vi "Elevator.vi"() -> ()   [LabVIEW 2018]
uses:
  Elevator Cabin.ctl
  Floors Schematic.ctl
  Elevator Panel.ctl
  Elevator Automate.ctl
  Elevator Command.ctl
  Elevator Constants.ctl
panel:
  out "Delay Timer":i32
  out "Passenger Information Board":string="Этаж 1\r\nОстановка"
  out "# elements in Elevator Command Queue":i32
  out "Global Wait in ms":u32=10
  out "# elements in Elevator Floor Queue":i32
  out "Position:Top":i32=585
  out "Elevator Floor Queue":u8[](array[numeric])
  out "Elevator Command Queue":T1[](array[typedef])
  in  "Elevator Automate":T2={"Elevator Panel Array"=[FALSE, FALSE, FALSE, FALSE, FALSE, FALSE, FALSE, FALSE, FALSE, FALSE, FALSE, FALSE], "Floor Array"=[FALSE, FALSE, FALSE, FALSE, FALSE, FALSE, FALSE, FALSE, FALSE, FALSE, FALSE, FALSE], "Elevator Command"=enum."Open Doors", "Target Floor"=0, "Forced Stop"=FALSE, "Cancel Delay"=FALSE, "Elevator Status"=enum."Stand By", "Update\nTarget Floor"=FALSE, "Take a Call"=FALSE, "Add Floor\nto Queue"=FALSE}
  in  "Elevator Panel":T3
  in  "Floors Schematic":T4={"Call 1"=FALSE, "Call 2"=FALSE, "Call 3"=FALSE, "Call 4"=FALSE, "Call 5"=FALSE, "Call 6"=FALSE, "Call 7"=FALSE, "Call 8"=FALSE, "Call 9"=FALSE, "Call 10"=FALSE, "Call 11"=FALSE, "Call 12"=FALSE, "Floor Position"=[0, 0, 0, 0, 0, 0, 0, 0, 0, 0, 0, 0]}
  in  "STOP":bool
  out "Elevator Cabin":T5 scale=0.0..100.0
  # "Краткая информация об автомате лифта\n\nЕсть две очереди: очередь команд лифта (Elevator Command Queue) и очередь вызовов этажей лифта (Elevator Floor Queue).\n\nАвтомат при вызове этажа обрабатывает и перестраивает очередь с учетом приоритета вызовов.\n\nАвтомат принимает решения исходя из этажа-цели (Target Floor), текущей выполняющейся команды (Elevator Command) и статуса состояния лифта (Elevator Status).\n\nАвтомат имеет хранилище вызовов этажей из кабины лифта (Elevator Panel Array) и вызовов с этажей дома (Floor Array).\n\nКоманды Elevator Command:\n1) Idle - команда ожидания;\n2) Short Delay - короткая задержка (2 сек);\n3) Long Delay - длинная задержка (6 сек);\n4) Cancel Delay - задержка в случае отмены вызова и принятия решений обработки следующего вызова (6 сек или 15 сек в зависимости от состояний автомата лифта);\n5) Open Doors - открыть двери кабины лифта;\n6) Close Doors - закрыть двери кабины лифта;\n7) Going Up - движение вверх к этажу-цели;\n8) Going Down - движение вниз к этажу-цели;\n9) Unpress Button отжать кнопки на этаже-цели.\n\nСостояния Elevator Status:\n1) Stand By - состояние остановки кабины лифта и ожидания вызова;\n2) Stop - состояние остановки кабины лифта при движении вверх или вниз;\n3) Going Up - состояние движения вверх к этажу-цели;\n4) Going Down - состояние движения вниз к этажу-цели;\n5) Cancel - состояние отмены текущих вызовов панели кабины лифта.\n\nКнопки Автомата для обработки событий:\n1) Take a Call - обработать следующий вызов из очереди;\n2) Add Floor to Queue - добавить этаж в очередь вызовов;\n3) Update Target Floor - обновить этаж-цель;\n4) Forced Stop - прерывание исполняемой команды лифта;\n5) Cancel Delay - обработка события отмены вызовов панели кабины лифта."
  # "Симулятор работы лифта в двенадцатиэтажном доме\n\nВ симуляторе имеются:\n1) кнопки вызова (1-12) на этажах дома (Floors Schematic);\n2) кнопки вызова (1-12) панели кабины лифта (Elevator Panel);\n3) кнопка отмены всех вызовов панели кабины лифта (Cancel);\n4) кнопка вызова оператора (Emergency);\n5) кнопка закрытия дверей (>||<);\n6) кнопка открытия дверей (<||>);\n7) Информационное табло лифта (Passenger Information Board).\n\nКнопки вызова на этажах дома являются вызовом по направлению движения кабины лифта вниз.\n\nПриоритет этажей построен так, чтобы обработать максимально возможное количество вызовов при заданном направлении движения кабины лифта.\n\nОчередь вызовов выстраивается с учетом направления движения кабины лифта, вызова на этаж из кабины лифта и вызова на этаж дома (приведено в поряжке убывания приоритета).\n\nНачальное состояние работы симулятора:\nкабина лифта на первом этаже, двери кабины лифта закрыты, все кнопки вызова отжаты.\n\nТабло лифта приводит информацию о текущем этаже, статусе движения кабины лифта (движение вверх, движение вниз, остановка), а также сигнализирует о работе кнопки вызова оператора.\n\nЕсли лифт приезжает на обработанный с учетом очереди этаж-цель (Targer Floor), кнопка вызова этажа-цели отжимаются как в кабине лифта, так и на этаже дома.\n\nДвери кабины лифта не откроются при движении лифта вверх или вниз. Лифт открывает двери повторно, если двери кабины лифта не закрыты на этаже-цели. Лифт не закроет двери, пока не закончится открытие дверей."
  # "12"
  # "11"
  # "10"
  # "9"
  # "8"
  # "7"
  # "6"
  # "5"
  # "4"
  # "3"
  # "2"
  # "1"
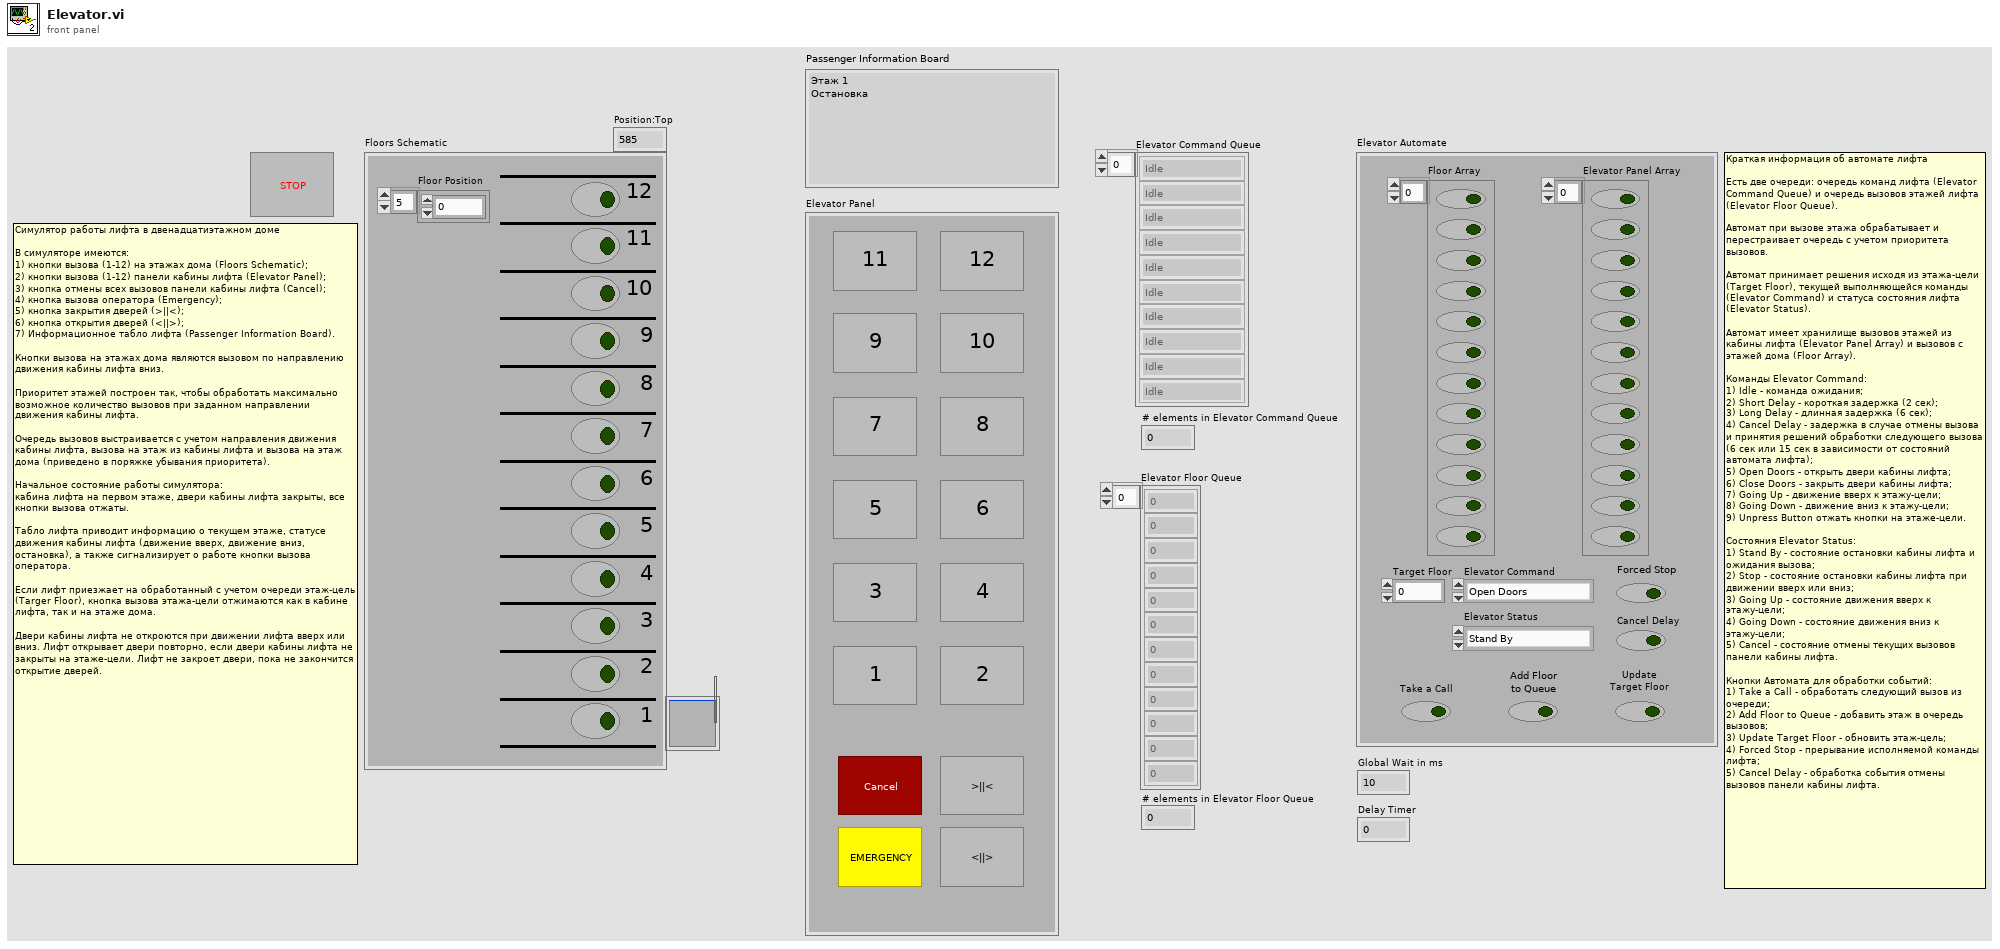
[diagram p1: front panel]
types:
  T1 = typedef "Elevator Command.ctl" = enum16{"Idle", "Short Delay", "Long Delay", "Cancel Delay", "Open Doors", "Close Doors", "Going Up", "Going Down", "Unpress Button"}
  T2 = typedef "Elevator Automate.ctl" = cluster{"Elevator Panel Array":bool[], "Floor Array":bool[], "Elevator Command":T1, "Target Floor":u8, "Forced Stop":bool, "Cancel Delay":bool, "Elevator Status":enum16{"Stand By", "Stop", "Going Up", "Going Down", "Cancel"}, "Update\nTarget Floor":bool, "Take a Call":bool, "Add Floor\nto Queue":bool}
  T3 = typedef "Elevator Panel.ctl" = cluster{"Open Doors":bool, "Close Doors":bool, "Floor 2":bool, "Floor 1":bool, "Floor 3":bool, "Floor 4":bool, "Floor 5":bool, "Floor 6":bool, "Floor 7":bool, "Floor 8":bool, "Floor 9":bool, "Floor 10":bool, "Floor 11":bool, "Floor 12":bool, "Emergency":bool, "Cancel":bool}
  T4 = typedef "Floors Schematic.ctl" = cluster{"Call 1":bool, "Call 2":bool, "Call 3":bool, "Call 4":bool, "Call 5":bool, "Call 6":bool, "Call 7":bool, "Call 8":bool, "Call 9":bool, "Call 10":bool, "Call 11":bool, "Call 12":bool, "Floor Position":i16[]}
  T5 = typedef "Elevator Cabin.ctl" = u8
  T6 = enum16{"Stand By", "Stop", "Going Up", "Going Down", "Cancel"}
  T7 = enum8{"Enabled", "Disabled", "Disabled and Grayed Out"}
  T8 = typedef "Elevator Constants.ctl" = u8
  T9 = enum16{"Stand By", "Stop", "Going Up", "Going Down"}
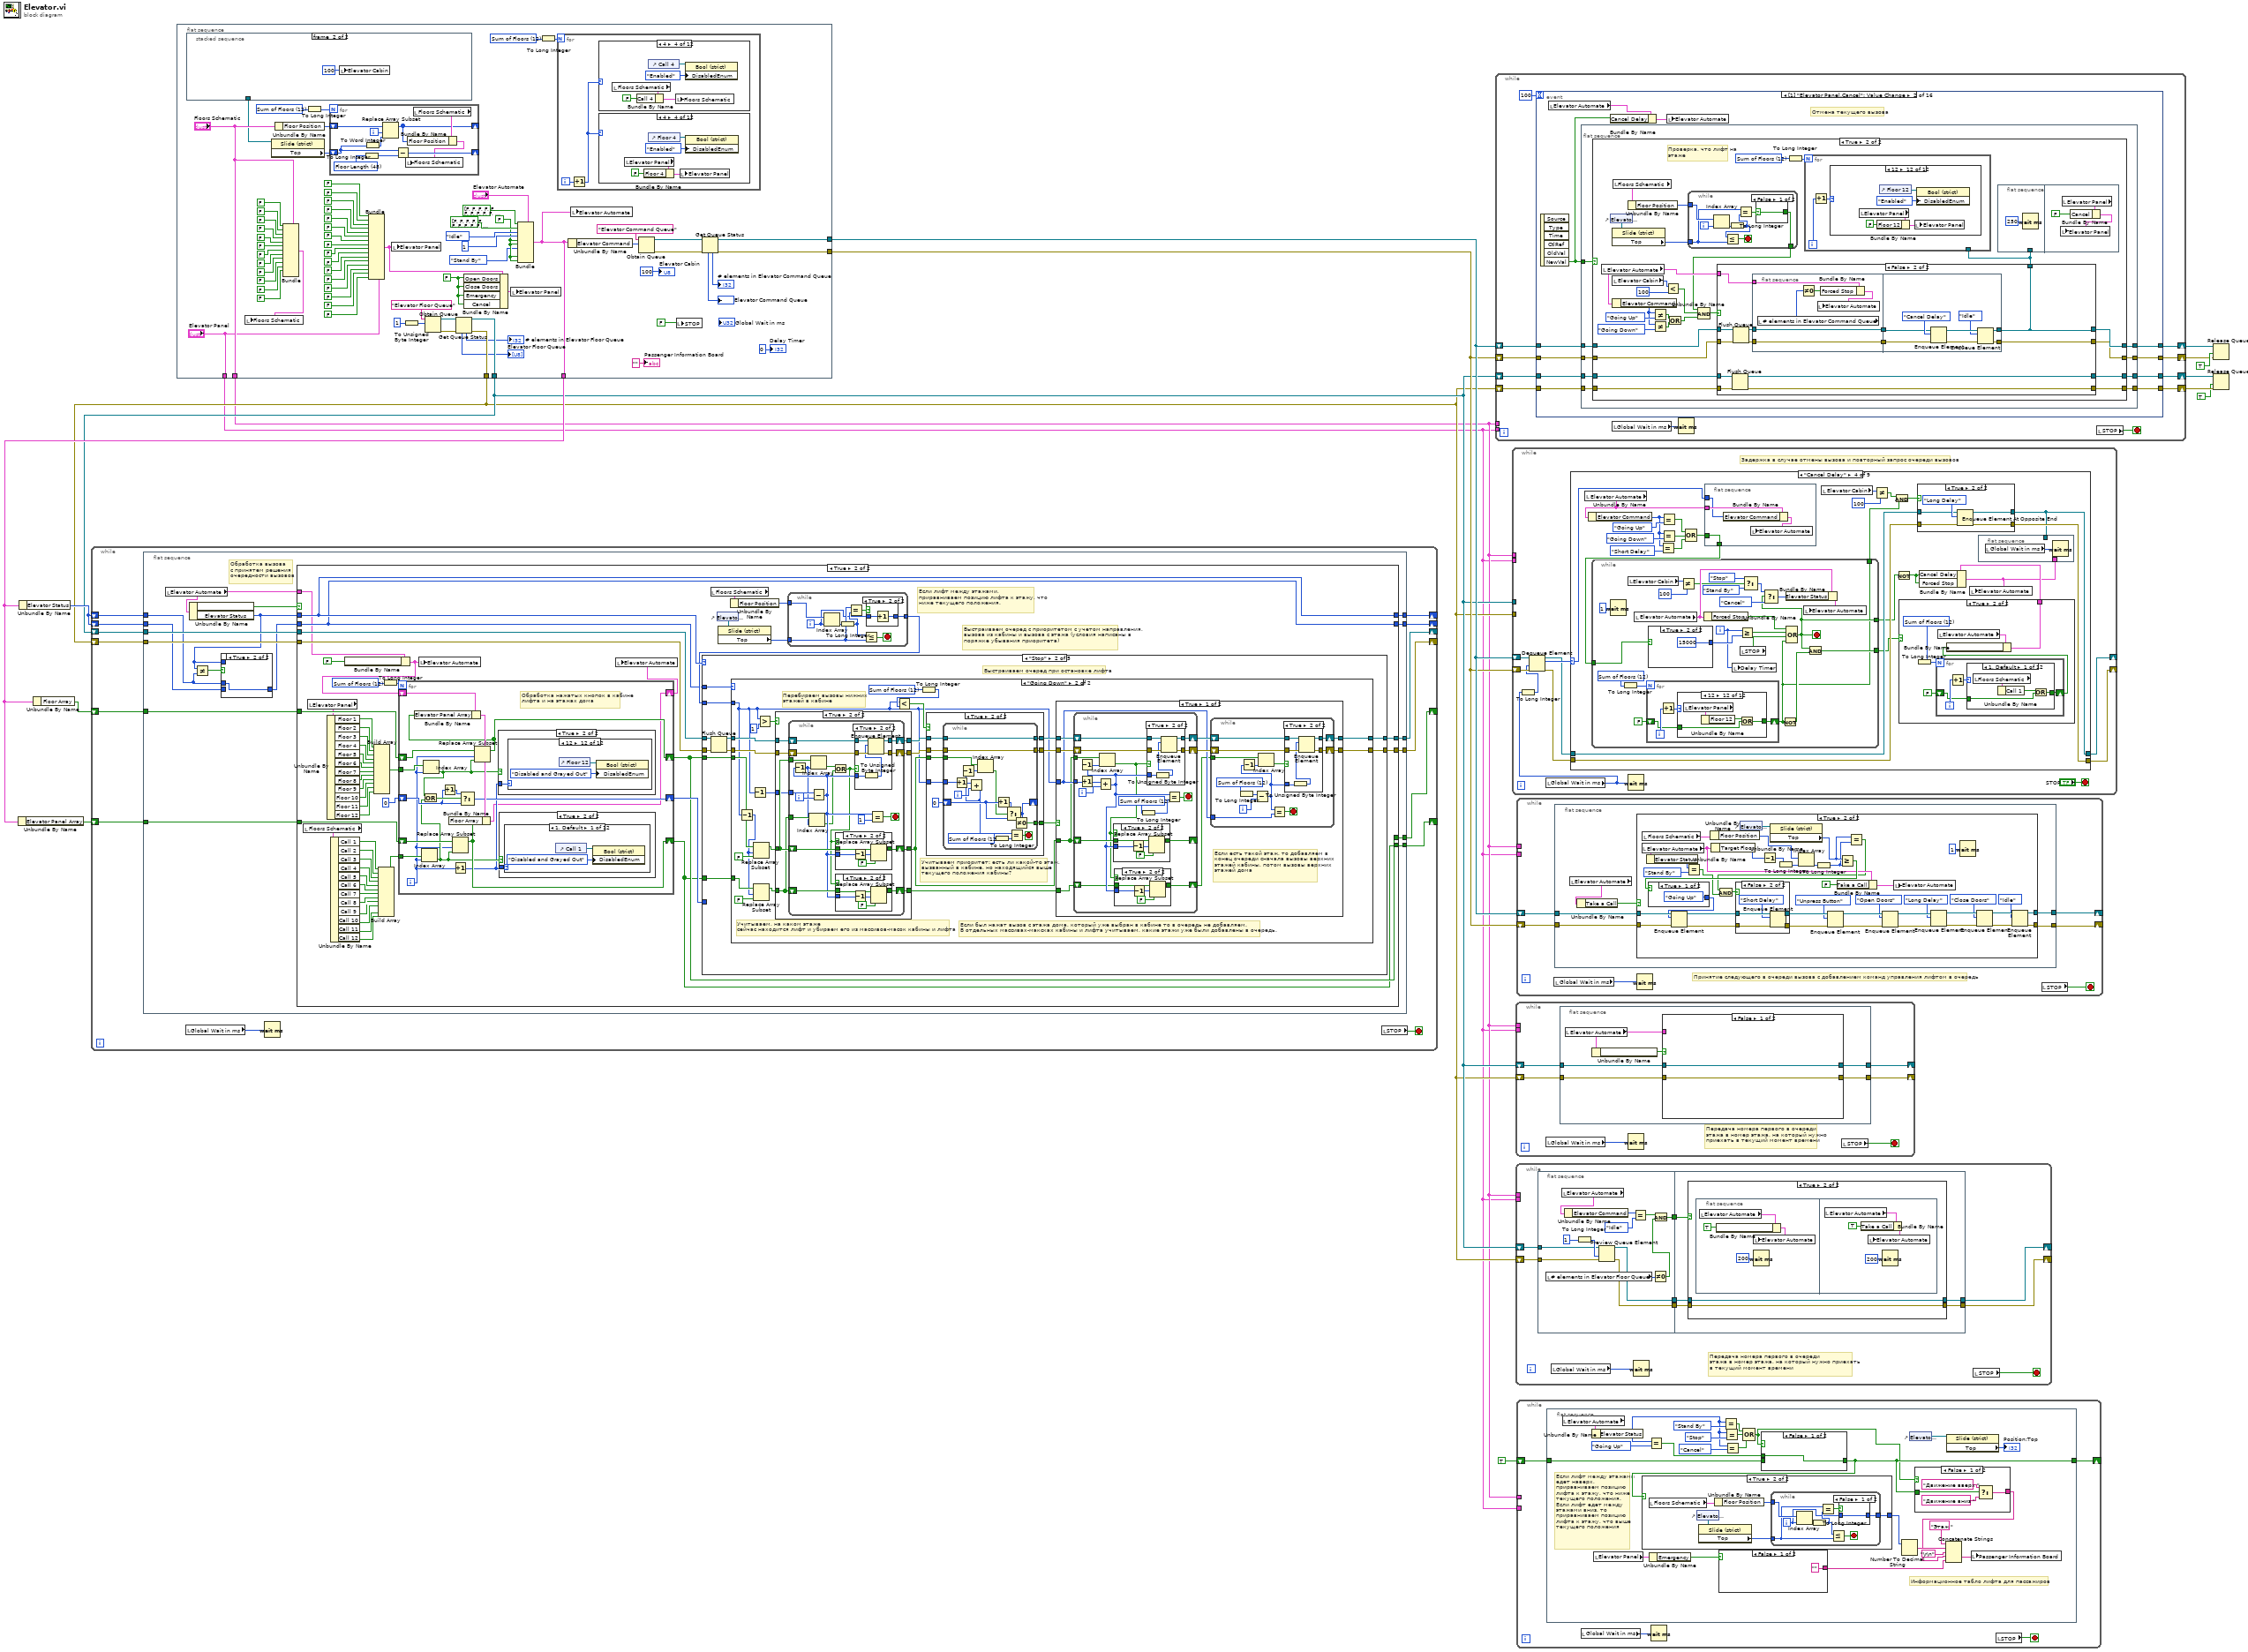
[diagram p0: block diagram]
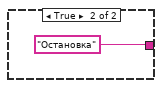
[diagram p2: hidden frame]
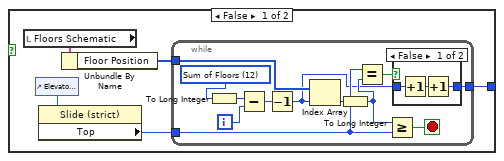
[diagram p4: hidden frame]
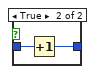
[diagram p5: hidden frame]
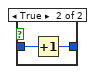
[diagram p6: hidden frame]
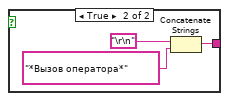
[diagram p7: hidden frame]
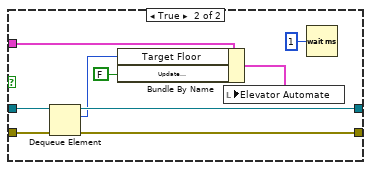
[diagram p9: hidden frame]
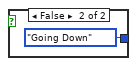
[diagram p12: hidden frame]
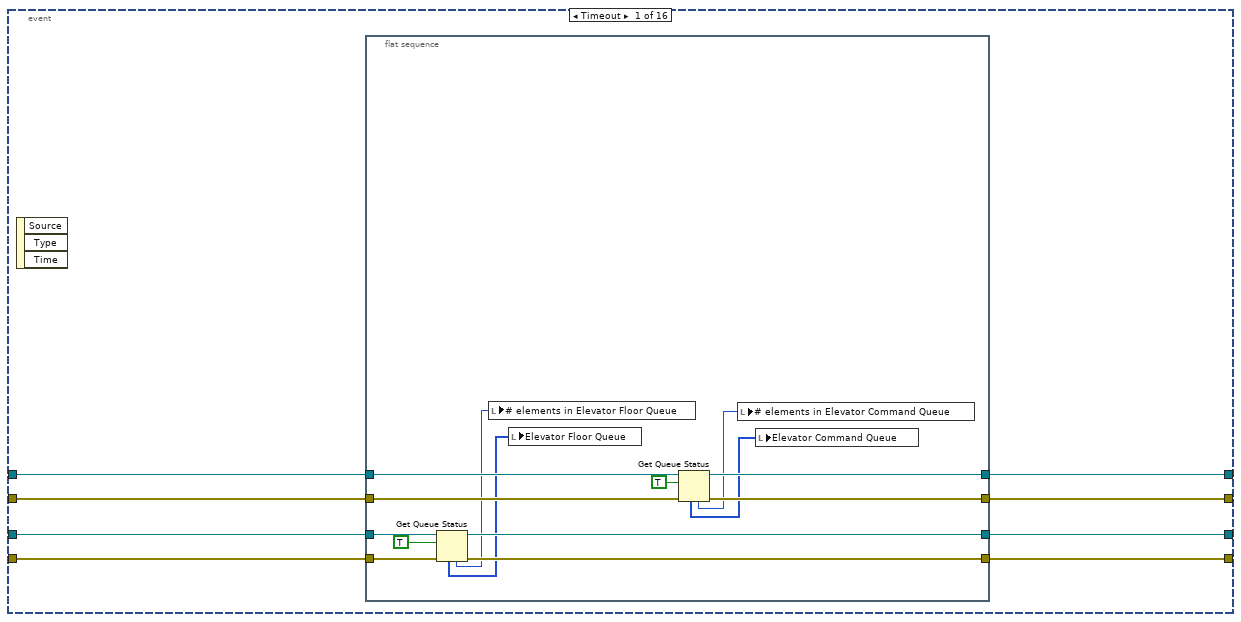
[diagram p13: hidden frame]
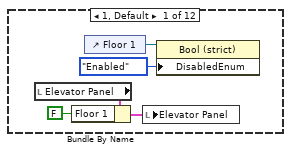
[diagram p15: hidden frame]
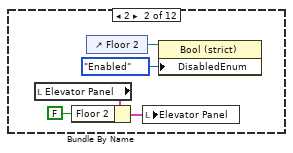
[diagram p16: hidden frame]
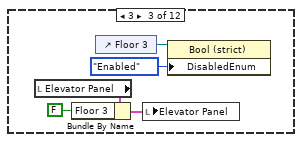
[diagram p17: hidden frame]
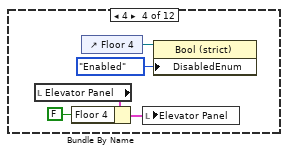
[diagram p18: hidden frame]
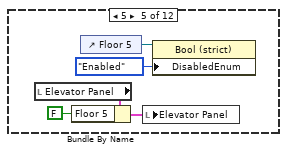
[diagram p19: hidden frame]
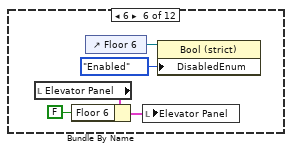
[diagram p20: hidden frame]
diagram:
  n1 = Unbundle By Name(w9) -> ("Elevator Panel Array"=w16:bool[])
  n2 = Unbundle By Name(w9) -> ("Elevator Status"=w8:T6)
  n3 = Unbundle By Name(w9) -> ("Floor Array"=w17:bool[])
  n4 = while {
    shift-right: [w26] -> _
    shift-left: w16 -> [w29]
    shift-right: [w25] -> _
    shift-left: w17 -> [w30]
    shift-right: [w23] -> _
    shift-left: w4 -> [w28]
    shift-right: [w24] -> _
    shift-left: w5 -> [w27]
    shift-right: [w22] -> _
    shift-left: w8 -> [w19]
    shift-right: [w20] -> _
    shift-left: w8 -> [w21]
    stop <- w31 stop-if-true
    n5 = flat-sequence {
      tunnel: [w43] -> w26
      tunnel: [w42] -> w25
      tunnel: [w41] -> w24
      tunnel: [w40] -> w23
      tunnel: [w39] -> w22
      tunnel: [w34] -> w20
      tunnel: w30 -> [w48]
      tunnel: w29 -> [w47]
      tunnel: w28 -> [w46]
      tunnel: w27 -> [w45]
      tunnel: w21 -> [w36]
      tunnel: w19 -> [w33]
      frame #0 {
        # "Обработка вызова\nс принятем решения\nочередности вызовов"
        n6 = local read "Elevator Automate"() -> (w38:T2)
        n7 = Unbundle By Name(w38) -> ("Add Floor\nto Queue"=w44:bool, "Elevator Status"=w35:T6)
        n8 = Not Equal?(x=w35, y=w36) -> (x != y?=w37:bool)
        n9 = case shown="True" w37 {
          tunnel: w35 -> [_ _]
          tunnel: w36 -> [_ w50]
          tunnel: w33 -> [w49 _]
          tunnel: [w49 w50] -> w32
          frame False {
          }
          frame True {
          }
        }
        n10 = case shown="True" w44 {
          tunnel: w48 -> [w53 w107]
          tunnel: w47 -> [w54 w106]
          tunnel: w46 -> [w55 w75]
          tunnel: w45 -> [w56 w74]
          tunnel: w35 -> [w52 w70]
          tunnel: [w56 w72] -> w41
          tunnel: [w55 w71] -> w40
          tunnel: [w54 w65] -> w43
          tunnel: [w53 w66] -> w42
          tunnel: w32 -> [w51 w64]
          tunnel: [w51 w64] -> w39
          tunnel: w38 -> [_ w59]
          tunnel: [w52 w70] -> w34
          frame False {
          }
          frame True {
            w77 = T8 12 items=["Floor Length"=48, "Sum of Floors"=12, "Floor Step in ms"=63, "Elevator Door Step in ms"=30, "Global Wait in ms"=20, "Event Wait in ms"=100] ("Elevator Constants")
            # "Выстраиваем очеред с приоритетом с учетом направления, вызова из кабины и вызова с этажа (условия написаны в поряжке убывания приоритета)"
            # "Если лифт между этажами,\nприравниваем позицию лифта к этажу, что ниже текущего положения."
            n11 = local read "Floors Schematic"() -> (w78:T4)
            n12 = local read "Elevator Panel"() -> (w79:T3)
            n13 = Unbundle By Name(w79) -> ("Floor 1"=w105:bool, "Floor 2"=w104:bool, "Floor 3"=w103:bool, "Floor 4"=w102:bool, "Floor 5"=w101:bool, "Floor 6"=w100:bool, "Floor 7"=w99:bool, "Floor 8"=w98:bool, "Floor 9"=w97:bool, "Floor 10"=w96:bool, "Floor 11"=w95:bool, "Floor 12"=w94:bool)
            n14 = Unbundle By Name(w78) -> ("Call 1"=w80:bool, "Call 2"=w92:bool, "Call 3"=w91:bool, "Call 4"=w90:bool, "Call 5"=w89:bool, "Call 6"=w88:bool, "Call 7"=w87:bool, "Call 8"=w86:bool, "Call 9"=w85:bool, "Call 10"=w84:bool, "Call 11"=w83:bool, "Call 12"=w82:bool)
            n15 = Bundle By Name(cluster=w59, "Add Floor\nto Queue"=FALSE ("Add Floor to Queue")) -> (w58:T2)
            n16 = Build Array(w105, w104, w103, w102, w101, w100, w99, w98, w97, w96, w95, w94) -> (w93:bool[])
            n17 = Build Array(w80, w92, w91, w90, w89, w88, w87, w86, w85, w84, w83, w82) -> (w81:bool[])
            n18 = To Long Integer(number=w77) -> (32bit integer=w76:i32)
            n19 = for {
              N: w76 -> [_]
              tunnel: w93 -> [w1124]
              tunnel: w81 -> [w1123]
              shift-right: [w1114] -> w65
              shift-left: w106 -> [w1120]
              shift-right: [w1115] -> w66
              shift-left: w107 -> [w1121]
              shift-right: [w1117] -> w69
              shift-left: 0 -> [w1116]
              shift-right: [w1108] -> w57
              shift-left: w58 -> [w1109]
              i -> [w1111]
              # "Обработка нажатых кнопок в кабине лифта и на этажах дома"
              n20 = Index Array(array=w1123, index=w1111) -> (element=w1113:bool)
              n21 = Index Array(array=w1124, index=w1111) -> (element=w1112:bool)
              n22 = Or(x=w1112, y=w1113) -> (x .or. y?=w1119:bool)
              n23 = Increment(x=w1116) -> (x+1=w1118:i32)
              n24 = Replace Array Subset(array=w1120, new element=w1113, index=w1111) -> (w1114:bool[])
              n25 = Increment(x=w1111) -> (x+1=w1110:i32)
              n26 = Select(t=w1118, s=w1119, f=w1116) -> (s? t:f=w1117:i32)
              n27 = Replace Array Subset(array=w1121, new element=w1112, index=w1111) -> (w1115:bool[])
              n28 = Bundle By Name(cluster=w1109, "Elevator Panel Array"=w1115) -> (w1122:T2)
              n29 = Bundle By Name(cluster=w1122, "Floor Array"=w1114) -> (w1108:T2)
              n30 = case shown="True" w1112 {
                tunnel: w1110 -> [_ w1150]
                frame False {
                }
                frame True {
                  n31 = case shown="12" w1150 {
                    frame 1, Default {
                      n32 = control-ref of="Floor 1"() -> (w1152:refnum<vi>)
                      n33 = property class="Bool (strict)"(reference=w1152, "DisabledEnum"=T7."Disabled and Grayed Out" ("Disabled")) -> ()  [unwired: 1 in, 2 out]
                    }
                    frame 2 {
                      n34 = control-ref of="Floor 2"() -> (w1154:refnum<vi>)
                      n35 = property class="Bool (strict)"(reference=w1154, "DisabledEnum"=T7."Disabled and Grayed Out" ("Disabled")) -> ()  [unwired: 1 in, 2 out]
                    }
                    frame 3 {
                      n36 = control-ref of="Floor 3"() -> (w1156:refnum<vi>)
                      n37 = property class="Bool (strict)"(reference=w1156, "DisabledEnum"=T7."Disabled and Grayed Out" ("Disabled")) -> ()  [unwired: 1 in, 2 out]
                    }
                    frame 4 {
                      n38 = control-ref of="Floor 4"() -> (w1158:refnum<vi>)
                      n39 = property class="Bool (strict)"(reference=w1158, "DisabledEnum"=T7."Disabled and Grayed Out" ("Disabled")) -> ()  [unwired: 1 in, 2 out]
                    }
                    frame 5 {
                      n40 = control-ref of="Floor 5"() -> (w1160:refnum<vi>)
                      n41 = property class="Bool (strict)"(reference=w1160, "DisabledEnum"=T7."Disabled and Grayed Out" ("Disabled")) -> ()  [unwired: 1 in, 2 out]
                    }
                    frame 6 {
                      n42 = control-ref of="Floor 6"() -> (w1162:refnum<vi>)
                      n43 = property class="Bool (strict)"(reference=w1162, "DisabledEnum"=T7."Disabled and Grayed Out" ("Disabled")) -> ()  [unwired: 1 in, 2 out]
                    }
                    frame 7 {
                      n44 = control-ref of="Floor 7"() -> (w1164:refnum<vi>)
                      n45 = property class="Bool (strict)"(reference=w1164, "DisabledEnum"=T7."Disabled and Grayed Out" ("Disabled")) -> ()  [unwired: 1 in, 2 out]
                    }
                    frame 8 {
                      n46 = control-ref of="Floor 8"() -> (w1166:refnum<vi>)
                      n47 = property class="Bool (strict)"(reference=w1166, "DisabledEnum"=T7."Disabled and Grayed Out" ("Disabled")) -> ()  [unwired: 1 in, 2 out]
                    }
                    frame 9 {
                      n48 = control-ref of="Floor 9"() -> (w1168:refnum<vi>)
                      n49 = property class="Bool (strict)"(reference=w1168, "DisabledEnum"=T7."Disabled and Grayed Out" ("Disabled")) -> ()  [unwired: 1 in, 2 out]
                    }
                    frame 10 {
                      n50 = control-ref of="Floor 10"() -> (w1170:refnum<vi>)
                      n51 = property class="Bool (strict)"(reference=w1170, "DisabledEnum"=T7."Disabled and Grayed Out" ("Disabled")) -> ()  [unwired: 1 in, 2 out]
                    }
                    frame 11 {
                      n52 = control-ref of="Floor 11"() -> (w1172:refnum<vi>)
                      n53 = property class="Bool (strict)"(reference=w1172, "DisabledEnum"=T7."Disabled and Grayed Out" ("Disabled")) -> ()  [unwired: 1 in, 2 out]
                    }
                    frame 12 {
                      n54 = control-ref of="Floor 12"() -> (w1174:refnum<vi>)
                      n55 = property class="Bool (strict)"(reference=w1174, "DisabledEnum"=T7."Disabled and Grayed Out" ("Disabled")) -> ()  [unwired: 1 in, 2 out]
                    }
                  }
                }
              }
              n56 = case shown="True" w1113 {
                tunnel: w1110 -> [_ w1125]
                frame False {
                }
                frame True {
                  n57 = case shown="1, Default" w1125 {
                    frame 1, Default {
                      n58 = control-ref of="Call 1"() -> (w1127:refnum<vi>)
                      n59 = property class="Bool (strict)"(reference=w1127, "DisabledEnum"=T7."Disabled and Grayed Out" ("Disabled")) -> ()  [unwired: 1 in, 2 out]
                    }
                    frame 2 {
                      n60 = control-ref of="Call 2"() -> (w1129:refnum<vi>)
                      n61 = property class="Bool (strict)"(reference=w1129, "DisabledEnum"=T7."Disabled and Grayed Out" ("Disabled")) -> ()  [unwired: 1 in, 2 out]
                    }
                    frame 3 {
                      n62 = control-ref of="Call 3"() -> (w1131:refnum<vi>)
                      n63 = property class="Bool (strict)"(reference=w1131, "DisabledEnum"=T7."Disabled and Grayed Out" ("Disabled")) -> ()  [unwired: 1 in, 2 out]
                    }
                    frame 4 {
                      n64 = control-ref of="Call 4"() -> (w1133:refnum<vi>)
                      n65 = property class="Bool (strict)"(reference=w1133, "DisabledEnum"=T7."Disabled and Grayed Out" ("Disabled")) -> ()  [unwired: 1 in, 2 out]
                    }
                    frame 5 {
                      n66 = control-ref of="Call 5"() -> (w1135:refnum<vi>)
                      n67 = property class="Bool (strict)"(reference=w1135, "DisabledEnum"=T7."Disabled and Grayed Out" ("Disabled")) -> ()  [unwired: 1 in, 2 out]
                    }
                    frame 6 {
                      n68 = control-ref of="Call 6"() -> (w1137:refnum<vi>)
                      n69 = property class="Bool (strict)"(reference=w1137, "DisabledEnum"=T7."Disabled and Grayed Out" ("Disabled")) -> ()  [unwired: 1 in, 2 out]
                    }
                    frame 7 {
                      n70 = control-ref of="Call 7"() -> (w1139:refnum<vi>)
                      n71 = property class="Bool (strict)"(reference=w1139, "DisabledEnum"=T7."Disabled and Grayed Out" ("Disabled")) -> ()  [unwired: 1 in, 2 out]
                    }
                    frame 8 {
                      n72 = control-ref of="Call 8"() -> (w1141:refnum<vi>)
                      n73 = property class="Bool (strict)"(reference=w1141, "DisabledEnum"=T7."Disabled and Grayed Out" ("Disabled")) -> ()  [unwired: 1 in, 2 out]
                    }
                    frame 9 {
                      n74 = control-ref of="Call 9"() -> (w1143:refnum<vi>)
                      n75 = property class="Bool (strict)"(reference=w1143, "DisabledEnum"=T7."Disabled and Grayed Out" ("Disabled")) -> ()  [unwired: 1 in, 2 out]
                    }
                    frame 10 {
                      n76 = control-ref of="Call 10"() -> (w1145:refnum<vi>)
                      n77 = property class="Bool (strict)"(reference=w1145, "DisabledEnum"=T7."Disabled and Grayed Out" ("Disabled")) -> ()  [unwired: 1 in, 2 out]
                    }
                    frame 11 {
                      n78 = control-ref of="Call 11"() -> (w1147:refnum<vi>)
                      n79 = property class="Bool (strict)"(reference=w1147, "DisabledEnum"=T7."Disabled and Grayed Out" ("Disabled")) -> ()  [unwired: 1 in, 2 out]
                    }
                    frame 12 {
                      n80 = control-ref of="Call 12"() -> (w1149:refnum<vi>)
                      n81 = property class="Bool (strict)"(reference=w1149, "DisabledEnum"=T7."Disabled and Grayed Out" ("Disabled")) -> ()  [unwired: 1 in, 2 out]
                    }
                  }
                }
              }
            }
            n82 = local write "Elevator Automate"(w58) -> ()
            n83 = local write "Elevator Automate"(w57) -> ()
            n84 = local read "Floors Schematic"() -> (w62:T4)
            n85 = control-ref of="Elevator Cabin"() -> (w63:refnum<vi>)
            n86 = property class="Slide (strict)"(reference=w63) -> ("Top"=w60:i32)  [unwired: 1 in, 2 out]
            n87 = Unbundle By Name(w62) -> ("Floor Position"=w61:i16[])
            n88 = while {
              tunnel: w61 -> [w113]
              tunnel: w60 -> [w111]
              tunnel: [w110] -> w68
              i -> [w108]
              stop <- w109 stop-if-true
              n89 = Index Array(array=w113, index=w108) -> (element=w114:i16)
              n90 = To Long Integer(number=w114) -> (32bit integer=w112:i32)
              n91 = Equal?(x=w111, y=w112) -> (x = y?=w115:bool)
              n92 = Less Or Equal?(x=w112, y=w111) -> (x <= y?=w109:bool)
              n93 = case shown="True" w115 {
                tunnel: w108 -> [w116 w118]
                tunnel: [w116 w117] -> w110
                frame False {
                }
                frame True {
                  n94 = Increment(x=w118) -> (x+1=w117:i32)
                }
              }
            }
            n95 = case shown="\"Stop\"" w70 {
              tunnel: w74 -> [w137 w258 w691 w887 w1107]
              tunnel: w75 -> [w136 w259 w692 w888 w1106]
              tunnel: w66 -> [w127 w263 w679 w890 _]
              tunnel: w65 -> [w125 w261 w680 w889 _]
              tunnel: w68 -> [w126 w262 w676 w868 _]
              tunnel: [w129 w265 w694 w892 w1107] -> w72
              tunnel: [w128 w264 w693 w891 w1106] -> w71
              tunnel: w64 -> [_ w260 _ _ _]
              tunnel: w69 -> [w122 _ _ _ _]
              frame "Stand By", Default {
                # "Перебираем вызовы на нижних этажах"
                # "Перебираем вызовы на верхних этажах"
                # "Если было одновременно несколько вызовов (например в Elevator Status = Cancel), то повторно обрабатываем\nочередь с учетом направления движения лифта"
                # "Перебираем вызовы верхних этажей в кабине"
                # "Перебираем вызовы нижних этажей в кабине"
                # "Выбираем приоритетный вызов в режиме ожидания"
                n96 = while {
                  tunnel: w127 -> [w215]
                  shift-right: [w212] -> w133
                  shift-left: w137 -> [w214]
                  shift-right: [w213] -> w132
                  shift-left: w136 -> [w216]
                  tunnel: w126 -> [w204]
                  tunnel: [w207] -> w131
                  i -> [w203]
                  stop <- w211 stop-if-true
                  w209 = T8 12 items=["Floor Length"=48, "Sum of Floors"=12, "Floor Step in ms"=63, "Elevator Door Step in ms"=30, "Global Wait in ms"=20, "Event Wait in ms"=100] ("Elevator Constants")
                  n97 = Add(x=w204, y=w203) -> (x+y=w205:i32)
                  n98 = Decrement(x=w205) -> (x-1=w206:i32)
                  n99 = Index Array(array=w215, index=w206) -> (element=w207:bool)
                  n100 = To Long Integer(number=w209) -> (32bit integer=w210:i32)
                  n101 = case shown="True" w207 {
                    tunnel: w214 -> [w218 w224]
                    tunnel: w216 -> [w217 w223]
                    tunnel: [w217 w222] -> w213
                    tunnel: [w218 w221] -> w212
                    tunnel: w205 -> [_ w220]
                    frame False {
                    }
                    frame True {
                      n102 = To Unsigned Byte Integer(number=w220) -> (unsigned 8bit integer=w219:u8)
                      n103 = Enqueue Element(queue=w224, element=w219, error in (no error)=w223) -> (queue out=w221:refnum<queue>, error out=w222:errorcluster)  [unwired: 1 in, 1 out]
                    }
                  }
                  n104 = Equal?(x=w205, y=w210) -> (x = y?=w208:bool)
                  n105 = Or(x=w207, y=w208) -> (x .or. y?=w211:bool)
                }
                n106 = Greater?(x=w122, y=1) -> (0:w124:bool)
                n107 = case shown="True" w124 {
                  frame True {
                    n108 = flat-sequence {
                      frame #0 {
                        n109 = Wait (ms)(milliseconds to wait=u32 300) -> ()  [unwired: 1 out]
                      }
                      frame #1 {
                        n110 = local read "Elevator Automate"() -> (w202:T2)
                        n111 = Bundle By Name(cluster=w202, "Add Floor\nto Queue"=TRUE ("Add Floor to Queue")) -> (w200:T2)
                        n112 = local write "Elevator Automate"(w200) -> ()
                      }
                    }
                  }
                  frame False {
                  }
                }
                n113 = case shown="False" w131 {
                  selector: w131 -> [w227 _]
                  tunnel: w132 -> [w225 w234]
                  tunnel: w133 -> [w226 w233]
                  tunnel: w126 -> [_ w232]
                  tunnel: w127 -> [_ w231]
                  tunnel: [w227 w230] -> w130
                  tunnel: [w226 w229] -> w135
                  tunnel: [w225 w228] -> w134
                  frame True {
                  }
                  frame False {
                    n114 = while {
                      tunnel: w231 -> [w246]
                      shift-right: [w243] -> w229
                      shift-left: w233 -> [w245]
                      shift-right: [w244] -> w228
                      shift-left: w234 -> [w247]
                      tunnel: w232 -> [w238]
                      tunnel: [w240] -> w230
                      i -> [w237]
                      stop <- w242 stop-if-true
                      n115 = Subtract(x=w238, y=w237) -> (x-y=w235:i32)
                      n116 = Decrement(x=w235) -> (x-1=w236:i32)
                      n117 = Index Array(array=w246, index=w236) -> (element=w240:bool)
                      n118 = case shown="True" w240 {
                        tunnel: w245 -> [w249 w255]
                        tunnel: w247 -> [w248 w254]
                        tunnel: [w248 w253] -> w244
                        tunnel: [w249 w252] -> w243
                        tunnel: w235 -> [_ w251]
                        frame False {
                        }
                        frame True {
                          n119 = To Unsigned Byte Integer(number=w251) -> (unsigned 8bit integer=w250:u8)
                          n120 = Enqueue Element(queue=w255, element=w250, error in (no error)=w254) -> (queue out=w252:refnum<queue>, error out=w253:errorcluster)  [unwired: 1 in, 1 out]
                        }
                      }
                      n121 = Equal?(x=w235, y=1) -> (x = y?=w241:bool)
                      n122 = Or(x=w240, y=w241) -> (x .or. y?=w242:bool)
                    }
                  }
                }
                n123 = case shown="False" w130 {
                  selector: w130 -> [w169 _]
                  tunnel: w134 -> [w167 w176]
                  tunnel: w135 -> [w168 w175]
                  tunnel: w126 -> [_ w174]
                  tunnel: w125 -> [_ w173]
                  tunnel: [w169 w172] -> w119
                  tunnel: [w168 w171] -> w121
                  tunnel: [w167 w170] -> w120
                  frame True {
                  }
                  frame False {
                    n124 = while {
                      tunnel: w173 -> [w189]
                      shift-right: [w186] -> w171
                      shift-left: w175 -> [w188]
                      shift-right: [w187] -> w170
                      shift-left: w176 -> [w190]
                      tunnel: w174 -> [w180]
                      tunnel: [w181] -> w172
                      i -> [w179]
                      stop <- w185 stop-if-true
                      w183 = T8 12 items=["Floor Length"=48, "Sum of Floors"=12, "Floor Step in ms"=63, "Elevator Door Step in ms"=30, "Global Wait in ms"=20, "Event Wait in ms"=100] ("Elevator Constants")
                      n125 = Add(x=w180, y=w179) -> (x+y=w178:i32)
                      n126 = Decrement(x=w178) -> (x-1=w177:i32)
                      n127 = Index Array(array=w189, index=w177) -> (element=w181:bool)
                      n128 = To Long Integer(number=w183) -> (32bit integer=w184:i32)
                      n129 = case shown="True" w181 {
                        tunnel: w188 -> [w192 w198]
                        tunnel: w190 -> [w191 w197]
                        tunnel: [w191 w196] -> w187
                        tunnel: [w192 w195] -> w186
                        tunnel: w178 -> [_ w194]
                        frame False {
                        }
                        frame True {
                          n130 = To Unsigned Byte Integer(number=w194) -> (unsigned 8bit integer=w193:u8)
                          n131 = Enqueue Element(queue=w198, element=w193, error in (no error)=w197) -> (queue out=w195:refnum<queue>, error out=w196:errorcluster)  [unwired: 1 in, 1 out]
                        }
                      }
                      n132 = Equal?(x=w178, y=w184) -> (x = y?=w182:bool)
                      n133 = Or(x=w181, y=w182) -> (x .or. y?=w185:bool)
                    }
                  }
                }
                n134 = case shown="False" w119 {
                  tunnel: w120 -> [w138 w145]
                  tunnel: w121 -> [w139 w144]
                  tunnel: w125 -> [_ w143]
                  tunnel: [w139 w142] -> w129
                  tunnel: [w138 w141] -> w128
                  tunnel: w126 -> [_ w140]
                  frame True {
                  }
                  frame False {
                    n135 = while {
                      tunnel: w143 -> [w157]
                      shift-right: [w154] -> w142
                      shift-left: w144 -> [w156]
                      shift-right: [w155] -> w141
                      shift-left: w145 -> [w158]
                      tunnel: [w151] -> _
                      tunnel: w140 -> [w147]
                      i -> [w148]
                      stop <- w153 stop-if-true
                      n136 = Subtract(x=w147, y=w148) -> (x-y=w146:i32)
                      n137 = Decrement(x=w146) -> (x-1=w149:i32)
                      n138 = Index Array(array=w157, index=w149) -> (element=w151:bool)
                      n139 = case shown="True" w151 {
                        tunnel: w156 -> [w160 w166]
                        tunnel: w158 -> [w159 w165]
                        tunnel: [w159 w164] -> w155
                        tunnel: [w160 w163] -> w154
                        tunnel: w146 -> [_ w162]
                        frame False {
                        }
                        frame True {
                          n140 = To Unsigned Byte Integer(number=w162) -> (unsigned 8bit integer=w161:u8)
                          n141 = Enqueue Element(queue=w166, element=w161, error in (no error)=w165) -> (queue out=w163:refnum<queue>, error out=w164:errorcluster)  [unwired: 1 in, 1 out]
                        }
                      }
                      n142 = Equal?(x=w146, y=1) -> (x = y?=w152:bool)
                      n143 = Or(x=w151, y=w152) -> (x .or. y?=w153:bool)
                    }
                  }
                }
              }
              frame "Stop" {
                # "Выстраиваем очеред при остановке лифта"
                n144 = Flush Queue(queue=w258, error in (no error)=w259) -> (queue out=w257:refnum<queue>, error out=w256:errorcluster)  [unwired: 1 out]
                n145 = case shown="\"Going Down\"" w260 {
                  tunnel: w257 -> [w292 w495]
                  tunnel: w256 -> [w291 w494]
                  tunnel: [w290 w493] -> w265
                  tunnel: [w289 w492] -> w264
                  tunnel: w263 -> [w287 w490]
                  tunnel: w262 -> [w267 w472]
                  tunnel: w261 -> [w283 w487]
                  frame "Going Up", Default {
                    w270 = T8 12 items=["Floor Length"=48, "Sum of Floors"=12, "Floor Step in ms"=63, "Elevator Door Step in ms"=30, "Global Wait in ms"=20, "Event Wait in ms"=100] ("Elevator Constants")
                    # "Учитываем приоритет: есть ли\nкакой-то этаж, вызванный в кабине, но находящийся ниже\nтекущего положения кабины?"
                    # "Учитываем, на каком этаже\nсейчас находится лифт и убираем его из массивов-масок кабины и лифта"
                    # "Если был нажат вызов с этажа дома, который уже выбран в кабине то в очередь не добавляем.\nВ отдельных массивах-максках кабины и лифта учитываем, какие этажи уже были добавлены в очередь."
                    # "Перебираем вызовы верхних этажей в кабине"
                    n146 = Decrement(x=w267) -> (x-1=w282:i32)
                    n147 = To Long Integer(number=w270) -> (32bit integer=w269:i32)
                    n148 = Increment(x=w267) -> (x+1=w273:i32)
                    n149 = Replace Array Subset(array=w287, new element=FALSE ("new element/subarray"), index=w282) -> (w286:bool[])
                    n150 = Replace Array Subset(array=w283, new element=FALSE ("new element/subarray"), index=w282) -> (w284:bool[])
                    n151 = Less?(x=w267, y=w269) -> (x < y?=w271:bool)
                    n152 = case shown="True" w271 {
                      tunnel: w292 -> [w326 w336]
                      tunnel: w291 -> [w325 w335]
                      tunnel: w286 -> [w322 w334]
                      tunnel: w284 -> [w321 w333]
                      tunnel: [w321 w332] -> w281
                      tunnel: [w322 w331] -> w280
                      tunnel: [w325 w330] -> w278
                      tunnel: [w326 w329] -> w275
                      tunnel: w273 -> [_ w328]
                      tunnel: [w323 w327] -> w272
                      frame False {
                        w324 = T8 12 items=["Floor Length"=48, "Sum of Floors"=12, "Floor Step in ms"=63, "Elevator Door Step in ms"=30, "Global Wait in ms"=20, "Event Wait in ms"=100] ("Elevator Constants")
                        n153 = To Long Integer(number=w324) -> (32bit integer=w323:i32)
                      }
                      frame True {
                        n154 = while {
                          tunnel: w334 -> [w345]
                          shift-right: [w352] -> w329
                          shift-left: w336 -> [w354]
                          shift-right: [w353] -> w330
                          shift-left: w335 -> [w355]
                          tunnel: w328 -> [w347]
                          shift-right: [w344] -> w331
                          shift-left: w334 -> [w343]
                          shift-right: [w341] -> w332
                          shift-left: w333 -> [w339]
                          shift-right: [w338] -> w327
                          shift-left: w328 -> [w337]
                          i -> [w349]
                          stop <- w348 stop-if-true
                          w346 = T8 12 items=["Floor Length"=48, "Sum of Floors"=12, "Floor Step in ms"=63, "Elevator Door Step in ms"=30, "Global Wait in ms"=20, "Event Wait in ms"=100] ("Elevator Constants")
                          n155 = Add(x=w347, y=w349) -> (x+y=w342:i32)
                          n156 = Decrement(x=w342) -> (x-1=w350:i32)
                          n157 = Index Array(array=w345, index=w350) -> (element=w340:bool)
                          n158 = case shown="True" w340 {
                            tunnel: w342 -> [_ w363]
                            tunnel: [w362 w365] -> w344
                            tunnel: w343 -> [w362 w364]
                            frame False {
                            }
                            frame True {
                              n159 = Decrement(x=w363) -> (x-1=w367:i32)
                              n160 = Replace Array Subset(array=w364, new element=FALSE ("new element/subarray"), index=w367) -> (w365:bool[])
                            }
                          }
                          n161 = case shown="True" w340 {
                            tunnel: [w356 w359] -> w341
                            tunnel: w339 -> [w356 w358]
                            tunnel: w342 -> [_ w357]
                            frame False {
                            }
                            frame True {
                              n162 = Decrement(x=w357) -> (x-1=w361:i32)
                              n163 = Replace Array Subset(array=w358, new element=FALSE ("new element/subarray"), index=w361) -> (w359:bool[])
                            }
                          }
                          n164 = case shown="True" w340 {
                            tunnel: w354 -> [w370 w376]
                            tunnel: w355 -> [w369 w375]
                            tunnel: [w369 w374] -> w353
                            tunnel: [w370 w373] -> w352
                            tunnel: w342 -> [_ w371]
                            tunnel: [w368 w371] -> w338
                            tunnel: w337 -> [w368 _]
                            frame False {
                            }
                            frame True {
                              n165 = To Unsigned Byte Integer(number=w371) -> (unsigned 8bit integer=w372:u8)
                              n166 = Enqueue Element(queue=w376, element=w372, error in (no error)=w375) -> (queue out=w373:refnum<queue>, error out=w374:errorcluster)  [unwired: 1 in, 1 out]
                            }
                          }
                          n167 = To Long Integer(number=w346) -> (32bit integer=w351:i32)
                          n168 = Equal?(x=w342, y=w351) -> (x = y?=w348:bool)
                        }
                      }
                    }
                    n169 = Greater?(x=w267, y=1) -> (0:w268:bool)
                    n170 = case shown="True" w268 {
                      tunnel: w280 -> [w294 w305]
                      tunnel: [w294 w304] -> w279
                      tunnel: w278 -> [w295 w303]
                      tunnel: [w295 w302] -> w277
                      tunnel: [w296 w301] -> w276
                      tunnel: w275 -> [w296 w300]
                      tunnel: [FALSE w298] -> w274
                      tunnel: w267 -> [_ w297]
                      frame False {
                      }
                      frame True {
                        n171 = while {
                          tunnel: w305 -> [w315]
                          tunnel: [w315] -> w304
                          tunnel: w303 -> [w320]
                          tunnel: [w320] -> w302
                          tunnel: [w319] -> w301
                          tunnel: w300 -> [w319]
                          tunnel: w297 -> [w317]
                          shift-right: [w311] -> _
                          shift-left: 0 -> [w312]
                          tunnel: [w310] -> w298
                          i -> [w316]
                          stop <- w308 stop-if-true
                          n172 = Decrement(x=w317) -> (x-1=w318:i32)
                          n173 = Subtract(x=w318, y=w316) -> (x-y=w307:i32)
                          n174 = Decrement(x=w307) -> (x-1=w314:i32)
                          n175 = Index Array(array=w315, index=w314) -> (element=w306:bool)
                          n176 = Increment(x=w312) -> (x+1=w313:i32)
                          n177 = Equal?(x=w307, y=1) -> (x = y?=w308:bool)
                          n178 = Select(t=w313, s=w306, f=w312) -> (s? t:f=w311:i32)
                          n179 = Not Equal To 0?(x=w311) -> (x != 0?=w310:bool)
                        }
                      }
                    }
                    n180 = case shown="True" w274 {
                      tunnel: [w385 w442] -> w290
                      tunnel: [w384 w441] -> w289
                      tunnel: w281 -> [w382 w446]
                      tunnel: w279 -> [w381 w445]
                      tunnel: w277 -> [w380 w444]
                      tunnel: w276 -> [w379 w443]
                      tunnel: w272 -> [w377 _]
                      tunnel: w267 -> [w378 _]
                      frame True {
                        # "Перебираем вызовы нижних этажей, начиная с самого высокого этажа, вызванного в кабине"
                        # "Если есть такой этаж, то добавляем в конец очереди вызовы верхних этажей дома"
                        n181 = while {
                          tunnel: w381 -> [w425]
                          shift-right: [w422] -> w387
                          shift-left: w379 -> [w424]
                          shift-right: [w423] -> w386
                          shift-left: w380 -> [w426]
                          tunnel: w377 -> [w415]
                          tunnel: w382 -> [w419]
                          shift-right: [w412] -> w383
                          shift-left: w382 -> [w413]
                          i -> [w417]
                          stop <- w420 stop-if-true
                          n182 = Decrement(x=w415) -> (x-1=w410:i32)
                          n183 = Subtract(x=w410, y=w417) -> (x-y=w409:i32)
                          n184 = Decrement(x=w409) -> (x-1=w416:i32)
                          n185 = Index Array(array=w425, index=w416) -> (element=w411:bool)
                          n186 = Index Array(array=w419, index=w416) -> (element=w418:bool)
                          n187 = Or(x=w411, y=w418) -> (x .or. y?=w414:bool)
                          n188 = case shown="True" w414 {
                            tunnel: w409 -> [_ w431]
                            tunnel: [w427 w429] -> w412
                            tunnel: w413 -> [w427 w428]
                            frame False {
                            }
                            frame True {
                              n189 = Decrement(x=w431) -> (x-1=w432:i32)
                              n190 = Replace Array Subset(array=w428, new element=FALSE ("new element/subarray"), index=w432) -> (w429:bool[])
                            }
                          }
                          n191 = case shown="True" w414 {
                            tunnel: w424 -> [w434 w440]
                            tunnel: w426 -> [w433 w439]
                            tunnel: [w433 w438] -> w423
                            tunnel: [w434 w437] -> w422
                            tunnel: w409 -> [_ w435]
                            frame False {
                            }
                            frame True {
                              n192 = To Unsigned Byte Integer(number=w435) -> (unsigned 8bit integer=w436:u8)
                              n193 = Enqueue Element(queue=w440, element=w436, error in (no error)=w439) -> (queue out=w437:refnum<queue>, error out=w438:errorcluster)  [unwired: 1 in, 1 out]
                            }
                          }
                          n194 = Less Or Equal?(x=w409, y=1) -> (x <= y?=w420:bool)
                        }
                        n195 = while {
                          tunnel: w383 -> [w399]
                          shift-right: [w396] -> w385
                          shift-left: w387 -> [w398]
                          shift-right: [w397] -> w384
                          shift-left: w386 -> [w400]
                          tunnel: w378 -> [w389]
                          i -> [w394]
                          stop <- w388 stop-if-true
                          w391 = T8 12 items=["Floor Length"=48, "Sum of Floors"=12, "Floor Step in ms"=63, "Elevator Door Step in ms"=30, "Global Wait in ms"=20, "Event Wait in ms"=100] ("Elevator Constants")
                          n196 = To Long Integer(number=w391) -> (32bit integer=w390:i32)
                          n197 = Subtract(x=w390, y=w394) -> (x-y=w393:i32)
                          n198 = Decrement(x=w393) -> (x-1=w392:i32)
                          n199 = Index Array(array=w399, index=w392) -> (element=w395:bool)
                          n200 = Less Or Equal?(x=w393, y=w389) -> (x <= y?=w388:bool)
                          n201 = case shown="True" w395 {
                            tunnel: w398 -> [w402 w408]
                            tunnel: w400 -> [w401 w407]
                            tunnel: [w401 w406] -> w397
                            tunnel: [w402 w405] -> w396
                            tunnel: w393 -> [_ w404]
                            frame False {
                            }
                            frame True {
                              n202 = To Unsigned Byte Integer(number=w404) -> (unsigned 8bit integer=w403:u8)
                              n203 = Enqueue Element(queue=w408, element=w403, error in (no error)=w407) -> (queue out=w405:refnum<queue>, error out=w406:errorcluster)  [unwired: 1 in, 1 out]
                            }
                          }
                        }
                      }
                      frame False {
                        # "Перебираем вызовы на нижних этажа дома, начиная с самого верхнего"
                        n204 = while {
                          tunnel: w445 -> [w461]
                          shift-right: [w458] -> w442
                          shift-left: w443 -> [w460]
                          shift-right: [w459] -> w441
                          shift-left: w444 -> [w462]
                          tunnel: w446 -> [w455]
                          i -> [w453]
                          stop <- w456 stop-if-true
                          w448 = T8 12 items=["Floor Length"=48, "Sum of Floors"=12, "Floor Step in ms"=63, "Elevator Door Step in ms"=30, "Global Wait in ms"=20, "Event Wait in ms"=100] ("Elevator Constants")
                          n205 = To Long Integer(number=w448) -> (32bit integer=w447:i32)
                          n206 = Subtract(x=w447, y=w453) -> (x-y=w449:i32)
                          n207 = Decrement(x=w449) -> (x-1=w452:i32)
                          n208 = Index Array(array=w461, index=w452) -> (element=w450:bool)
                          n209 = Index Array(array=w455, index=w452) -> (element=w454:bool)
                          n210 = Or(x=w450, y=w454) -> (x .or. y?=w451:bool)
                          n211 = case shown="True" w451 {
                            tunnel: w460 -> [w464 w470]
                            tunnel: w462 -> [w463 w469]
                            tunnel: [w463 w468] -> w459
                            tunnel: [w464 w467] -> w458
                            tunnel: w449 -> [_ w465]
                            frame False {
                            }
                            frame True {
                              n212 = To Unsigned Byte Integer(number=w465) -> (unsigned 8bit integer=w466:u8)
                              n213 = Enqueue Element(queue=w470, element=w466, error in (no error)=w469) -> (queue out=w467:refnum<queue>, error out=w468:errorcluster)  [unwired: 1 in, 1 out]
                            }
                          }
                          n214 = Equal?(x=w449, y=1) -> (x = y?=w456:bool)
                        }
                      }
                    }
                  }
                  frame "Going Down" {
                    w476 = T8 12 items=["Floor Length"=48, "Sum of Floors"=12, "Floor Step in ms"=63, "Elevator Door Step in ms"=30, "Global Wait in ms"=20, "Event Wait in ms"=100] ("Elevator Constants")
                    # "Учитываем приоритет: есть ли какой-то этаж, вызванный в кабине, но находящийся выше текущего положения кабины?"
                    # "Учитываем, на каком этаже\nсейчас находится лифт и убираем его из массивов-масок кабины и лифта"
                    # "Если был нажат вызов с этажа дома, который уже выбран в кабине то в очередь не добавляем.\nВ отдельных массивах-максках кабины и лифта учитываем, какие этажи уже были добавлены в очередь."
                    # "Перебираем вызовы нижних этажей в кабине"
                    n215 = Decrement(x=w472) -> (x-1=w486:i32)
                    n216 = Decrement(x=w472) -> (x-1=w474:i32)
                    n217 = Replace Array Subset(array=w490, new element=FALSE ("new element/subarray"), index=w486) -> (w489:bool[])
                    n218 = Replace Array Subset(array=w487, new element=FALSE ("new element/subarray"), index=w486) -> (w480:bool[])
                    n219 = Greater?(x=w472, y=1) -> (0:w473:bool)
                    n220 = case shown="True" w473 {
                      tunnel: w495 -> [w499 w508]
                      tunnel: w494 -> [w498 w507]
                      tunnel: w489 -> [w497 w506]
                      tunnel: [w498 w505] -> w485
                      tunnel: [w499 w504] -> w482
                      tunnel: w480 -> [w496 w503]
                      tunnel: [w497 w502] -> w479
                      tunnel: [w496 w501] -> w478
                      tunnel: w474 -> [_ w500]
                      frame False {
                      }
                      frame True {
                        n221 = while {
                          tunnel: w506 -> [w520]
                          shift-right: [w524] -> w504
                          shift-left: w508 -> [w526]
                          shift-right: [w525] -> w505
                          shift-left: w507 -> [w527]
                          tunnel: w500 -> [w521]
                          shift-right: [w519] -> w502
                          shift-left: w506 -> [w518]
                          shift-right: [w517] -> w501
                          shift-left: w503 -> [w516]
                          tunnel: w503 -> [w513]
                          i -> [w523]
                          stop <- w522 stop-if-true
                          n222 = Subtract(x=w521, y=w523) -> (x-y=w512:i32)
                          n223 = Decrement(x=w512) -> (x-1=w510:i32)
                          n224 = Index Array(array=w513, index=w510) -> (element=w511:bool)
                          n225 = Index Array(array=w520, index=w510) -> (element=w514:bool)
                          n226 = Or(x=w514, y=w511) -> (x .or. y?=w509:bool)
                          n227 = case shown="True" w509 {
                            tunnel: w512 -> [_ w535]
                            tunnel: [w534 w537] -> w519
                            tunnel: w518 -> [w534 w536]
                            frame False {
                            }
                            frame True {
                              n228 = Decrement(x=w535) -> (x-1=w539:i32)
                              n229 = Replace Array Subset(array=w536, new element=FALSE ("new element/subarray"), index=w539) -> (w537:bool[])
                            }
                          }
                          n230 = case shown="True" w509 {
                            tunnel: [w528 w531] -> w517
                            tunnel: w516 -> [w528 w530]
                            tunnel: w512 -> [_ w529]
                            frame False {
                            }
                            frame True {
                              n231 = Decrement(x=w529) -> (x-1=w533:i32)
                              n232 = Replace Array Subset(array=w530, new element=FALSE ("new element/subarray"), index=w533) -> (w531:bool[])
                            }
                          }
                          n233 = case shown="True" w509 {
                            tunnel: w526 -> [w541 w547]
                            tunnel: w527 -> [w540 w546]
                            tunnel: [w540 w545] -> w525
                            tunnel: [w541 w544] -> w524
                            tunnel: w512 -> [_ w542]
                            frame False {
                            }
                            frame True {
                              n234 = To Unsigned Byte Integer(number=w542) -> (unsigned 8bit integer=w543:u8)
                              n235 = Enqueue Element(queue=w547, element=w543, error in (no error)=w546) -> (queue out=w544:refnum<queue>, error out=w545:errorcluster)  [unwired: 1 in, 1 out]
                            }
                          }
                          n236 = Equal?(x=w512, y=1) -> (x = y?=w522:bool)
                        }
                      }
                    }
                    n237 = To Long Integer(number=w476) -> (32bit integer=w475:i32)
                    n238 = Less?(x=w472, y=w475) -> (x < y?=w477:bool)
                    n239 = case shown="True" w477 {
                      tunnel: w485 -> [w548 w558]
                      tunnel: [w548 w557] -> w484
                      tunnel: [w549 w556] -> w483
                      tunnel: w482 -> [w549 w555]
                      tunnel: [FALSE w553] -> w481
                      tunnel: w479 -> [_ w552]
                      tunnel: w472 -> [_ w551]
                      frame False {
                      }
                      frame True {
                        n240 = while {
                          tunnel: w552 -> [w569]
                          tunnel: w558 -> [w574]
                          tunnel: [w574] -> w557
                          tunnel: [w573] -> w556
                          tunnel: w555 -> [w573]
                          tunnel: w551 -> [w571]
                          shift-right: [w565] -> _
                          shift-left: 0 -> [w566]
                          tunnel: [w564] -> w553
                          i -> [w570]
                          stop <- w563 stop-if-true
                          w561 = T8 12 items=["Floor Length"=48, "Sum of Floors"=12, "Floor Step in ms"=63, "Elevator Door Step in ms"=30, "Global Wait in ms"=20, "Event Wait in ms"=100] ("Elevator Constants")
                          n241 = Increment(x=w571) -> (x+1=w572:i32)
                          n242 = Add(x=w572, y=w570) -> (x+y=w562:i32)
                          n243 = Decrement(x=w562) -> (x-1=w568:i32)
                          n244 = Index Array(array=w569, index=w568) -> (element=w559:bool)
                          n245 = To Long Integer(number=w561) -> (32bit integer=w560:i32)
                          n246 = Increment(x=w566) -> (x+1=w567:i32)
                          n247 = Select(t=w567, s=w559, f=w566) -> (s? t:f=w565:i32)
                          n248 = Equal?(x=w562, y=w560) -> (x = y?=w563:bool)
                          n249 = Not Equal To 0?(x=w565) -> (x != 0?=w564:bool)
                        }
                      }
                    }
                    n250 = case shown="True" w481 {
                      tunnel: [w582 w647] -> w493
                      tunnel: [w581 w646] -> w492
                      tunnel: w479 -> [w575 w644]
                      tunnel: w484 -> [w580 w649]
                      tunnel: w483 -> [w579 w648]
                      tunnel: w472 -> [w578 _]
                      tunnel: w478 -> [w577 w645]
                      frame True {
                        # "Если есть такой этаж, то добавляем в конец очереди сначала вызовы верхних этажей кабины, потом вызовы верхних этажей дома"
                        n251 = while {
                          tunnel: w575 -> [w622]
                          shift-right: [w619] -> w584
                          shift-left: w579 -> [w621]
                          shift-right: [w620] -> w583
                          shift-left: w580 -> [w623]
                          tunnel: w578 -> [w615]
                          shift-right: [w613] -> _
                          shift-left: w575 -> [w614]
                          shift-right: [w609] -> w576
                          shift-left: w577 -> [w610]
                          i -> [w617]
                          stop <- w618 stop-if-true
                          w608 = T8 12 items=["Floor Length"=48, "Sum of Floors"=12, "Floor Step in ms"=63, "Elevator Door Step in ms"=30, "Global Wait in ms"=20, "Event Wait in ms"=100] ("Elevator Constants")
                          n252 = Increment(x=w615) -> (x+1=w612:i32)
                          n253 = Add(x=w612, y=w617) -> (x+y=w611:i32)
                          n254 = Decrement(x=w611) -> (x-1=w616:i32)
                          n255 = Index Array(array=w622, index=w616) -> (element=w606:bool)
                          n256 = case shown="True" w606 {
                            tunnel: w611 -> [_ w634]
                            tunnel: [w630 w632] -> w613
                            tunnel: w614 -> [w630 w631]
                            frame False {
                            }
                            frame True {
                              n257 = Decrement(x=w634) -> (x-1=w635:i32)
                              n258 = Replace Array Subset(array=w631, new element=FALSE ("new element/subarray"), index=w635) -> (w632:bool[])
                            }
                          }
                          n259 = case shown="True" w606 {
                            tunnel: [w624 w627] -> w609
                            tunnel: w610 -> [w624 w626]
                            tunnel: w611 -> [_ w625]
                            frame False {
                            }
                            frame True {
                              n260 = Decrement(x=w625) -> (x-1=w629:i32)
                              n261 = Replace Array Subset(array=w626, new element=FALSE ("new element/subarray"), index=w629) -> (w627:bool[])
                            }
                          }
                          n262 = To Long Integer(number=w608) -> (32bit integer=w607:i32)
                          n263 = case shown="True" w606 {
                            tunnel: w621 -> [w637 w643]
                            tunnel: w623 -> [w636 w642]
                            tunnel: [w636 w641] -> w620
                            tunnel: [w637 w640] -> w619
                            tunnel: w611 -> [_ w638]
                            frame False {
                            }
                            frame True {
                              n264 = To Unsigned Byte Integer(number=w638) -> (unsigned 8bit integer=w639:u8)
                              n265 = Enqueue Element(queue=w643, element=w639, error in (no error)=w642) -> (queue out=w640:refnum<queue>, error out=w641:errorcluster)  [unwired: 1 in, 1 out]
                            }
                          }
                          n266 = Equal?(x=w611, y=w607) -> (x = y?=w618:bool)
                        }
                        n267 = while {
                          tunnel: w576 -> [w596]
                          shift-right: [w593] -> w582
                          shift-left: w584 -> [w595]
                          shift-right: [w594] -> w581
                          shift-left: w583 -> [w597]
                          tunnel: w578 -> [w586]
                          i -> [w591]
                          stop <- w585 stop-if-true
                          w588 = T8 12 items=["Floor Length"=48, "Sum of Floors"=12, "Floor Step in ms"=63, "Elevator Door Step in ms"=30, "Global Wait in ms"=20, "Event Wait in ms"=100] ("Elevator Constants")
                          n268 = To Long Integer(number=w588) -> (32bit integer=w587:i32)
                          n269 = Subtract(x=w587, y=w591) -> (x-y=w590:i32)
                          n270 = Decrement(x=w590) -> (x-1=w589:i32)
                          n271 = Index Array(array=w596, index=w589) -> (element=w592:bool)
                          n272 = Equal?(x=w590, y=w586) -> (x = y?=w585:bool)
                          n273 = case shown="True" w592 {
                            tunnel: w595 -> [w599 w605]
                            tunnel: w597 -> [w598 w604]
                            tunnel: [w598 w603] -> w594
                            tunnel: [w599 w602] -> w593
                            tunnel: w590 -> [_ w601]
                            frame False {
                            }
                            frame True {
                              n274 = To Unsigned Byte Integer(number=w601) -> (unsigned 8bit integer=w600:u8)
                              n275 = Enqueue Element(queue=w605, element=w600, error in (no error)=w604) -> (queue out=w602:refnum<queue>, error out=w603:errorcluster)  [unwired: 1 in, 1 out]
                            }
                          }
                        }
                      }
                      frame False {
                        n276 = while {
                          tunnel: w644 -> [w664]
                          shift-right: [w661] -> w647
                          shift-left: w648 -> [w663]
                          shift-right: [w662] -> w646
                          shift-left: w649 -> [w665]
                          tunnel: w645 -> [w658]
                          i -> [w656]
                          stop <- w659 stop-if-true
                          w651 = T8 12 items=["Floor Length"=48, "Sum of Floors"=12, "Floor Step in ms"=63, "Elevator Door Step in ms"=30, "Global Wait in ms"=20, "Event Wait in ms"=100] ("Elevator Constants")
                          n277 = To Long Integer(number=w651) -> (32bit integer=w650:i32)
                          n278 = Subtract(x=w650, y=w656) -> (x-y=w652:i32)
                          n279 = Decrement(x=w652) -> (x-1=w655:i32)
                          n280 = Index Array(array=w664, index=w655) -> (element=w653:bool)
                          n281 = Index Array(array=w658, index=w655) -> (element=w657:bool)
                          n282 = Or(x=w653, y=w657) -> (x .or. y?=w654:bool)
                          n283 = case shown="True" w654 {
                            tunnel: w663 -> [w667 w673]
                            tunnel: w665 -> [w666 w672]
                            tunnel: [w666 w671] -> w662
                            tunnel: [w667 w670] -> w661
                            tunnel: w652 -> [_ w668]
                            frame False {
                            }
                            frame True {
                              n284 = To Unsigned Byte Integer(number=w668) -> (unsigned 8bit integer=w669:u8)
                              n285 = Enqueue Element(queue=w673, element=w669, error in (no error)=w672) -> (queue out=w670:refnum<queue>, error out=w671:errorcluster)  [unwired: 1 in, 1 out]
                            }
                          }
                          n286 = Equal?(x=w652, y=1) -> (x = y?=w659:bool)
                        }
                      }
                    }
                  }
                }
              }
              frame "Going Down" {
                w675 = T8 12 items=["Floor Length"=48, "Sum of Floors"=12, "Floor Step in ms"=63, "Elevator Door Step in ms"=30, "Global Wait in ms"=20, "Event Wait in ms"=100] ("Elevator Constants")
                # "Выстраиваем очеред при движении лифта вниз"
                # "Учитываем приоритет: есть ли какой-то этаж, вызванный в кабине, но находящийся выше текущего положения кабины?"
                # "Если был нажат вызов с этажа дома, который уже выбран в кабине то в очередь не добавляем.\nВ отдельных массивах-максках кабины и лифта учитываем, какие этажи уже были добавлены в очередь."
                # "Перебираем вызовы нижних этажей в кабине и вызовы на этажах дома"
                n287 = Flush Queue(queue=w691, error in (no error)=w692) -> (queue out=w690:refnum<queue>, error out=w689:errorcluster)  [unwired: 1 out]
                n288 = while {
                  tunnel: w679 -> [w840]
                  shift-right: [w844] -> w684
                  shift-left: w690 -> [w846]
                  shift-right: [w845] -> w687
                  shift-left: w689 -> [w847]
                  tunnel: w676 -> [w841]
                  shift-right: [w839] -> w682
                  shift-left: w679 -> [w838]
                  shift-right: [w837] -> w681
                  shift-left: w680 -> [w836]
                  tunnel: w680 -> [w833]
                  i -> [w843]
                  stop <- w842 stop-if-true
                  n289 = Subtract(x=w841, y=w843) -> (x-y=w832:i32)
                  n290 = Decrement(x=w832) -> (x-1=w830:i32)
                  n291 = Index Array(array=w833, index=w830) -> (element=w831:bool)
                  n292 = Index Array(array=w840, index=w830) -> (element=w834:bool)
                  n293 = Or(x=w834, y=w831) -> (x .or. y?=w829:bool)
                  n294 = case shown="True" w829 {
                    tunnel: w832 -> [_ w855]
                    tunnel: [w854 w857] -> w839
                    tunnel: w838 -> [w854 w856]
                    frame False {
                    }
                    frame True {
                      n295 = Decrement(x=w855) -> (x-1=w859:i32)
                      n296 = Replace Array Subset(array=w856, new element=FALSE ("new element/subarray"), index=w859) -> (w857:bool[])
                    }
                  }
                  n297 = case shown="True" w829 {
                    tunnel: [w848 w851] -> w837
                    tunnel: w836 -> [w848 w850]
                    tunnel: w832 -> [_ w849]
                    frame False {
                    }
                    frame True {
                      n298 = Decrement(x=w849) -> (x-1=w853:i32)
                      n299 = Replace Array Subset(array=w850, new element=FALSE ("new element/subarray"), index=w853) -> (w851:bool[])
                    }
                  }
                  n300 = case shown="False" w829 {
                    tunnel: w846 -> [w861 w867]
                    tunnel: w847 -> [w860 w866]
                    tunnel: [w860 w865] -> w845
                    tunnel: [w861 w864] -> w844
                    tunnel: w832 -> [_ w862]
                    frame False {
                    }
                    frame True {
                      n301 = To Unsigned Byte Integer(number=w862) -> (unsigned 8bit integer=w863:u8)
                      n302 = Enqueue Element(queue=w867, element=w863, error in (no error)=w866) -> (queue out=w864:refnum<queue>, error out=w865:errorcluster)  [unwired: 1 in, 1 out]
                    }
                  }
                  n303 = Equal?(x=w832, y=1) -> (x = y?=w842:bool)
                }
                n304 = To Long Integer(number=w675) -> (32bit integer=w674:i32)
                n305 = Less?(x=w676, y=w674) -> (x < y?=w677:bool)
                n306 = case shown="True" w677 {
                  tunnel: [w696 w707] -> w688
                  tunnel: w687 -> [w697 w706]
                  tunnel: [w697 w705] -> w686
                  tunnel: [w698 w704] -> w685
                  tunnel: w684 -> [w698 w703]
                  tunnel: [FALSE w701] -> w683
                  tunnel: w682 -> [w696 w700]
                  tunnel: w676 -> [_ w699]
                  frame False {
                  }
                  frame True {
                    n307 = while {
                      tunnel: w700 -> [w718]
                      tunnel: [w718] -> w707
                      tunnel: w706 -> [w723]
                      tunnel: [w723] -> w705
                      tunnel: [w722] -> w704
                      tunnel: w703 -> [w722]
                      tunnel: w699 -> [w720]
                      shift-right: [w714] -> _
                      shift-left: 0 -> [w715]
                      tunnel: [w713] -> w701
                      i -> [w719]
                      stop <- w712 stop-if-true
                      w710 = T8 12 items=["Floor Length"=48, "Sum of Floors"=12, "Floor Step in ms"=63, "Elevator Door Step in ms"=30, "Global Wait in ms"=20, "Event Wait in ms"=100] ("Elevator Constants")
                      n308 = Increment(x=w720) -> (x+1=w721:i32)
                      n309 = Add(x=w721, y=w719) -> (x+y=w711:i32)
                      n310 = Decrement(x=w711) -> (x-1=w717:i32)
                      n311 = Index Array(array=w718, index=w717) -> (element=w708:bool)
                      n312 = To Long Integer(number=w710) -> (32bit integer=w709:i32)
                      n313 = Increment(x=w715) -> (x+1=w716:i32)
                      n314 = Select(t=w716, s=w708, f=w715) -> (s? t:f=w714:i32)
                      n315 = Equal?(x=w711, y=w709) -> (x = y?=w712:bool)
                      n316 = Not Equal To 0?(x=w714) -> (x != 0?=w713:bool)
                    }
                  }
                }
                n317 = case shown="True" w683 {
                  tunnel: [w736 w801] -> w694
                  tunnel: [w735 w800] -> w693
                  tunnel: w682 -> [w728 _]
                  tunnel: w688 -> [w734 w804]
                  tunnel: w686 -> [w733 w803]
                  tunnel: w685 -> [w732 w802]
                  tunnel: w676 -> [w731 _]
                  tunnel: w681 -> [w730 w799]
                  tunnel: [TRUE ("Update Target Floor") TRUE ("Update Target Floor")] -> w678
                  frame True {
                    # "Если есть такой этаж, то добавляем в конец очереди сначала вызовы верхних этажей кабины от меньшего к большему, потом вызовы верхних этажей дома"
                    n318 = while {
                      tunnel: w734 -> [w776]
                      shift-right: [w773] -> w738
                      shift-left: w732 -> [w775]
                      shift-right: [w774] -> w737
                      shift-left: w733 -> [w777]
                      tunnel: w731 -> [w769]
                      shift-right: [w767] -> _
                      shift-left: w728 -> [w768]
                      shift-right: [w763] -> w729
                      shift-left: w730 -> [w764]
                      i -> [w771]
                      stop <- w772 stop-if-true
                      w762 = T8 12 items=["Floor Length"=48, "Sum of Floors"=12, "Floor Step in ms"=63, "Elevator Door Step in ms"=30, "Global Wait in ms"=20, "Event Wait in ms"=100] ("Elevator Constants")
                      n319 = Increment(x=w769) -> (x+1=w766:i32)
                      n320 = Add(x=w766, y=w771) -> (x+y=w765:i32)
                      n321 = Decrement(x=w765) -> (x-1=w770:i32)
                      n322 = Index Array(array=w776, index=w770) -> (element=w760:bool)
                      n323 = case shown="True" w760 {
                        tunnel: w765 -> [_ w788]
                        tunnel: [w784 w786] -> w767
                        tunnel: w768 -> [w784 w785]
                        frame False {
                        }
                        frame True {
                          n324 = Decrement(x=w788) -> (x-1=w789:i32)
                          n325 = Replace Array Subset(array=w785, new element=FALSE ("new element/subarray"), index=w789) -> (w786:bool[])
                        }
                      }
                      n326 = case shown="True" w760 {
                        tunnel: [w778 w781] -> w763
                        tunnel: w764 -> [w778 w780]
                        tunnel: w765 -> [_ w779]
                        frame False {
                        }
                        frame True {
                          n327 = Decrement(x=w779) -> (x-1=w783:i32)
                          n328 = Replace Array Subset(array=w780, new element=FALSE ("new element/subarray"), index=w783) -> (w781:bool[])
                        }
                      }
                      n329 = To Long Integer(number=w762) -> (32bit integer=w761:i32)
                      n330 = case shown="True" w760 {
                        tunnel: w775 -> [w791 w797]
                        tunnel: w777 -> [w790 w796]
                        tunnel: [w790 w795] -> w774
                        tunnel: [w791 w794] -> w773
                        tunnel: w765 -> [_ w792]
                        frame False {
                        }
                        frame True {
                          n331 = To Unsigned Byte Integer(number=w792) -> (unsigned 8bit integer=w793:u8)
                          n332 = Enqueue Element(queue=w797, element=w793, error in (no error)=w796) -> (queue out=w794:refnum<queue>, error out=w795:errorcluster)  [unwired: 1 in, 1 out]
                        }
                      }
                      n333 = Equal?(x=w765, y=w761) -> (x = y?=w772:bool)
                    }
                    n334 = while {
                      tunnel: w729 -> [w750]
                      shift-right: [w747] -> w736
                      shift-left: w738 -> [w749]
                      shift-right: [w748] -> w735
                      shift-left: w737 -> [w751]
                      tunnel: w731 -> [w740]
                      i -> [w745]
                      stop <- w739 stop-if-true
                      w742 = T8 12 items=["Floor Length"=48, "Sum of Floors"=12, "Floor Step in ms"=63, "Elevator Door Step in ms"=30, "Global Wait in ms"=20, "Event Wait in ms"=100] ("Elevator Constants")
                      n335 = To Long Integer(number=w742) -> (32bit integer=w741:i32)
                      n336 = Subtract(x=w741, y=w745) -> (x-y=w744:i32)
                      n337 = Decrement(x=w744) -> (x-1=w743:i32)
                      n338 = Index Array(array=w750, index=w743) -> (element=w746:bool)
                      n339 = Equal?(x=w744, y=w740) -> (x = y?=w739:bool)
                      n340 = case shown="True" w746 {
                        tunnel: w749 -> [w753 w759]
                        tunnel: w751 -> [w752 w758]
                        tunnel: [w752 w757] -> w748
                        tunnel: [w753 w756] -> w747
                        tunnel: w744 -> [_ w755]
                        frame False {
                        }
                        frame True {
                          n341 = To Unsigned Byte Integer(number=w755) -> (unsigned 8bit integer=w754:u8)
                          n342 = Enqueue Element(queue=w759, element=w754, error in (no error)=w758) -> (queue out=w756:refnum<queue>, error out=w757:errorcluster)  [unwired: 1 in, 1 out]
                        }
                      }
                    }
                  }
                  frame False {
                    n343 = while {
                      tunnel: w804 -> [w819]
                      shift-right: [w816] -> w801
                      shift-left: w802 -> [w818]
                      shift-right: [w817] -> w800
                      shift-left: w803 -> [w820]
                      tunnel: w799 -> [w813]
                      i -> [w811]
                      stop <- w814 stop-if-true
                      w806 = T8 12 items=["Floor Length"=48, "Sum of Floors"=12, "Floor Step in ms"=63, "Elevator Door Step in ms"=30, "Global Wait in ms"=20, "Event Wait in ms"=100] ("Elevator Constants")
                      n344 = To Long Integer(number=w806) -> (32bit integer=w805:i32)
                      n345 = Subtract(x=w805, y=w811) -> (x-y=w807:i32)
                      n346 = Decrement(x=w807) -> (x-1=w810:i32)
                      n347 = Index Array(array=w819, index=w810) -> (element=w808:bool)
                      n348 = Index Array(array=w813, index=w810) -> (element=w812:bool)
                      n349 = Or(x=w808, y=w812) -> (x .or. y?=w809:bool)
                      n350 = case shown="True" w809 {
                        tunnel: w818 -> [w822 w828]
                        tunnel: w820 -> [w821 w827]
                        tunnel: [w821 w826] -> w817
                        tunnel: [w822 w825] -> w816
                        tunnel: w807 -> [_ w823]
                        frame False {
                        }
                        frame True {
                          n351 = To Unsigned Byte Integer(number=w823) -> (unsigned 8bit integer=w824:u8)
                          n352 = Enqueue Element(queue=w828, element=w824, error in (no error)=w827) -> (queue out=w825:refnum<queue>, error out=w826:errorcluster)  [unwired: 1 in, 1 out]
                        }
                      }
                      n353 = Equal?(x=w807, y=1) -> (x = y?=w814:bool)
                    }
                  }
                }
                n354 = flat-sequence {
                  tunnel: w678 -> [w724]
                  frame #0 {
                    n355 = local read "Elevator Automate"() -> (w726:T2)
                    n356 = Bundle By Name(cluster=w726, "Update\nTarget Floor"=w724) -> (w725:T2)
                    n357 = local write "Elevator Automate"(w725) -> ()
                  }
                }
              }
              frame "Going Up" {
                w870 = T8 12 items=["Floor Length"=48, "Sum of Floors"=12, "Floor Step in ms"=63, "Elevator Door Step in ms"=30, "Global Wait in ms"=20, "Event Wait in ms"=100] ("Elevator Constants")
                # "Выстраиваем очеред при движении лифта вверх"
                # "Учитываем приоритет: есть ли какой-то этаж, вызванный в кабине  и находящийся выше\nтекущего положения кабины?"
                # "Учитываем приоритет: есть ли какой-то этаж, вызванный в кабине и  находящийся ниже текущего положения кабины?"
                # "Если был нажат вызов с этажа, который уже выбран в кабине то в очередь не добавляем. В отдельных массивах-максках кабины и лифта учитываем, какие этажи уже были добавлены в очередь."
                # "Перебираем вызовы верхних этажей в кабине"
                n358 = Flush Queue(queue=w887, error in (no error)=w888) -> (queue out=w886:refnum<queue>, error out=w885:errorcluster)  [unwired: 1 out]
                n359 = Increment(x=w868) -> (x+1=w876:i32)
                n360 = To Long Integer(number=w870) -> (32bit integer=w869:i32)
                n361 = Less?(x=w868, y=w869) -> (x < y?=w871:bool)
                n362 = case shown="True" w871 {
                  tunnel: w890 -> [w894 w910]
                  tunnel: w889 -> [w893 w909]
                  tunnel: w886 -> [w898 w908]
                  tunnel: w885 -> [w897 w907]
                  tunnel: [w894 w906] -> w884
                  tunnel: [w897 w905] -> w882
                  tunnel: [w898 w904] -> w879
                  tunnel: w876 -> [_ w903]
                  tunnel: [0 w902] -> w875
                  tunnel: [w893 w901] -> w874
                  tunnel: [FALSE w899] -> w873
                  frame False {
                  }
                  frame True {
                    n363 = while {
                      tunnel: w910 -> [w923]
                      shift-right: [w930] -> w904
                      shift-left: w908 -> [w932]
                      shift-right: [w931] -> w905
                      shift-left: w907 -> [w933]
                      tunnel: w903 -> [w925]
                      shift-right: [w922] -> w906
                      shift-left: w910 -> [w921]
                      shift-right: [w917] -> w901
                      shift-left: w909 -> [w919]
                      shift-right: [w913] -> w902
                      shift-left: w903 -> [w918]
                      shift-right: [w912] -> _
                      shift-left: 0 -> [w914]
                      tunnel: [w911] -> w899
                      i -> [w927]
                      stop <- w926 stop-if-true
                      w924 = T8 12 items=["Floor Length"=48, "Sum of Floors"=12, "Floor Step in ms"=63, "Elevator Door Step in ms"=30, "Global Wait in ms"=20, "Event Wait in ms"=100] ("Elevator Constants")
                      n364 = Add(x=w925, y=w927) -> (x+y=w920:i32)
                      n365 = Decrement(x=w920) -> (x-1=w928:i32)
                      n366 = Index Array(array=w923, index=w928) -> (element=w916:bool)
                      n367 = case shown="True" w916 {
                        tunnel: w920 -> [_ w941]
                        tunnel: [w940 w943] -> w922
                        tunnel: w921 -> [w940 w942]
                        frame False {
                        }
                        frame True {
                          n368 = Decrement(x=w941) -> (x-1=w945:i32)
                          n369 = Replace Array Subset(array=w942, new element=FALSE ("new element/subarray"), index=w945) -> (w943:bool[])
                        }
                      }
                      n370 = case shown="True" w916 {
                        tunnel: [w934 w937] -> w917
                        tunnel: w919 -> [w934 w936]
                        tunnel: w920 -> [_ w935]
                        frame False {
                        }
                        frame True {
                          n371 = Decrement(x=w935) -> (x-1=w939:i32)
                          n372 = Replace Array Subset(array=w936, new element=FALSE ("new element/subarray"), index=w939) -> (w937:bool[])
                        }
                      }
                      n373 = case shown="True" w916 {
                        tunnel: w932 -> [w948 w954]
                        tunnel: w933 -> [w947 w953]
                        tunnel: [w947 w952] -> w931
                        tunnel: [w948 w951] -> w930
                        tunnel: w920 -> [_ w949]
                        tunnel: [w946 w949] -> w913
                        tunnel: w918 -> [w946 _]
                        frame False {
                        }
                        frame True {
                          n374 = To Unsigned Byte Integer(number=w949) -> (unsigned 8bit integer=w950:u8)
                          n375 = Enqueue Element(queue=w954, element=w950, error in (no error)=w953) -> (queue out=w951:refnum<queue>, error out=w952:errorcluster)  [unwired: 1 in, 1 out]
                        }
                      }
                      n376 = Increment(x=w914) -> (x+1=w915:i32)
                      n377 = To Long Integer(number=w924) -> (32bit integer=w929:i32)
                      n378 = Equal?(x=w920, y=w929) -> (x = y?=w926:bool)
                      n379 = Select(t=w915, s=w916, f=w914) -> (s? t:f=w912:i32)
                      n380 = Not Equal To 0?(x=w912) -> (x != 0?=w911:bool)
                    }
                  }
                }
                n381 = while {
                  tunnel: w884 -> [w1102]
                  tunnel: [w1102] -> w883
                  tunnel: w882 -> [w1105]
                  tunnel: [w1105] -> w881
                  tunnel: [w1104] -> w880
                  tunnel: w879 -> [w1104]
                  tunnel: w868 -> [w1092]
                  shift-right: [w1098] -> _
                  shift-left: 0 -> [w1099]
                  tunnel: [w1097] -> w877
                  i -> [w1103]
                  stop <- w1095 stop-if-true
                  n382 = Subtract(x=w1092, y=w1103) -> (x-y=w1094:i32)
                  n383 = Decrement(x=w1094) -> (x-1=w1101:i32)
                  n384 = Index Array(array=w1102, index=w1101) -> (element=w1093:bool)
                  n385 = Equal?(x=w1094, y=1) -> (x = y?=w1095:bool)
                  n386 = Increment(x=w1099) -> (x+1=w1100:i32)
                  n387 = Select(t=w1100, s=w1093, f=w1099) -> (s? t:f=w1098:i32)
                  n388 = Not Equal To 0?(x=w1098) -> (x != 0?=w1097:bool)
                }
                n389 = case shown="True" w873 {
                  tunnel: [w961 w995] -> w892
                  tunnel: [w960 w994] -> w891
                  tunnel: w883 -> [w959 w993]
                  tunnel: w881 -> [w958 w992]
                  tunnel: w880 -> [w957 w991]
                  tunnel: w877 -> [_ w990]
                  tunnel: w868 -> [_ w989]
                  tunnel: w875 -> [_ w988]
                  tunnel: w874 -> [w956 w987]
                  tunnel: [TRUE ("Update Target Floor") TRUE ("Update Target Floor")] -> w872
                  frame False {
                    # "Перебираем вызовы  на этажах"
                    n390 = while {
                      tunnel: w959 -> [w976]
                      shift-right: [w973] -> w961
                      shift-left: w957 -> [w975]
                      shift-right: [w974] -> w960
                      shift-left: w958 -> [w977]
                      tunnel: w956 -> [w970]
                      i -> [w968]
                      stop <- w971 stop-if-true
                      w963 = T8 12 items=["Floor Length"=48, "Sum of Floors"=12, "Floor Step in ms"=63, "Elevator Door Step in ms"=30, "Global Wait in ms"=20, "Event Wait in ms"=100] ("Elevator Constants")
                      n391 = To Long Integer(number=w963) -> (32bit integer=w962:i32)
                      n392 = Subtract(x=w962, y=w968) -> (x-y=w964:i32)
                      n393 = Decrement(x=w964) -> (x-1=w967:i32)
                      n394 = Index Array(array=w976, index=w967) -> (element=w965:bool)
                      n395 = Index Array(array=w970, index=w967) -> (element=w969:bool)
                      n396 = Or(x=w965, y=w969) -> (x .or. y?=w966:bool)
                      n397 = case shown="True" w966 {
                        tunnel: w975 -> [w979 w985]
                        tunnel: w977 -> [w978 w984]
                        tunnel: [w978 w983] -> w974
                        tunnel: [w979 w982] -> w973
                        tunnel: w964 -> [_ w980]
                        frame False {
                        }
                        frame True {
                          n398 = To Unsigned Byte Integer(number=w980) -> (unsigned 8bit integer=w981:u8)
                          n399 = Enqueue Element(queue=w985, element=w981, error in (no error)=w984) -> (queue out=w982:refnum<queue>, error out=w983:errorcluster)  [unwired: 1 in, 1 out]
                        }
                      }
                      n400 = Equal?(x=w964, y=1) -> (x = y?=w971:bool)
                    }
                  }
                  frame True {
                    n401 = case shown="True" w990 {
                      tunnel: [w1004 w1060] -> w995
                      tunnel: [w1003 w1059] -> w994
                      tunnel: w987 -> [w1001 w1064]
                      tunnel: w993 -> [w1000 w1063]
                      tunnel: w992 -> [w999 w1062]
                      tunnel: w991 -> [w998 w1061]
                      tunnel: w988 -> [w997 _]
                      tunnel: w989 -> [w996 _]
                      frame True {
                        # "Перебираем вызовы нижних этажей в кабине и на этажах"
                        # "Добавляем в конец очереди вызовы с верхних этажей, если в кабине есть вызовы на этажи ниже, чем его текущее положение"
                        n402 = while {
                          tunnel: w1000 -> [w1043]
                          shift-right: [w1040] -> w1006
                          shift-left: w998 -> [w1042]
                          shift-right: [w1041] -> w1005
                          shift-left: w999 -> [w1044]
                          tunnel: w997 -> [w1028]
                          tunnel: w1001 -> [w1037]
                          shift-right: [w1031] -> w1002
                          shift-left: w1001 -> [w1032]
                          i -> [w1035]
                          stop <- w1038 stop-if-true
                          n403 = Subtract(x=w1028, y=w1035) -> (x-y=w1029:i32)
                          n404 = Decrement(x=w1029) -> (x-1=w1034:i32)
                          n405 = Index Array(array=w1043, index=w1034) -> (element=w1030:bool)
                          n406 = Index Array(array=w1037, index=w1034) -> (element=w1036:bool)
                          n407 = Or(x=w1030, y=w1036) -> (x .or. y?=w1033:bool)
                          n408 = case shown="True" w1033 {
                            tunnel: w1029 -> [_ w1046]
                            tunnel: [w1045 w1048] -> w1031
                            tunnel: w1032 -> [w1045 w1047]
                            frame False {
                            }
                            frame True {
                              n409 = Decrement(x=w1046) -> (x-1=w1050:i32)
                              n410 = Replace Array Subset(array=w1047, new element=FALSE ("new element/subarray"), index=w1050) -> (w1048:bool[])
                            }
                          }
                          n411 = case shown="True" w1033 {
                            tunnel: w1042 -> [w1052 w1058]
                            tunnel: w1044 -> [w1051 w1057]
                            tunnel: [w1051 w1056] -> w1041
                            tunnel: [w1052 w1055] -> w1040
                            tunnel: w1029 -> [_ w1053]
                            frame False {
                            }
                            frame True {
                              n412 = To Unsigned Byte Integer(number=w1053) -> (unsigned 8bit integer=w1054:u8)
                              n413 = Enqueue Element(queue=w1058, element=w1054, error in (no error)=w1057) -> (queue out=w1055:refnum<queue>, error out=w1056:errorcluster)  [unwired: 1 in, 1 out]
                            }
                          }
                          n414 = Equal?(x=w1029, y=1) -> (x = y?=w1038:bool)
                        }
                        n415 = while {
                          tunnel: w1002 -> [w1018]
                          shift-right: [w1015] -> w1004
                          shift-left: w1006 -> [w1017]
                          shift-right: [w1016] -> w1003
                          shift-left: w1005 -> [w1019]
                          tunnel: w996 -> [w1008]
                          i -> [w1013]
                          stop <- w1007 stop-if-true
                          w1010 = T8 12 items=["Floor Length"=48, "Sum of Floors"=12, "Floor Step in ms"=63, "Elevator Door Step in ms"=30, "Global Wait in ms"=20, "Event Wait in ms"=100] ("Elevator Constants")
                          n416 = To Long Integer(number=w1010) -> (32bit integer=w1009:i32)
                          n417 = Subtract(x=w1009, y=w1013) -> (x-y=w1012:i32)
                          n418 = Decrement(x=w1012) -> (x-1=w1011:i32)
                          n419 = Index Array(array=w1018, index=w1011) -> (element=w1014:bool)
                          n420 = Equal?(x=w1012, y=w1008) -> (x = y?=w1007:bool)
                          n421 = case shown="True" w1014 {
                            tunnel: w1017 -> [w1021 w1027]
                            tunnel: w1019 -> [w1020 w1026]
                            tunnel: [w1020 w1025] -> w1016
                            tunnel: [w1021 w1024] -> w1015
                            tunnel: w1012 -> [_ w1023]
                            frame False {
                            }
                            frame True {
                              n422 = To Unsigned Byte Integer(number=w1023) -> (unsigned 8bit integer=w1022:u8)
                              n423 = Enqueue Element(queue=w1027, element=w1022, error in (no error)=w1026) -> (queue out=w1024:refnum<queue>, error out=w1025:errorcluster)  [unwired: 1 in, 1 out]
                            }
                          }
                        }
                      }
                      frame False {
                        # "Перебираем вызовы  на этажах"
                        n424 = while {
                          tunnel: w1063 -> [w1079]
                          shift-right: [w1076] -> w1060
                          shift-left: w1061 -> [w1078]
                          shift-right: [w1077] -> w1059
                          shift-left: w1062 -> [w1080]
                          tunnel: w1064 -> [w1073]
                          i -> [w1071]
                          stop <- w1074 stop-if-true
                          w1066 = T8 12 items=["Floor Length"=48, "Sum of Floors"=12, "Floor Step in ms"=63, "Elevator Door Step in ms"=30, "Global Wait in ms"=20, "Event Wait in ms"=100] ("Elevator Constants")
                          n425 = To Long Integer(number=w1066) -> (32bit integer=w1065:i32)
                          n426 = Subtract(x=w1065, y=w1071) -> (x-y=w1067:i32)
                          n427 = Decrement(x=w1067) -> (x-1=w1070:i32)
                          n428 = Index Array(array=w1079, index=w1070) -> (element=w1068:bool)
                          n429 = Index Array(array=w1073, index=w1070) -> (element=w1072:bool)
                          n430 = Or(x=w1068, y=w1072) -> (x .or. y?=w1069:bool)
                          n431 = case shown="True" w1069 {
                            tunnel: w1078 -> [w1082 w1088]
                            tunnel: w1080 -> [w1081 w1087]
                            tunnel: [w1081 w1086] -> w1077
                            tunnel: [w1082 w1085] -> w1076
                            tunnel: w1067 -> [_ w1083]
                            frame False {
                            }
                            frame True {
                              n432 = To Unsigned Byte Integer(number=w1083) -> (unsigned 8bit integer=w1084:u8)
                              n433 = Enqueue Element(queue=w1088, element=w1084, error in (no error)=w1087) -> (queue out=w1085:refnum<queue>, error out=w1086:errorcluster)  [unwired: 1 in, 1 out]
                            }
                          }
                          n434 = Equal?(x=w1067, y=1) -> (x = y?=w1074:bool)
                        }
                      }
                    }
                  }
                }
                n435 = flat-sequence {
                  tunnel: w872 -> [w1089]
                  frame #0 {
                    n436 = local read "Elevator Automate"() -> (w1091:T2)
                    n437 = Bundle By Name(cluster=w1091, "Update\nTarget Floor"=w1089) -> (w1090:T2)
                    n438 = local write "Elevator Automate"(w1090) -> ()
                  }
                }
              }
              frame "Cancel" {
              }
            }
          }
        }
      }
    }
    n439 = local read "Global Wait in ms"() -> (w18:u32)
    n440 = Wait (ms)(milliseconds to wait=w18) -> ()  [unwired: 1 out]
    n441 = local read "STOP"() -> (w31:bool)
  }
  n442 = flat-sequence {
    tunnel: ["Floors Schematic"] -> w2
    tunnel: ["Elevator Panel"] -> w1
    tunnel: [w1184] -> w7
    tunnel: [w1183] -> w6
    tunnel: [w1177] -> w9
    tunnel: [w1188] -> w5
    tunnel: [w1187] -> w4
    frame #0 {
      w1179 = FALSE ("Open Doors")
      w1196 = T8 12 items=["Floor Length"=48, "Sum of Floors"=12, "Floor Step in ms"=63, "Elevator Door Step in ms"=30, "Global Wait in ms"=20, "Event Wait in ms"=100] ("Elevator Constants")
      w1198 = T8 12 items=["Floor Length"=48, "Sum of Floors"=12, "Floor Step in ms"=63, "Elevator Door Step in ms"=30, "Global Wait in ms"=20, "Event Wait in ms"=100] ("Elevator Constants")
      w1194 = FALSE ("GoTo Idle")
      n443 = stacked-sequence {
        tunnel: [w1374 _] -> w1213
        frame #0 {
          n444 = control-ref of="Call 1"() -> (w1369:refnum<vi>)
          n445 = property class="Bool (strict)"(reference=w1369) -> ("Left"=w1371:i32, "Top"=w1373:i32)  [unwired: 1 in, 2 out]
          n446 = control-ref of="Elevator Cabin"() -> (w1375:refnum<vi>)
          n447 = Add(x=w1373, y=1) -> (x+y=w1368:i32)
          n448 = Add(x=w1371, y=100) -> (x+y=w1367:i32)
          n449 = property class="Slide (strict)"(reference=w1375, "Left"=w1367, "Top"=w1368) -> (reference out=w1374:refnum<vi>)  [unwired: 1 in, 1 out]
        }
        frame #1 {
          n450 = local write "Elevator Cabin"(T5 100 ("Elevator Cabin")) -> ()
        }
      }
      n451 = property class="Slide (strict)"(reference=w1213) -> ("Top"=w1212:i32)  [unwired: 1 in, 2 out]
      n452 = Unbundle By Name("Floors Schematic") -> ("Floor Position"=w1230:i16[])
      n453 = Bundle(cluster="Floors Schematic", "Call 1"=FALSE, "Call 2"=FALSE, "Call 3"=FALSE, "Call 4"=FALSE, "Call 5"=FALSE, "Call 6"=FALSE, "Call 7"=FALSE, "Call 8"=FALSE, "Call 9"=FALSE, "Call 10"=FALSE, "Call 11"=FALSE, "Call 12"=FALSE) -> (w1202:T4)  [unwired: 1 in]
      n454 = local write "Floors Schematic"(w1202) -> ()
      n455 = To Long Integer(number=w1196) -> (32bit integer=w1195:i32)
      n456 = for {
        N: w1195 -> [_]
        shift-right: [w1384] -> _
        shift-left: w1212 -> [w1379]
        shift-right: [w1381] -> _
        shift-left: w1230 -> [w1383]
        i -> [w1386]
        w1377 = T8 48 items=["Floor Length"=48, "Sum of Floors"=12, "Milliseconds Per Step"=63] ("Elevator Constants")
        n457 = To Long Integer(number=w1377) -> (32bit integer=w1378:i32)
        n458 = To Word Integer(number=w1379) -> (16bit integer=w1385:i16)
        n459 = Replace Array Subset(array=w1383, new element=w1385, index=w1386) -> (w1381:i16[])
        n460 = Subtract(x=w1379, y=w1378) -> (x-y=w1384:i32)
        n461 = local read "Floors Schematic"() -> (w1382:T4)
        n462 = Bundle By Name(cluster=w1382, "Floor Position"=w1381) -> (w1380:T4)
        n463 = local write "Floors Schematic"(w1380) -> ()
      }
      n464 = Bundle(cluster="Elevator Panel", "Open Doors"=FALSE, "Close Doors"=FALSE, "Floor 2"=FALSE, "Floor 1"=FALSE, "Floor 3"=FALSE, "Floor 4"=FALSE, "Floor 5"=FALSE, "Floor 6"=FALSE, "Floor 7"=FALSE, "Floor 8"=FALSE, "Floor 9"=FALSE, "Floor 10"=FALSE, "Floor 11"=FALSE, "Floor 12"=FALSE, "Emergency"=FALSE, "Cancel"=FALSE) -> (w1180:T3)
      n465 = local write "Elevator Panel"(w1180) -> ()
      n466 = To Unsigned Byte Integer(number=1) -> (unsigned 8bit integer=w1200:u8)
      n467 = Obtain Queue(name (unnamed)="Elevator Floor Queue", element data type=w1200) -> (queue out=w1190:refnum<queue>, error out=w1189:errorcluster)  [unwired: 3 in, 1 out]
      n468 = Get Queue Status(queue=w1190, error in (no error)=w1189) -> (queue out=w1188:refnum<queue>, error out=w1187:errorcluster, # elements in queue=→"# elements in Elevator Floor Queue":i32, elements=→"Elevator Floor Queue":u8[])  [unwired: 1 in, 4 out]
      n469 = Bundle By Name(cluster=w1180, "Open Doors"=w1179, "Close Doors"=w1179, "Emergency"=w1179, "Cancel"=w1179) -> (w1178:T3)
      n470 = local write "Elevator Panel"(w1178) -> ()
      n471 = Bundle(cluster="Elevator Automate", "Elevator Panel Array"=bool[] [FALSE, FALSE, FALSE, FALSE, FALSE, FALSE, FALSE, FALSE, FALSE, FALSE, FALSE, FALSE], "Floor Array"=bool[] [FALSE, FALSE, FALSE, FALSE, FALSE, FALSE, FALSE, FALSE, FALSE, FALSE, FALSE, FALSE], "Elevator Command"=Elevator_Command."Idle", "Target Floor"=u8 1, "Forced Stop"=w1194, "Cancel Delay"=w1194, "Elevator Status"=T6."Stand By", "Take a Call"=w1194, "Add Floor\nto Queue"=w1194) -> (w1177:T2)  [unwired: 1 in]
      n472 = To Long Integer(number=w1198) -> (32bit integer=w1197:i32)
      n473 = for {
        N: w1197 -> [_]
        i -> [w1246]
        n474 = Increment(x=w1246) -> (x+1=w1245:i32)
        n475 = case shown="4" w1245 {
          frame 1, Default {
            n476 = local read "Floors Schematic"() -> (w1309:T4)
            n477 = Bundle By Name(cluster=w1309, "Call 1"=FALSE ("Call 12")) -> (w1307:T4)
            n478 = control-ref of="Call 1"() -> (w1311:refnum<vi>)
            n479 = local write "Floors Schematic"(w1307) -> ()
            n480 = property class="Bool (strict)"(reference=w1311, "DisabledEnum"=T7."Enabled" ("Disabled")) -> ()  [unwired: 1 in, 2 out]
          }
          frame 2 {
            n481 = local read "Floors Schematic"() -> (w1314:T4)
            n482 = Bundle By Name(cluster=w1314, "Call 2"=FALSE ("Call 12")) -> (w1312:T4)
            n483 = control-ref of="Call 2"() -> (w1316:refnum<vi>)
            n484 = local write "Floors Schematic"(w1312) -> ()
            n485 = property class="Bool (strict)"(reference=w1316, "DisabledEnum"=T7."Enabled" ("Disabled")) -> ()  [unwired: 1 in, 2 out]
          }
          frame 3 {
            n486 = local read "Floors Schematic"() -> (w1319:T4)
            n487 = Bundle By Name(cluster=w1319, "Call 3"=FALSE ("Call 12")) -> (w1317:T4)
            n488 = control-ref of="Call 3"() -> (w1321:refnum<vi>)
            n489 = local write "Floors Schematic"(w1317) -> ()
            n490 = property class="Bool (strict)"(reference=w1321, "DisabledEnum"=T7."Enabled" ("Disabled")) -> ()  [unwired: 1 in, 2 out]
          }
          frame 4 {
            n491 = local read "Floors Schematic"() -> (w1324:T4)
            n492 = Bundle By Name(cluster=w1324, "Call 4"=FALSE ("Call 12")) -> (w1322:T4)
            n493 = control-ref of="Call 4"() -> (w1326:refnum<vi>)
            n494 = local write "Floors Schematic"(w1322) -> ()
            n495 = property class="Bool (strict)"(reference=w1326, "DisabledEnum"=T7."Enabled" ("Disabled")) -> ()  [unwired: 1 in, 2 out]
          }
          frame 5 {
            n496 = local read "Floors Schematic"() -> (w1329:T4)
            n497 = Bundle By Name(cluster=w1329, "Call 5"=FALSE ("Call 12")) -> (w1327:T4)
            n498 = control-ref of="Call 5"() -> (w1331:refnum<vi>)
            n499 = local write "Floors Schematic"(w1327) -> ()
            n500 = property class="Bool (strict)"(reference=w1331, "DisabledEnum"=T7."Enabled" ("Disabled")) -> ()  [unwired: 1 in, 2 out]
          }
          frame 6 {
            n501 = local read "Floors Schematic"() -> (w1334:T4)
            n502 = Bundle By Name(cluster=w1334, "Call 6"=FALSE ("Call 12")) -> (w1332:T4)
            n503 = control-ref of="Call 6"() -> (w1336:refnum<vi>)
            n504 = local write "Floors Schematic"(w1332) -> ()
            n505 = property class="Bool (strict)"(reference=w1336, "DisabledEnum"=T7."Enabled" ("Disabled")) -> ()  [unwired: 1 in, 2 out]
          }
          frame 7 {
            n506 = local read "Floors Schematic"() -> (w1339:T4)
            n507 = Bundle By Name(cluster=w1339, "Call 7"=FALSE ("Call 12")) -> (w1337:T4)
            n508 = control-ref of="Call 7"() -> (w1341:refnum<vi>)
            n509 = local write "Floors Schematic"(w1337) -> ()
            n510 = property class="Bool (strict)"(reference=w1341, "DisabledEnum"=T7."Enabled" ("Disabled")) -> ()  [unwired: 1 in, 2 out]
          }
          frame 8 {
            n511 = local read "Floors Schematic"() -> (w1344:T4)
            n512 = Bundle By Name(cluster=w1344, "Call 8"=FALSE ("Call 12")) -> (w1342:T4)
            n513 = control-ref of="Call 8"() -> (w1346:refnum<vi>)
            n514 = local write "Floors Schematic"(w1342) -> ()
            n515 = property class="Bool (strict)"(reference=w1346, "DisabledEnum"=T7."Enabled" ("Disabled")) -> ()  [unwired: 1 in, 2 out]
          }
          frame 9 {
            n516 = local read "Floors Schematic"() -> (w1349:T4)
            n517 = Bundle By Name(cluster=w1349, "Call 9"=FALSE ("Call 12")) -> (w1347:T4)
            n518 = control-ref of="Call 9"() -> (w1351:refnum<vi>)
            n519 = local write "Floors Schematic"(w1347) -> ()
            n520 = property class="Bool (strict)"(reference=w1351, "DisabledEnum"=T7."Enabled" ("Disabled")) -> ()  [unwired: 1 in, 2 out]
          }
          frame 10 {
            n521 = local read "Floors Schematic"() -> (w1354:T4)
            n522 = Bundle By Name(cluster=w1354, "Call 10"=FALSE ("Call 12")) -> (w1352:T4)
            n523 = control-ref of="Call 10"() -> (w1356:refnum<vi>)
            n524 = local write "Floors Schematic"(w1352) -> ()
            n525 = property class="Bool (strict)"(reference=w1356, "DisabledEnum"=T7."Enabled" ("Disabled")) -> ()  [unwired: 1 in, 2 out]
          }
          frame 11 {
            n526 = local read "Floors Schematic"() -> (w1359:T4)
            n527 = Bundle By Name(cluster=w1359, "Call 11"=FALSE ("Call 12")) -> (w1357:T4)
            n528 = control-ref of="Call 11"() -> (w1361:refnum<vi>)
            n529 = local write "Floors Schematic"(w1357) -> ()
            n530 = property class="Bool (strict)"(reference=w1361, "DisabledEnum"=T7."Enabled" ("Disabled")) -> ()  [unwired: 1 in, 2 out]
          }
          frame 12 {
            n531 = local read "Floors Schematic"() -> (w1364:T4)
            n532 = Bundle By Name(cluster=w1364, "Call 12"=FALSE) -> (w1362:T4)
            n533 = control-ref of="Call 12"() -> (w1366:refnum<vi>)
            n534 = local write "Floors Schematic"(w1362) -> ()
            n535 = property class="Bool (strict)"(reference=w1366, "DisabledEnum"=T7."Enabled" ("Disabled")) -> ()  [unwired: 1 in, 2 out]
          }
        }
        n536 = case shown="4" w1245 {
          frame 1, Default {
            n537 = local read "Elevator Panel"() -> (w1249:T3)
            n538 = Bundle By Name(cluster=w1249, "Floor 1"=FALSE ("Call 12")) -> (w1247:T3)
            n539 = control-ref of="Floor 1"() -> (w1251:refnum<vi>)
            n540 = local write "Elevator Panel"(w1247) -> ()
            n541 = property class="Bool (strict)"(reference=w1251, "DisabledEnum"=T7."Enabled" ("Disabled")) -> ()  [unwired: 1 in, 2 out]
          }
          frame 2 {
            n542 = local read "Elevator Panel"() -> (w1254:T3)
            n543 = Bundle By Name(cluster=w1254, "Floor 2"=FALSE ("Call 12")) -> (w1252:T3)
            n544 = control-ref of="Floor 2"() -> (w1256:refnum<vi>)
            n545 = local write "Elevator Panel"(w1252) -> ()
            n546 = property class="Bool (strict)"(reference=w1256, "DisabledEnum"=T7."Enabled" ("Disabled")) -> ()  [unwired: 1 in, 2 out]
          }
          frame 3 {
            n547 = local read "Elevator Panel"() -> (w1259:T3)
            n548 = Bundle By Name(cluster=w1259, "Floor 3"=FALSE ("Call 12")) -> (w1257:T3)
            n549 = control-ref of="Floor 3"() -> (w1261:refnum<vi>)
            n550 = local write "Elevator Panel"(w1257) -> ()
            n551 = property class="Bool (strict)"(reference=w1261, "DisabledEnum"=T7."Enabled" ("Disabled")) -> ()  [unwired: 1 in, 2 out]
          }
          frame 4 {
            n552 = local read "Elevator Panel"() -> (w1264:T3)
            n553 = Bundle By Name(cluster=w1264, "Floor 4"=FALSE ("Call 12")) -> (w1262:T3)
            n554 = control-ref of="Floor 4"() -> (w1266:refnum<vi>)
            n555 = local write "Elevator Panel"(w1262) -> ()
            n556 = property class="Bool (strict)"(reference=w1266, "DisabledEnum"=T7."Enabled" ("Disabled")) -> ()  [unwired: 1 in, 2 out]
          }
          frame 5 {
            n557 = local read "Elevator Panel"() -> (w1269:T3)
            n558 = Bundle By Name(cluster=w1269, "Floor 5"=FALSE ("Call 12")) -> (w1267:T3)
            n559 = control-ref of="Floor 5"() -> (w1271:refnum<vi>)
            n560 = local write "Elevator Panel"(w1267) -> ()
            n561 = property class="Bool (strict)"(reference=w1271, "DisabledEnum"=T7."Enabled" ("Disabled")) -> ()  [unwired: 1 in, 2 out]
          }
          frame 6 {
            n562 = local read "Elevator Panel"() -> (w1274:T3)
            n563 = Bundle By Name(cluster=w1274, "Floor 6"=FALSE ("Call 12")) -> (w1272:T3)
            n564 = control-ref of="Floor 6"() -> (w1276:refnum<vi>)
            n565 = local write "Elevator Panel"(w1272) -> ()
            n566 = property class="Bool (strict)"(reference=w1276, "DisabledEnum"=T7."Enabled" ("Disabled")) -> ()  [unwired: 1 in, 2 out]
          }
          frame 7 {
            n567 = local read "Elevator Panel"() -> (w1279:T3)
            n568 = Bundle By Name(cluster=w1279, "Floor 7"=FALSE ("Call 12")) -> (w1277:T3)
            n569 = control-ref of="Floor 7"() -> (w1281:refnum<vi>)
            n570 = local write "Elevator Panel"(w1277) -> ()
            n571 = property class="Bool (strict)"(reference=w1281, "DisabledEnum"=T7."Enabled" ("Disabled")) -> ()  [unwired: 1 in, 2 out]
          }
          frame 8 {
            n572 = local read "Elevator Panel"() -> (w1284:T3)
            n573 = Bundle By Name(cluster=w1284, "Floor 8"=FALSE ("Call 12")) -> (w1282:T3)
            n574 = control-ref of="Floor 8"() -> (w1286:refnum<vi>)
            n575 = local write "Elevator Panel"(w1282) -> ()
            n576 = property class="Bool (strict)"(reference=w1286, "DisabledEnum"=T7."Enabled" ("Disabled")) -> ()  [unwired: 1 in, 2 out]
          }
          frame 9 {
            n577 = local read "Elevator Panel"() -> (w1289:T3)
            n578 = Bundle By Name(cluster=w1289, "Floor 9"=FALSE ("Call 12")) -> (w1287:T3)
            n579 = control-ref of="Floor 9"() -> (w1291:refnum<vi>)
            n580 = local write "Elevator Panel"(w1287) -> ()
            n581 = property class="Bool (strict)"(reference=w1291, "DisabledEnum"=T7."Enabled" ("Disabled")) -> ()  [unwired: 1 in, 2 out]
          }
          frame 10 {
            n582 = local read "Elevator Panel"() -> (w1294:T3)
            n583 = Bundle By Name(cluster=w1294, "Floor 10"=FALSE ("Call 12")) -> (w1292:T3)
            n584 = control-ref of="Floor 10"() -> (w1296:refnum<vi>)
            n585 = local write "Elevator Panel"(w1292) -> ()
            n586 = property class="Bool (strict)"(reference=w1296, "DisabledEnum"=T7."Enabled" ("Disabled")) -> ()  [unwired: 1 in, 2 out]
          }
          frame 11 {
            n587 = local read "Elevator Panel"() -> (w1299:T3)
            n588 = Bundle By Name(cluster=w1299, "Floor 11"=FALSE ("Call 12")) -> (w1297:T3)
            n589 = control-ref of="Floor 11"() -> (w1301:refnum<vi>)
            n590 = local write "Elevator Panel"(w1297) -> ()
            n591 = property class="Bool (strict)"(reference=w1301, "DisabledEnum"=T7."Enabled" ("Disabled")) -> ()  [unwired: 1 in, 2 out]
          }
          frame 12 {
            n592 = local read "Elevator Panel"() -> (w1304:T3)
            n593 = Bundle By Name(cluster=w1304, "Floor 12"=FALSE ("Call 12")) -> (w1303:T3)
            n594 = control-ref of="Floor 12"() -> (w1306:refnum<vi>)
            n595 = local write "Elevator Panel"(w1303) -> ()
            n596 = property class="Bool (strict)"(reference=w1306, "DisabledEnum"=T7."Enabled" ("Disabled")) -> ()  [unwired: 1 in, 2 out]
          }
        }
      }
      n597 = Unbundle By Name(w1177) -> ("Elevator Command"=w1206:T1)
      n598 = local write "Elevator Automate"(w1177) -> ()
      n599 = Obtain Queue(name (unnamed)="Elevator Command Queue", element data type=w1206) -> (queue out=w1192:refnum<queue>, error out=w1191:errorcluster)  [unwired: 3 in, 1 out]
      n600 = local write "STOP"(FALSE ("STOP")) -> ()
      n601 = Get Queue Status(queue=w1192, error in (no error)=w1191) -> (queue out=w1184:refnum<queue>, error out=w1183:errorcluster, # elements in queue=→"# elements in Elevator Command Queue":i32, elements=→"Elevator Command Queue":T1[])  [unwired: 1 in, 4 out]
      "Elevator Cabin" <- T5 100 ("Elevator Cabin")
      "Passenger Information Board" <- "" ("Passenger Information Board")
      "Delay Timer" <- 0 ("Pause Clock")
    }
  }
  n602 = while {
    shift-right: [w1394] -> w14
    shift-left: w5 -> [w1396]
    shift-right: [w1393] -> w15
    shift-left: w4 -> [w1395]
    shift-right: [w1389] -> w10
    shift-left: w6 -> [w1391]
    shift-right: [w1390] -> w11
    shift-left: w7 -> [w1392]
    tunnel: w2 -> [_]
    tunnel: w1 -> [_]
    stop <- w1397 stop-if-true
    n603 = event shown="[1] \"Elevator Panel.Cancel\": Value Change" {
      selector: _ -> [_ _ _ _ _ _ _ _ _ _ _ _ _ _ _ _]
      dyn-events: _ -> [_ _ _ _ _ _ _ _ _ _ _ _ _ _ _ _]
      timeout: 100 -> [_ _ _ _ _ _ _ _ _ _ _ _ _ _ _ _]
      tunnel: w1396 -> [w1401 w1423 w1615 w1702 w1789 w1876 w1963 w2050 w2137 w2224 w2311 w2398 w2485 w2572 w2652 w2730]
      tunnel: w1395 -> [w1400 w1422 w1614 w1701 w1788 w1875 w1962 w2049 w2136 w2223 w2310 w2397 w2484 w2571 w2651 w2729]
      tunnel: [w1399 w1421 w1613 w1700 w1787 w1874 w1961 w2048 w2135 w2222 w2309 w2396 w2483 w2570 w2652 w2730] -> w1394
      tunnel: [w1398 w1420 w1612 w1699 w1786 w1873 w1960 w2047 w2134 w2221 w2308 w2395 w2482 w2569 w2651 w2729] -> w1393
      tunnel: w1392 -> [w1405 w1430 w1609 w1696 w1783 w1870 w1957 w2044 w2131 w2218 w2305 w2392 w2479 w2566 w2656 w2734]
      tunnel: w1391 -> [w1404 w1429 w1607 w1694 w1781 w1868 w1955 w2042 w2129 w2216 w2303 w2390 w2477 w2564 w2654 w2733]
      tunnel: [w1403 w1428 w1610 w1697 w1784 w1871 w1958 w2045 w2132 w2219 w2306 w2393 w2480 w2567 w2655 w2732] -> w1390
      tunnel: [w1402 w1427 w1608 w1695 w1782 w1869 w1956 w2043 w2130 w2217 w2304 w2391 w2478 w2565 w2653 w2731] -> w1389
      event Timeout {
        n604 = event-data() -> ()  [unwired: 1 in, 3 out]
        n605 = flat-sequence {
          tunnel: w1405 -> [w1417]
          tunnel: w1404 -> [w1416]
          tunnel: [w1415] -> w1403
          tunnel: [w1414] -> w1402
          tunnel: w1401 -> [w1413]
          tunnel: w1400 -> [w1412]
          tunnel: [w1411] -> w1399
          tunnel: [w1410] -> w1398
          frame #0 {
            n606 = Get Queue Status(queue=w1413, return elements? (F)=TRUE, error in (no error)=w1412) -> (queue out=w1411:refnum<queue>, error out=w1410:errorcluster, # elements in queue=w1407:i32, elements=w1406:u8[])  [unwired: 4 out]
            n607 = local write "# elements in Elevator Floor Queue"(w1407) -> ()
            n608 = local write "Elevator Floor Queue"(w1406) -> ()
            n609 = Get Queue Status(queue=w1417, return elements? (F)=TRUE, error in (no error)=w1416) -> (queue out=w1415:refnum<queue>, error out=w1414:errorcluster, # elements in queue=w1409:i32, elements=w1408:T1[])  [unwired: 4 out]
            n610 = local write "# elements in Elevator Command Queue"(w1409) -> ()
            n611 = local write "Elevator Command Queue"(w1408) -> ()
          }
        }
      }
      event Value Change {
        # "Отмена текущего вызова"
        n612 = event-data() -> ("NewVal"=w1426:bool)  [unwired: 1 in, 5 out]
        n613 = local read "Elevator Automate"() -> (w1425:T2)
        n614 = flat-sequence {
          tunnel: w1426 -> [w1439]
          tunnel: w1430 -> [w1438]
          tunnel: [w1437] -> w1428
          tunnel: w1429 -> [w1436]
          tunnel: [w1435] -> w1427
          tunnel: w1423 -> [w1434]
          tunnel: w1422 -> [w1433]
          tunnel: [w1432] -> w1421
          tunnel: [w1431] -> w1420
          frame #0 {
            n615 = case shown="True" w1439 {
              tunnel: [w1443 w1459] -> w1437
              tunnel: [w1442 w1458] -> w1435
              tunnel: w1438 -> [w1443 w1463]
              tunnel: w1436 -> [w1442 w1462]
              tunnel: w1434 -> [w1441 w1456]
              tunnel: w1433 -> [w1440 w1455]
              tunnel: [w1441 w1454] -> w1432
              tunnel: [w1440 w1453] -> w1431
              frame False {
              }
              frame True {
                w1461 = T8 12 items=["Floor Length"=48, "Sum of Floors"=12, "Floor Step in ms"=63, "Elevator Door Step in ms"=30, "Global Wait in ms"=20, "Event Wait in ms"=100] ("Elevator Constants")
                # "Проверка, что лифт на этаже"
                n616 = local read "Elevator Automate"() -> (w1468:T2)
                n617 = control-ref of="Elevator Cabin"() -> (w1467:refnum<vi>)
                n618 = property class="Slide (strict)"(reference=w1467) -> ("Top"=w1464:i32)  [unwired: 1 in, 2 out]
                n619 = local read "Elevator Cabin"() -> (w1448:T5)
                n620 = Unbundle By Name(w1468) -> ("Elevator Command"=w1452:T1)
                n621 = local read "Floors Schematic"() -> (w1466:T4)
                n622 = Unbundle By Name(w1466) -> ("Floor Position"=w1465:i16[])
                n623 = Not Equal?(x=w1452, y=Elevator_Command."Going Up") -> (x != y?=w1450:bool)
                n624 = Not Equal?(x=w1452, y=Elevator_Command."Going Down") -> (x != y?=w1449:bool)
                n625 = Less?(x=w1448, y=T5 100) -> (x < y?=w1445:bool)
                n626 = Or(x=w1450, y=w1449) -> (x .or. y?=w1444:bool)
                n627 = while {
                  tunnel: w1465 -> [w1542]
                  tunnel: w1464 -> [w1540]
                  tunnel: [w1537] -> w1446
                  i -> [w1538]
                  stop <- w1539 stop-if-true
                  n628 = Index Array(array=w1542, index=w1538) -> (element=w1543:i16)
                  n629 = To Long Integer(number=w1543) -> (32bit integer=w1541:i32)
                  n630 = Less Or Equal?(x=w1541, y=w1540) -> (x <= y?=w1539:bool)
                  n631 = Equal?(x=w1540, y=w1541) -> (x = y?=w1544:bool)
                  n632 = case shown="False" w1544 {
                    selector: w1544 -> [w1545 w1546]
                    tunnel: [w1545 w1546] -> w1537
                    frame False {
                    }
                    frame True {
                    }
                  }
                }
                n633 = Compound Arithmetic op=AND(w1446, w1445, w1444) -> (w1451:bool)
                n634 = case shown="False" w1451 {
                  tunnel: [w1556 w1591] -> w1459
                  tunnel: [w1555 w1590] -> w1458
                  tunnel: w1468 -> [w1559 w1592]
                  tunnel: w1463 -> [w1554 w1587]
                  tunnel: w1462 -> [w1553 w1584]
                  tunnel: [w1556 w1591] -> w1457
                  tunnel: w1456 -> [w1550 w1583]
                  tunnel: w1455 -> [w1549 w1582]
                  tunnel: [w1548 w1581] -> w1454
                  tunnel: [w1547 w1580] -> w1453
                  frame True {
                    n635 = Flush Queue(queue=w1554, error in (no error)=w1553) -> (queue out=w1551:refnum<queue>, error out=w1552:errorcluster)  [unwired: 1 out]
                    n636 = Flush Queue(queue=w1550, error in (no error)=w1549) -> (queue out=w1548:refnum<queue>, error out=w1547:errorcluster)  [unwired: 1 out]
                    n637 = flat-sequence {
                      tunnel: w1559 -> [w1565]
                      tunnel: [w1561] -> w1558
                      tunnel: [w1560] -> w1557
                      tunnel: w1551 -> [w1561]
                      tunnel: w1552 -> [w1560]
                      tunnel: [w1570] -> w1556
                      tunnel: [w1569] -> w1555
                      tunnel: w1558 -> [w1567]
                      tunnel: w1557 -> [w1566]
                      frame #0 {
                        n638 = local read "# elements in Elevator Command Queue"() -> (w1563:i32)
                        n639 = Not Equal To 0?(x=w1563) -> (x != 0?=w1562:bool)
                        n640 = Bundle By Name(cluster=w1565, "Forced Stop"=w1562) -> (w1564:T2)
                        n641 = local write "Elevator Automate"(w1564) -> ()
                      }
                      frame #1 {
                        n642 = Enqueue Element(queue=w1567, element=Elevator_Command."Open Doors", error in (no error)=w1566) -> (queue out=w1575:refnum<queue>, error out=w1574:errorcluster)  [unwired: 1 in, 1 out]
                        n643 = Enqueue Element(queue=w1575, element=Elevator_Command."Cancel Delay", error in (no error)=w1574) -> (queue out=w1578:refnum<queue>, error out=w1577:errorcluster)  [unwired: 1 in, 1 out]
                        n644 = Enqueue Element(queue=w1578, element=Elevator_Command."Close Doors", error in (no error)=w1577) -> (queue out=w1572:refnum<queue>, error out=w1571:errorcluster)  [unwired: 1 in, 1 out]
                        n645 = Enqueue Element(queue=w1572, element=Elevator_Command."Idle", error in (no error)=w1571) -> (queue out=w1570:refnum<queue>, error out=w1569:errorcluster)  [unwired: 1 in, 1 out]
                      }
                    }
                  }
                  frame False {
                    n646 = Flush Queue(queue=w1583, error in (no error)=w1582) -> (queue out=w1581:refnum<queue>, error out=w1580:errorcluster)  [unwired: 1 out]
                    n647 = Flush Queue(queue=w1587, error in (no error)=w1584) -> (queue out=w1586:refnum<queue>, error out=w1585:errorcluster)  [unwired: 1 out]
                    n648 = flat-sequence {
                      tunnel: w1592 -> [w1598]
                      tunnel: [w1594] -> w1589
                      tunnel: [w1593] -> w1588
                      tunnel: w1586 -> [w1594]
                      tunnel: w1585 -> [w1593]
                      tunnel: [w1602] -> w1591
                      tunnel: [w1601] -> w1590
                      tunnel: w1589 -> [w1600]
                      tunnel: w1588 -> [w1599]
                      frame #0 {
                        n649 = local read "# elements in Elevator Command Queue"() -> (w1596:i32)
                        n650 = Not Equal To 0?(x=w1596) -> (x != 0?=w1595:bool)
                        n651 = Bundle By Name(cluster=w1598, "Forced Stop"=w1595) -> (w1597:T2)
                        n652 = local write "Elevator Automate"(w1597) -> ()
                      }
                      frame #1 {
                        n653 = Enqueue Element(queue=w1600, element=Elevator_Command."Cancel Delay", error in (no error)=w1599) -> (queue out=w1605:refnum<queue>, error out=w1604:errorcluster)  [unwired: 1 in, 1 out]
                        n654 = Enqueue Element(queue=w1605, element=Elevator_Command."Idle", error in (no error)=w1604) -> (queue out=w1602:refnum<queue>, error out=w1601:errorcluster)  [unwired: 1 in, 1 out]
                      }
                    }
                  }
                }
                n655 = To Long Integer(number=w1461) -> (32bit integer=w1460:i32)
                n656 = for {
                  N: w1460 -> [_]
                  tunnel: w1457 -> [_]
                  i -> [w1475]
                  n657 = Increment(x=w1475) -> (x+1=w1476:i32)
                  n658 = case shown="12" w1476 {
                    frame 1, Default {
                      n659 = local read "Elevator Panel"() -> (w1479:T3)
                      n660 = Bundle By Name(cluster=w1479, "Floor 1"=FALSE ("Call 12")) -> (w1477:T3)
                      n661 = control-ref of="Floor 1"() -> (w1481:refnum<vi>)
                      n662 = local write "Elevator Panel"(w1477) -> ()
                      n663 = property class="Bool (strict)"(reference=w1481, "DisabledEnum"=T7."Enabled" ("Disabled")) -> ()  [unwired: 1 in, 2 out]
                    }
                    frame 2 {
                      n664 = local read "Elevator Panel"() -> (w1484:T3)
                      n665 = Bundle By Name(cluster=w1484, "Floor 2"=FALSE ("Call 12")) -> (w1482:T3)
                      n666 = control-ref of="Floor 2"() -> (w1486:refnum<vi>)
                      n667 = local write "Elevator Panel"(w1482) -> ()
                      n668 = property class="Bool (strict)"(reference=w1486, "DisabledEnum"=T7."Enabled" ("Disabled")) -> ()  [unwired: 1 in, 2 out]
                    }
                    frame 3 {
                      n669 = local read "Elevator Panel"() -> (w1489:T3)
                      n670 = Bundle By Name(cluster=w1489, "Floor 3"=FALSE ("Call 12")) -> (w1487:T3)
                      n671 = control-ref of="Floor 3"() -> (w1491:refnum<vi>)
                      n672 = local write "Elevator Panel"(w1487) -> ()
                      n673 = property class="Bool (strict)"(reference=w1491, "DisabledEnum"=T7."Enabled" ("Disabled")) -> ()  [unwired: 1 in, 2 out]
                    }
                    frame 4 {
                      n674 = local read "Elevator Panel"() -> (w1494:T3)
                      n675 = Bundle By Name(cluster=w1494, "Floor 4"=FALSE ("Call 12")) -> (w1492:T3)
                      n676 = control-ref of="Floor 4"() -> (w1496:refnum<vi>)
                      n677 = local write "Elevator Panel"(w1492) -> ()
                      n678 = property class="Bool (strict)"(reference=w1496, "DisabledEnum"=T7."Enabled" ("Disabled")) -> ()  [unwired: 1 in, 2 out]
                    }
                    frame 5 {
                      n679 = local read "Elevator Panel"() -> (w1499:T3)
                      n680 = Bundle By Name(cluster=w1499, "Floor 5"=FALSE ("Call 12")) -> (w1497:T3)
                      n681 = control-ref of="Floor 5"() -> (w1501:refnum<vi>)
                      n682 = local write "Elevator Panel"(w1497) -> ()
                      n683 = property class="Bool (strict)"(reference=w1501, "DisabledEnum"=T7."Enabled" ("Disabled")) -> ()  [unwired: 1 in, 2 out]
                    }
                    frame 6 {
                      n684 = local read "Elevator Panel"() -> (w1504:T3)
                      n685 = Bundle By Name(cluster=w1504, "Floor 6"=FALSE ("Call 12")) -> (w1502:T3)
                      n686 = control-ref of="Floor 6"() -> (w1506:refnum<vi>)
                      n687 = local write "Elevator Panel"(w1502) -> ()
                      n688 = property class="Bool (strict)"(reference=w1506, "DisabledEnum"=T7."Enabled" ("Disabled")) -> ()  [unwired: 1 in, 2 out]
                    }
                    frame 7 {
                      n689 = local read "Elevator Panel"() -> (w1509:T3)
                      n690 = Bundle By Name(cluster=w1509, "Floor 7"=FALSE ("Call 12")) -> (w1507:T3)
                      n691 = control-ref of="Floor 7"() -> (w1511:refnum<vi>)
                      n692 = local write "Elevator Panel"(w1507) -> ()
                      n693 = property class="Bool (strict)"(reference=w1511, "DisabledEnum"=T7."Enabled" ("Disabled")) -> ()  [unwired: 1 in, 2 out]
                    }
                    frame 8 {
                      n694 = local read "Elevator Panel"() -> (w1514:T3)
                      n695 = Bundle By Name(cluster=w1514, "Floor 8"=FALSE ("Call 12")) -> (w1512:T3)
                      n696 = control-ref of="Floor 8"() -> (w1516:refnum<vi>)
                      n697 = local write "Elevator Panel"(w1512) -> ()
                      n698 = property class="Bool (strict)"(reference=w1516, "DisabledEnum"=T7."Enabled" ("Disabled")) -> ()  [unwired: 1 in, 2 out]
                    }
                    frame 9 {
                      n699 = local read "Elevator Panel"() -> (w1519:T3)
                      n700 = Bundle By Name(cluster=w1519, "Floor 9"=FALSE ("Call 12")) -> (w1517:T3)
                      n701 = control-ref of="Floor 9"() -> (w1521:refnum<vi>)
                      n702 = local write "Elevator Panel"(w1517) -> ()
                      n703 = property class="Bool (strict)"(reference=w1521, "DisabledEnum"=T7."Enabled" ("Disabled")) -> ()  [unwired: 1 in, 2 out]
                    }
                    frame 10 {
                      n704 = local read "Elevator Panel"() -> (w1524:T3)
                      n705 = Bundle By Name(cluster=w1524, "Floor 10"=FALSE ("Call 12")) -> (w1522:T3)
                      n706 = control-ref of="Floor 10"() -> (w1526:refnum<vi>)
                      n707 = local write "Elevator Panel"(w1522) -> ()
                      n708 = property class="Bool (strict)"(reference=w1526, "DisabledEnum"=T7."Enabled" ("Disabled")) -> ()  [unwired: 1 in, 2 out]
                    }
                    frame 11 {
                      n709 = local read "Elevator Panel"() -> (w1529:T3)
                      n710 = Bundle By Name(cluster=w1529, "Floor 11"=FALSE ("Call 12")) -> (w1527:T3)
                      n711 = control-ref of="Floor 11"() -> (w1531:refnum<vi>)
                      n712 = local write "Elevator Panel"(w1527) -> ()
                      n713 = property class="Bool (strict)"(reference=w1531, "DisabledEnum"=T7."Enabled" ("Disabled")) -> ()  [unwired: 1 in, 2 out]
                    }
                    frame 12 {
                      n714 = local read "Elevator Panel"() -> (w1534:T3)
                      n715 = Bundle By Name(cluster=w1534, "Floor 12"=FALSE ("Call 12")) -> (w1533:T3)
                      n716 = control-ref of="Floor 12"() -> (w1536:refnum<vi>)
                      n717 = local write "Elevator Panel"(w1533) -> ()
                      n718 = property class="Bool (strict)"(reference=w1536, "DisabledEnum"=T7."Enabled" ("Disabled")) -> ()  [unwired: 1 in, 2 out]
                    }
                  }
                }
                n719 = flat-sequence {
                  tunnel: w1457 -> [_]
                  frame #0 {
                    n720 = Wait (ms)(milliseconds to wait=u32 250) -> ()  [unwired: 1 out]
                  }
                  frame #1 {
                    n721 = local read "Elevator Panel"() -> (w1474:T3)
                    n722 = Bundle By Name(cluster=w1474, "Cancel"=FALSE ("Open Doors")) -> (w1473:T3)
                    n723 = local write "Elevator Panel"(w1473) -> ()
                  }
                }
              }
            }
          }
        }
        n724 = Bundle By Name(cluster=w1425, "Cancel Delay"=w1426) -> (w1424:T2)
        n725 = local write "Elevator Automate"(w1424) -> ()
      }
      event Value Change {
        n726 = event-data() -> ("NewVal"=w1611:bool)  [unwired: 1 in, 5 out]
        n727 = flat-sequence {
          tunnel: w1615 -> [w1624]
          tunnel: w1614 -> [w1623]
          tunnel: [w1622] -> w1613
          tunnel: [w1621] -> w1612
          tunnel: w1611 -> [w1620]
          tunnel: [w1619] -> w1610
          tunnel: w1609 -> [w1618]
          tunnel: [w1617] -> w1608
          tunnel: w1607 -> [w1616]
          frame #0 {
            n728 = case shown="True" w1620 {
              tunnel: w1624 -> [w1628 w1647]
              tunnel: w1623 -> [w1627 w1646]
              tunnel: [w1628 w1647] -> w1622
              tunnel: [w1627 w1646] -> w1621
              tunnel: [w1626 w1645] -> w1619
              tunnel: w1618 -> [w1626 w1636]
              tunnel: [w1625 w1644] -> w1617
              tunnel: w1616 -> [w1625 w1635]
              frame False {
              }
              frame True {
                n729 = control-ref of="Elevator Cabin"() -> (w1643:refnum<vi>)
                n730 = property class="Slide (strict)"(reference=w1643) -> ("Top"=w1642:i32)  [unwired: 1 in, 2 out]
                n731 = local read "Floors Schematic"() -> (w1640:T4)
                n732 = Preview Queue Element(queue=w1636, timeout in ms (-1)=1, error in (no error)=w1635) -> (timed out?=w1634:bool)  [unwired: 3 out]
                n733 = Unbundle By Name(w1640) -> ("Floor Position"=w1641:i16[])
                n734 = Decrement(x=1 ("32bit integer")) -> (x-1=w1630:i32)
                n735 = Index Array(array=w1641, index=w1630) -> (element=w1638:i16)
                n736 = To Long Integer(number=w1638) -> (32bit integer=w1639:i32)
                n737 = Not Equal?(x=w1639, y=w1642) -> (x != y?=w1633:bool)
                n738 = Select(t=TRUE, s=w1634, f=w1633) -> (s? t:f=w1631:bool)
                n739 = case shown="False" w1631 {
                  tunnel: w1636 -> [w1649 w1661]
                  tunnel: w1635 -> [w1648 w1660]
                  tunnel: [w1649 w1659] -> w1645
                  tunnel: [w1648 w1658] -> w1644
                  frame True {
                    n740 = local read "Elevator Automate"() -> (w1651:T2)
                    n741 = Bundle By Name(cluster=w1651, "Add Floor\nto Queue"=TRUE ("Add to Queue")) -> (w1652:T2)
                    n742 = local write "Elevator Automate"(w1652) -> ()
                  }
                  frame False {
                    n743 = local read "Elevator Automate"() -> (w1665:T2)
                    n744 = Unbundle By Name(w1665) -> ("Elevator Command"=w1664:T1)
                    n745 = Equal?(x=w1664, y=Elevator_Command."Close Doors") -> (x = y?=w1662:bool)
                    n746 = case shown="True" w1662 {
                      tunnel: w1661 -> [w1678 w1693]
                      tunnel: w1660 -> [w1677 w1692]
                      tunnel: [w1676 w1693] -> w1659
                      tunnel: [w1675 w1692] -> w1658
                      tunnel: [FALSE ("Call 12") FALSE ("Call 12")] -> w1653
                      frame True {
                        w1688 = T8 20 items=["Floor Length"=48, "Sum of Floors"=12, "Floor Step in ms"=63, "Elevator Door Step in ms"=30, "Global Wait in ms"=20, "Event Wait in ms"=100] ("Elevator Constants")
                        n747 = local read "Elevator Automate"() -> (w1687:T2)
                        n748 = Flush Queue(queue=w1678, error in (no error)=w1677) -> (queue out=w1674:refnum<queue>, error out=w1673:errorcluster)  [unwired: 1 out]
                        n749 = To Long Integer(number=w1688) -> (32bit integer=w1689:i32)
                        n750 = Preview Queue Element(queue=w1674, timeout in ms (-1)=w1689, error in (no error)=w1673) -> (queue out=w1668:refnum<queue>, timed out?=w1667:bool, error out=w1669:errorcluster)  [unwired: 1 out]
                        n751 = Bundle By Name(cluster=w1687, "Forced Stop"=w1667) -> (w1686:T2)
                        n752 = Enqueue Element(queue=w1668, element=Elevator_Command."Open Doors", error in (no error)=w1669) -> (queue out=w1671:refnum<queue>, error out=w1670:errorcluster)  [unwired: 1 in, 1 out]
                        n753 = local write "Elevator Automate"(w1686) -> ()
                        n754 = Enqueue Element(queue=w1671, element=Elevator_Command."Long Delay", error in (no error)=w1670) -> (queue out=w1685:refnum<queue>, error out=w1684:errorcluster)  [unwired: 1 in, 1 out]
                        n755 = Enqueue Element(queue=w1685, element=Elevator_Command."Close Doors", error in (no error)=w1684) -> (queue out=w1683:refnum<queue>, error out=w1682:errorcluster)  [unwired: 1 in, 1 out]
                        n756 = Enqueue Element(queue=w1683, element=Elevator_Command."Idle", error in (no error)=w1682) -> (queue out=w1676:refnum<queue>, error out=w1675:errorcluster)  [unwired: 1 in, 1 out]
                      }
                      frame False {
                        n757 = Wait (ms)(milliseconds to wait=u32 250) -> ()  [unwired: 1 out]
                      }
                    }
                    n758 = local read "Floors Schematic"() -> (w1657:T4)
                    n759 = local read "Elevator Panel"() -> (w1655:T3)
                    n760 = Bundle By Name(cluster=w1657, "Call 1"=w1653) -> (w1656:T4)
                    n761 = Bundle By Name(cluster=w1655, "Floor 1"=w1653) -> (w1654:T3)
                    n762 = local write "Elevator Panel"(w1654) -> ()
                    n763 = local write "Floors Schematic"(w1656) -> ()
                  }
                }
              }
            }
          }
        }
      }
      event Value Change {
        n764 = event-data() -> ("NewVal"=w1698:bool)  [unwired: 1 in, 5 out]
        n765 = flat-sequence {
          tunnel: w1702 -> [w1711]
          tunnel: w1701 -> [w1710]
          tunnel: [w1709] -> w1700
          tunnel: [w1708] -> w1699
          tunnel: w1698 -> [w1707]
          tunnel: [w1706] -> w1697
          tunnel: w1696 -> [w1705]
          tunnel: [w1704] -> w1695
          tunnel: w1694 -> [w1703]
          frame #0 {
            n766 = case shown="True" w1707 {
              tunnel: w1711 -> [w1715 w1734]
              tunnel: w1710 -> [w1714 w1733]
              tunnel: [w1715 w1734] -> w1709
              tunnel: [w1714 w1733] -> w1708
              tunnel: [w1713 w1732] -> w1706
              tunnel: w1705 -> [w1713 w1723]
              tunnel: [w1712 w1731] -> w1704
              tunnel: w1703 -> [w1712 w1722]
              frame False {
              }
              frame True {
                n767 = control-ref of="Elevator Cabin"() -> (w1730:refnum<vi>)
                n768 = property class="Slide (strict)"(reference=w1730) -> ("Top"=w1729:i32)  [unwired: 1 in, 2 out]
                n769 = local read "Floors Schematic"() -> (w1727:T4)
                n770 = Preview Queue Element(queue=w1723, timeout in ms (-1)=1, error in (no error)=w1722) -> (timed out?=w1721:bool)  [unwired: 3 out]
                n771 = Unbundle By Name(w1727) -> ("Floor Position"=w1728:i16[])
                n772 = Decrement(x=2 ("32bit integer")) -> (x-1=w1717:i32)
                n773 = Index Array(array=w1728, index=w1717) -> (element=w1725:i16)
                n774 = To Long Integer(number=w1725) -> (32bit integer=w1726:i32)
                n775 = Not Equal?(x=w1726, y=w1729) -> (x != y?=w1720:bool)
                n776 = Select(t=TRUE, s=w1721, f=w1720) -> (s? t:f=w1718:bool)
                n777 = case shown="True" w1718 {
                  tunnel: w1723 -> [w1736 w1748]
                  tunnel: w1722 -> [w1735 w1747]
                  tunnel: [w1736 w1746] -> w1732
                  tunnel: [w1735 w1745] -> w1731
                  frame True {
                    n778 = local read "Elevator Automate"() -> (w1738:T2)
                    n779 = Bundle By Name(cluster=w1738, "Add Floor\nto Queue"=TRUE ("Add to Queue")) -> (w1739:T2)
                    n780 = local write "Elevator Automate"(w1739) -> ()
                  }
                  frame False {
                    n781 = local read "Elevator Automate"() -> (w1752:T2)
                    n782 = Unbundle By Name(w1752) -> ("Elevator Command"=w1751:T1)
                    n783 = Equal?(x=w1751, y=Elevator_Command."Close Doors") -> (x = y?=w1749:bool)
                    n784 = case shown="True" w1749 {
                      tunnel: w1748 -> [w1765 w1780]
                      tunnel: w1747 -> [w1764 w1779]
                      tunnel: [w1763 w1780] -> w1746
                      tunnel: [w1762 w1779] -> w1745
                      tunnel: [FALSE ("Call 12") FALSE ("Call 12")] -> w1740
                      frame True {
                        w1775 = T8 20 items=["Floor Length"=48, "Sum of Floors"=12, "Floor Step in ms"=63, "Elevator Door Step in ms"=30, "Global Wait in ms"=20, "Event Wait in ms"=100] ("Elevator Constants")
                        n785 = local read "Elevator Automate"() -> (w1774:T2)
                        n786 = Flush Queue(queue=w1765, error in (no error)=w1764) -> (queue out=w1761:refnum<queue>, error out=w1760:errorcluster)  [unwired: 1 out]
                        n787 = To Long Integer(number=w1775) -> (32bit integer=w1776:i32)
                        n788 = Preview Queue Element(queue=w1761, timeout in ms (-1)=w1776, error in (no error)=w1760) -> (queue out=w1755:refnum<queue>, timed out?=w1754:bool, error out=w1756:errorcluster)  [unwired: 1 out]
                        n789 = Bundle By Name(cluster=w1774, "Forced Stop"=w1754) -> (w1773:T2)
                        n790 = Enqueue Element(queue=w1755, element=Elevator_Command."Open Doors", error in (no error)=w1756) -> (queue out=w1758:refnum<queue>, error out=w1757:errorcluster)  [unwired: 1 in, 1 out]
                        n791 = local write "Elevator Automate"(w1773) -> ()
                        n792 = Enqueue Element(queue=w1758, element=Elevator_Command."Long Delay", error in (no error)=w1757) -> (queue out=w1772:refnum<queue>, error out=w1771:errorcluster)  [unwired: 1 in, 1 out]
                        n793 = Enqueue Element(queue=w1772, element=Elevator_Command."Close Doors", error in (no error)=w1771) -> (queue out=w1770:refnum<queue>, error out=w1769:errorcluster)  [unwired: 1 in, 1 out]
                        n794 = Enqueue Element(queue=w1770, element=Elevator_Command."Idle", error in (no error)=w1769) -> (queue out=w1763:refnum<queue>, error out=w1762:errorcluster)  [unwired: 1 in, 1 out]
                      }
                      frame False {
                        n795 = Wait (ms)(milliseconds to wait=u32 250) -> ()  [unwired: 1 out]
                      }
                    }
                    n796 = local read "Floors Schematic"() -> (w1744:T4)
                    n797 = local read "Elevator Panel"() -> (w1742:T3)
                    n798 = Bundle By Name(cluster=w1744, "Call 2"=w1740) -> (w1743:T4)
                    n799 = Bundle By Name(cluster=w1742, "Floor 2"=w1740) -> (w1741:T3)
                    n800 = local write "Elevator Panel"(w1741) -> ()
                    n801 = local write "Floors Schematic"(w1743) -> ()
                  }
                }
              }
            }
          }
        }
      }
      event Value Change {
        n802 = event-data() -> ("NewVal"=w1785:bool)  [unwired: 1 in, 5 out]
        n803 = flat-sequence {
          tunnel: w1789 -> [w1798]
          tunnel: w1788 -> [w1797]
          tunnel: [w1796] -> w1787
          tunnel: [w1795] -> w1786
          tunnel: w1785 -> [w1794]
          tunnel: [w1793] -> w1784
          tunnel: w1783 -> [w1792]
          tunnel: [w1791] -> w1782
          tunnel: w1781 -> [w1790]
          frame #0 {
            n804 = case shown="True" w1794 {
              tunnel: w1798 -> [w1802 w1821]
              tunnel: w1797 -> [w1801 w1820]
              tunnel: [w1802 w1821] -> w1796
              tunnel: [w1801 w1820] -> w1795
              tunnel: [w1800 w1819] -> w1793
              tunnel: w1792 -> [w1800 w1810]
              tunnel: [w1799 w1818] -> w1791
              tunnel: w1790 -> [w1799 w1809]
              frame False {
              }
              frame True {
                n805 = control-ref of="Elevator Cabin"() -> (w1817:refnum<vi>)
                n806 = property class="Slide (strict)"(reference=w1817) -> ("Top"=w1816:i32)  [unwired: 1 in, 2 out]
                n807 = local read "Floors Schematic"() -> (w1814:T4)
                n808 = Preview Queue Element(queue=w1810, timeout in ms (-1)=1, error in (no error)=w1809) -> (timed out?=w1808:bool)  [unwired: 3 out]
                n809 = Unbundle By Name(w1814) -> ("Floor Position"=w1815:i16[])
                n810 = Decrement(x=3 ("32bit integer")) -> (x-1=w1804:i32)
                n811 = Index Array(array=w1815, index=w1804) -> (element=w1812:i16)
                n812 = To Long Integer(number=w1812) -> (32bit integer=w1813:i32)
                n813 = Not Equal?(x=w1813, y=w1816) -> (x != y?=w1807:bool)
                n814 = Select(t=TRUE, s=w1808, f=w1807) -> (s? t:f=w1805:bool)
                n815 = case shown="False" w1805 {
                  tunnel: w1810 -> [w1823 w1835]
                  tunnel: w1809 -> [w1822 w1834]
                  tunnel: [w1823 w1833] -> w1819
                  tunnel: [w1822 w1832] -> w1818
                  frame True {
                    n816 = local read "Elevator Automate"() -> (w1825:T2)
                    n817 = Bundle By Name(cluster=w1825, "Add Floor\nto Queue"=TRUE ("Add to Queue")) -> (w1826:T2)
                    n818 = local write "Elevator Automate"(w1826) -> ()
                  }
                  frame False {
                    n819 = local read "Elevator Automate"() -> (w1839:T2)
                    n820 = Unbundle By Name(w1839) -> ("Elevator Command"=w1838:T1)
                    n821 = Equal?(x=w1838, y=Elevator_Command."Close Doors") -> (x = y?=w1836:bool)
                    n822 = case shown="True" w1836 {
                      tunnel: w1835 -> [w1852 w1867]
                      tunnel: w1834 -> [w1851 w1866]
                      tunnel: [w1850 w1867] -> w1833
                      tunnel: [w1849 w1866] -> w1832
                      tunnel: [FALSE ("Call 12") FALSE ("Call 12")] -> w1827
                      frame True {
                        w1862 = T8 20 items=["Floor Length"=48, "Sum of Floors"=12, "Floor Step in ms"=63, "Elevator Door Step in ms"=30, "Global Wait in ms"=20, "Event Wait in ms"=100] ("Elevator Constants")
                        n823 = local read "Elevator Automate"() -> (w1861:T2)
                        n824 = Flush Queue(queue=w1852, error in (no error)=w1851) -> (queue out=w1848:refnum<queue>, error out=w1847:errorcluster)  [unwired: 1 out]
                        n825 = To Long Integer(number=w1862) -> (32bit integer=w1863:i32)
                        n826 = Preview Queue Element(queue=w1848, timeout in ms (-1)=w1863, error in (no error)=w1847) -> (queue out=w1842:refnum<queue>, timed out?=w1841:bool, error out=w1843:errorcluster)  [unwired: 1 out]
                        n827 = Bundle By Name(cluster=w1861, "Forced Stop"=w1841) -> (w1860:T2)
                        n828 = Enqueue Element(queue=w1842, element=Elevator_Command."Open Doors", error in (no error)=w1843) -> (queue out=w1845:refnum<queue>, error out=w1844:errorcluster)  [unwired: 1 in, 1 out]
                        n829 = local write "Elevator Automate"(w1860) -> ()
                        n830 = Enqueue Element(queue=w1845, element=Elevator_Command."Long Delay", error in (no error)=w1844) -> (queue out=w1859:refnum<queue>, error out=w1858:errorcluster)  [unwired: 1 in, 1 out]
                        n831 = Enqueue Element(queue=w1859, element=Elevator_Command."Close Doors", error in (no error)=w1858) -> (queue out=w1857:refnum<queue>, error out=w1856:errorcluster)  [unwired: 1 in, 1 out]
                        n832 = Enqueue Element(queue=w1857, element=Elevator_Command."Idle", error in (no error)=w1856) -> (queue out=w1850:refnum<queue>, error out=w1849:errorcluster)  [unwired: 1 in, 1 out]
                      }
                      frame False {
                        n833 = Wait (ms)(milliseconds to wait=u32 250) -> ()  [unwired: 1 out]
                      }
                    }
                    n834 = local read "Floors Schematic"() -> (w1831:T4)
                    n835 = local read "Elevator Panel"() -> (w1829:T3)
                    n836 = Bundle By Name(cluster=w1831, "Call 3"=w1827) -> (w1830:T4)
                    n837 = Bundle By Name(cluster=w1829, "Floor 3"=w1827) -> (w1828:T3)
                    n838 = local write "Elevator Panel"(w1828) -> ()
                    n839 = local write "Floors Schematic"(w1830) -> ()
                  }
                }
              }
            }
          }
        }
      }
      event Value Change {
        n840 = event-data() -> ("NewVal"=w1872:bool)  [unwired: 1 in, 5 out]
        n841 = flat-sequence {
          tunnel: w1876 -> [w1885]
          tunnel: w1875 -> [w1884]
          tunnel: [w1883] -> w1874
          tunnel: [w1882] -> w1873
          tunnel: w1872 -> [w1881]
          tunnel: [w1880] -> w1871
          tunnel: w1870 -> [w1879]
          tunnel: [w1878] -> w1869
          tunnel: w1868 -> [w1877]
          frame #0 {
            n842 = case shown="True" w1881 {
              tunnel: w1885 -> [w1889 w1908]
              tunnel: w1884 -> [w1888 w1907]
              tunnel: [w1889 w1908] -> w1883
              tunnel: [w1888 w1907] -> w1882
              tunnel: [w1887 w1906] -> w1880
              tunnel: w1879 -> [w1887 w1897]
              tunnel: [w1886 w1905] -> w1878
              tunnel: w1877 -> [w1886 w1896]
              frame False {
              }
              frame True {
                n843 = control-ref of="Elevator Cabin"() -> (w1904:refnum<vi>)
                n844 = property class="Slide (strict)"(reference=w1904) -> ("Top"=w1903:i32)  [unwired: 1 in, 2 out]
                n845 = local read "Floors Schematic"() -> (w1901:T4)
                n846 = Preview Queue Element(queue=w1897, timeout in ms (-1)=1, error in (no error)=w1896) -> (timed out?=w1895:bool)  [unwired: 3 out]
                n847 = Unbundle By Name(w1901) -> ("Floor Position"=w1902:i16[])
                n848 = Decrement(x=4 ("32bit integer")) -> (x-1=w1891:i32)
                n849 = Index Array(array=w1902, index=w1891) -> (element=w1899:i16)
                n850 = To Long Integer(number=w1899) -> (32bit integer=w1900:i32)
                n851 = Not Equal?(x=w1900, y=w1903) -> (x != y?=w1894:bool)
                n852 = Select(t=TRUE, s=w1895, f=w1894) -> (s? t:f=w1892:bool)
                n853 = case shown="False" w1892 {
                  tunnel: w1897 -> [w1910 w1922]
                  tunnel: w1896 -> [w1909 w1921]
                  tunnel: [w1910 w1920] -> w1906
                  tunnel: [w1909 w1919] -> w1905
                  frame True {
                    n854 = local read "Elevator Automate"() -> (w1912:T2)
                    n855 = Bundle By Name(cluster=w1912, "Add Floor\nto Queue"=TRUE ("Add to Queue")) -> (w1913:T2)
                    n856 = local write "Elevator Automate"(w1913) -> ()
                  }
                  frame False {
                    n857 = local read "Elevator Automate"() -> (w1926:T2)
                    n858 = Unbundle By Name(w1926) -> ("Elevator Command"=w1925:T1)
                    n859 = Equal?(x=w1925, y=Elevator_Command."Close Doors") -> (x = y?=w1923:bool)
                    n860 = case shown="True" w1923 {
                      tunnel: w1922 -> [w1939 w1954]
                      tunnel: w1921 -> [w1938 w1953]
                      tunnel: [w1937 w1954] -> w1920
                      tunnel: [w1936 w1953] -> w1919
                      tunnel: [FALSE ("Call 12") FALSE ("Call 12")] -> w1914
                      frame True {
                        w1949 = T8 20 items=["Floor Length"=48, "Sum of Floors"=12, "Floor Step in ms"=63, "Elevator Door Step in ms"=30, "Global Wait in ms"=20, "Event Wait in ms"=100] ("Elevator Constants")
                        n861 = local read "Elevator Automate"() -> (w1948:T2)
                        n862 = Flush Queue(queue=w1939, error in (no error)=w1938) -> (queue out=w1935:refnum<queue>, error out=w1934:errorcluster)  [unwired: 1 out]
                        n863 = To Long Integer(number=w1949) -> (32bit integer=w1950:i32)
                        n864 = Preview Queue Element(queue=w1935, timeout in ms (-1)=w1950, error in (no error)=w1934) -> (queue out=w1929:refnum<queue>, timed out?=w1928:bool, error out=w1930:errorcluster)  [unwired: 1 out]
                        n865 = Bundle By Name(cluster=w1948, "Forced Stop"=w1928) -> (w1947:T2)
                        n866 = Enqueue Element(queue=w1929, element=Elevator_Command."Open Doors", error in (no error)=w1930) -> (queue out=w1932:refnum<queue>, error out=w1931:errorcluster)  [unwired: 1 in, 1 out]
                        n867 = local write "Elevator Automate"(w1947) -> ()
                        n868 = Enqueue Element(queue=w1932, element=Elevator_Command."Long Delay", error in (no error)=w1931) -> (queue out=w1946:refnum<queue>, error out=w1945:errorcluster)  [unwired: 1 in, 1 out]
                        n869 = Enqueue Element(queue=w1946, element=Elevator_Command."Close Doors", error in (no error)=w1945) -> (queue out=w1944:refnum<queue>, error out=w1943:errorcluster)  [unwired: 1 in, 1 out]
                        n870 = Enqueue Element(queue=w1944, element=Elevator_Command."Idle", error in (no error)=w1943) -> (queue out=w1937:refnum<queue>, error out=w1936:errorcluster)  [unwired: 1 in, 1 out]
                      }
                      frame False {
                        n871 = Wait (ms)(milliseconds to wait=u32 250) -> ()  [unwired: 1 out]
                      }
                    }
                    n872 = local read "Floors Schematic"() -> (w1918:T4)
                    n873 = local read "Elevator Panel"() -> (w1916:T3)
                    n874 = Bundle By Name(cluster=w1918, "Call 4"=w1914) -> (w1917:T4)
                    n875 = Bundle By Name(cluster=w1916, "Floor 4"=w1914) -> (w1915:T3)
                    n876 = local write "Elevator Panel"(w1915) -> ()
                    n877 = local write "Floors Schematic"(w1917) -> ()
                  }
                }
              }
            }
          }
        }
      }
      event Value Change {
        n878 = event-data() -> ("NewVal"=w1959:bool)  [unwired: 1 in, 5 out]
        n879 = flat-sequence {
          tunnel: w1963 -> [w1972]
          tunnel: w1962 -> [w1971]
          tunnel: [w1970] -> w1961
          tunnel: [w1969] -> w1960
          tunnel: w1959 -> [w1968]
          tunnel: [w1967] -> w1958
          tunnel: w1957 -> [w1966]
          tunnel: [w1965] -> w1956
          tunnel: w1955 -> [w1964]
          frame #0 {
            n880 = case shown="True" w1968 {
              tunnel: w1972 -> [w1976 w1995]
              tunnel: w1971 -> [w1975 w1994]
              tunnel: [w1976 w1995] -> w1970
              tunnel: [w1975 w1994] -> w1969
              tunnel: [w1974 w1993] -> w1967
              tunnel: w1966 -> [w1974 w1984]
              tunnel: [w1973 w1992] -> w1965
              tunnel: w1964 -> [w1973 w1983]
              frame False {
              }
              frame True {
                n881 = control-ref of="Elevator Cabin"() -> (w1991:refnum<vi>)
                n882 = property class="Slide (strict)"(reference=w1991) -> ("Top"=w1990:i32)  [unwired: 1 in, 2 out]
                n883 = local read "Floors Schematic"() -> (w1988:T4)
                n884 = Preview Queue Element(queue=w1984, timeout in ms (-1)=1, error in (no error)=w1983) -> (timed out?=w1982:bool)  [unwired: 3 out]
                n885 = Unbundle By Name(w1988) -> ("Floor Position"=w1989:i16[])
                n886 = Decrement(x=5 ("32bit integer")) -> (x-1=w1978:i32)
                n887 = Index Array(array=w1989, index=w1978) -> (element=w1986:i16)
                n888 = To Long Integer(number=w1986) -> (32bit integer=w1987:i32)
                n889 = Not Equal?(x=w1987, y=w1990) -> (x != y?=w1981:bool)
                n890 = Select(t=TRUE, s=w1982, f=w1981) -> (s? t:f=w1979:bool)
                n891 = case shown="False" w1979 {
                  tunnel: w1984 -> [w1997 w2009]
                  tunnel: w1983 -> [w1996 w2008]
                  tunnel: [w1997 w2007] -> w1993
                  tunnel: [w1996 w2006] -> w1992
                  frame True {
                    n892 = local read "Elevator Automate"() -> (w1999:T2)
                    n893 = Bundle By Name(cluster=w1999, "Add Floor\nto Queue"=TRUE ("Add to Queue")) -> (w2000:T2)
                    n894 = local write "Elevator Automate"(w2000) -> ()
                  }
                  frame False {
                    n895 = local read "Elevator Automate"() -> (w2013:T2)
                    n896 = Unbundle By Name(w2013) -> ("Elevator Command"=w2012:T1)
                    n897 = Equal?(x=w2012, y=Elevator_Command."Close Doors") -> (x = y?=w2010:bool)
                    n898 = case shown="True" w2010 {
                      tunnel: w2009 -> [w2026 w2041]
                      tunnel: w2008 -> [w2025 w2040]
                      tunnel: [w2024 w2041] -> w2007
                      tunnel: [w2023 w2040] -> w2006
                      tunnel: [FALSE ("Call 12") FALSE ("Call 12")] -> w2001
                      frame True {
                        w2036 = T8 20 items=["Floor Length"=48, "Sum of Floors"=12, "Floor Step in ms"=63, "Elevator Door Step in ms"=30, "Global Wait in ms"=20, "Event Wait in ms"=100] ("Elevator Constants")
                        n899 = local read "Elevator Automate"() -> (w2035:T2)
                        n900 = Flush Queue(queue=w2026, error in (no error)=w2025) -> (queue out=w2022:refnum<queue>, error out=w2021:errorcluster)  [unwired: 1 out]
                        n901 = To Long Integer(number=w2036) -> (32bit integer=w2037:i32)
                        n902 = Preview Queue Element(queue=w2022, timeout in ms (-1)=w2037, error in (no error)=w2021) -> (queue out=w2016:refnum<queue>, timed out?=w2015:bool, error out=w2017:errorcluster)  [unwired: 1 out]
                        n903 = Bundle By Name(cluster=w2035, "Forced Stop"=w2015) -> (w2034:T2)
                        n904 = Enqueue Element(queue=w2016, element=Elevator_Command."Open Doors", error in (no error)=w2017) -> (queue out=w2019:refnum<queue>, error out=w2018:errorcluster)  [unwired: 1 in, 1 out]
                        n905 = local write "Elevator Automate"(w2034) -> ()
                        n906 = Enqueue Element(queue=w2019, element=Elevator_Command."Long Delay", error in (no error)=w2018) -> (queue out=w2033:refnum<queue>, error out=w2032:errorcluster)  [unwired: 1 in, 1 out]
                        n907 = Enqueue Element(queue=w2033, element=Elevator_Command."Close Doors", error in (no error)=w2032) -> (queue out=w2031:refnum<queue>, error out=w2030:errorcluster)  [unwired: 1 in, 1 out]
                        n908 = Enqueue Element(queue=w2031, element=Elevator_Command."Idle", error in (no error)=w2030) -> (queue out=w2024:refnum<queue>, error out=w2023:errorcluster)  [unwired: 1 in, 1 out]
                      }
                      frame False {
                        n909 = Wait (ms)(milliseconds to wait=u32 250) -> ()  [unwired: 1 out]
                      }
                    }
                    n910 = local read "Floors Schematic"() -> (w2005:T4)
                    n911 = local read "Elevator Panel"() -> (w2003:T3)
                    n912 = Bundle By Name(cluster=w2005, "Call 5"=w2001) -> (w2004:T4)
                    n913 = Bundle By Name(cluster=w2003, "Floor 5"=w2001) -> (w2002:T3)
                    n914 = local write "Elevator Panel"(w2002) -> ()
                    n915 = local write "Floors Schematic"(w2004) -> ()
                  }
                }
              }
            }
          }
        }
      }
      event Value Change {
        n916 = event-data() -> ("NewVal"=w2046:bool)  [unwired: 1 in, 5 out]
        n917 = flat-sequence {
          tunnel: w2050 -> [w2059]
          tunnel: w2049 -> [w2058]
          tunnel: [w2057] -> w2048
          tunnel: [w2056] -> w2047
          tunnel: w2046 -> [w2055]
          tunnel: [w2054] -> w2045
          tunnel: w2044 -> [w2053]
          tunnel: [w2052] -> w2043
          tunnel: w2042 -> [w2051]
          frame #0 {
            n918 = case shown="True" w2055 {
              tunnel: w2059 -> [w2063 w2082]
              tunnel: w2058 -> [w2062 w2081]
              tunnel: [w2063 w2082] -> w2057
              tunnel: [w2062 w2081] -> w2056
              tunnel: [w2061 w2080] -> w2054
              tunnel: w2053 -> [w2061 w2071]
              tunnel: [w2060 w2079] -> w2052
              tunnel: w2051 -> [w2060 w2070]
              frame False {
              }
              frame True {
                n919 = control-ref of="Elevator Cabin"() -> (w2078:refnum<vi>)
                n920 = property class="Slide (strict)"(reference=w2078) -> ("Top"=w2077:i32)  [unwired: 1 in, 2 out]
                n921 = local read "Floors Schematic"() -> (w2075:T4)
                n922 = Preview Queue Element(queue=w2071, timeout in ms (-1)=1, error in (no error)=w2070) -> (timed out?=w2069:bool)  [unwired: 3 out]
                n923 = Unbundle By Name(w2075) -> ("Floor Position"=w2076:i16[])
                n924 = Decrement(x=6 ("32bit integer")) -> (x-1=w2065:i32)
                n925 = Index Array(array=w2076, index=w2065) -> (element=w2073:i16)
                n926 = To Long Integer(number=w2073) -> (32bit integer=w2074:i32)
                n927 = Not Equal?(x=w2074, y=w2077) -> (x != y?=w2068:bool)
                n928 = Select(t=TRUE, s=w2069, f=w2068) -> (s? t:f=w2066:bool)
                n929 = case shown="False" w2066 {
                  tunnel: w2071 -> [w2084 w2096]
                  tunnel: w2070 -> [w2083 w2095]
                  tunnel: [w2084 w2094] -> w2080
                  tunnel: [w2083 w2093] -> w2079
                  frame True {
                    n930 = local read "Elevator Automate"() -> (w2086:T2)
                    n931 = Bundle By Name(cluster=w2086, "Add Floor\nto Queue"=TRUE ("Add to Queue")) -> (w2087:T2)
                    n932 = local write "Elevator Automate"(w2087) -> ()
                  }
                  frame False {
                    n933 = local read "Elevator Automate"() -> (w2100:T2)
                    n934 = Unbundle By Name(w2100) -> ("Elevator Command"=w2099:T1)
                    n935 = Equal?(x=w2099, y=Elevator_Command."Close Doors") -> (x = y?=w2097:bool)
                    n936 = case shown="True" w2097 {
                      tunnel: w2096 -> [w2113 w2128]
                      tunnel: w2095 -> [w2112 w2127]
                      tunnel: [w2111 w2128] -> w2094
                      tunnel: [w2110 w2127] -> w2093
                      tunnel: [FALSE ("Call 12") FALSE ("Call 12")] -> w2088
                      frame True {
                        w2123 = T8 20 items=["Floor Length"=48, "Sum of Floors"=12, "Floor Step in ms"=63, "Elevator Door Step in ms"=30, "Global Wait in ms"=20, "Event Wait in ms"=100] ("Elevator Constants")
                        n937 = local read "Elevator Automate"() -> (w2122:T2)
                        n938 = Flush Queue(queue=w2113, error in (no error)=w2112) -> (queue out=w2109:refnum<queue>, error out=w2108:errorcluster)  [unwired: 1 out]
                        n939 = To Long Integer(number=w2123) -> (32bit integer=w2124:i32)
                        n940 = Preview Queue Element(queue=w2109, timeout in ms (-1)=w2124, error in (no error)=w2108) -> (queue out=w2103:refnum<queue>, timed out?=w2102:bool, error out=w2104:errorcluster)  [unwired: 1 out]
                        n941 = Bundle By Name(cluster=w2122, "Forced Stop"=w2102) -> (w2121:T2)
                        n942 = Enqueue Element(queue=w2103, element=Elevator_Command."Open Doors", error in (no error)=w2104) -> (queue out=w2106:refnum<queue>, error out=w2105:errorcluster)  [unwired: 1 in, 1 out]
                        n943 = local write "Elevator Automate"(w2121) -> ()
                        n944 = Enqueue Element(queue=w2106, element=Elevator_Command."Long Delay", error in (no error)=w2105) -> (queue out=w2120:refnum<queue>, error out=w2119:errorcluster)  [unwired: 1 in, 1 out]
                        n945 = Enqueue Element(queue=w2120, element=Elevator_Command."Close Doors", error in (no error)=w2119) -> (queue out=w2118:refnum<queue>, error out=w2117:errorcluster)  [unwired: 1 in, 1 out]
                        n946 = Enqueue Element(queue=w2118, element=Elevator_Command."Idle", error in (no error)=w2117) -> (queue out=w2111:refnum<queue>, error out=w2110:errorcluster)  [unwired: 1 in, 1 out]
                      }
                      frame False {
                        n947 = Wait (ms)(milliseconds to wait=u32 250) -> ()  [unwired: 1 out]
                      }
                    }
                    n948 = local read "Floors Schematic"() -> (w2092:T4)
                    n949 = local read "Elevator Panel"() -> (w2090:T3)
                    n950 = Bundle By Name(cluster=w2092, "Call 6"=w2088) -> (w2091:T4)
                    n951 = Bundle By Name(cluster=w2090, "Floor 6"=w2088) -> (w2089:T3)
                    n952 = local write "Elevator Panel"(w2089) -> ()
                    n953 = local write "Floors Schematic"(w2091) -> ()
                  }
                }
              }
            }
          }
        }
      }
      event Value Change {
        n954 = event-data() -> ("NewVal"=w2133:bool)  [unwired: 1 in, 5 out]
        n955 = flat-sequence {
          tunnel: w2137 -> [w2146]
          tunnel: w2136 -> [w2145]
          tunnel: [w2144] -> w2135
          tunnel: [w2143] -> w2134
          tunnel: w2133 -> [w2142]
          tunnel: [w2141] -> w2132
          tunnel: w2131 -> [w2140]
          tunnel: [w2139] -> w2130
          tunnel: w2129 -> [w2138]
          frame #0 {
            n956 = case shown="True" w2142 {
              tunnel: w2146 -> [w2150 w2169]
              tunnel: w2145 -> [w2149 w2168]
              tunnel: [w2150 w2169] -> w2144
              tunnel: [w2149 w2168] -> w2143
              tunnel: [w2148 w2167] -> w2141
              tunnel: w2140 -> [w2148 w2158]
              tunnel: [w2147 w2166] -> w2139
              tunnel: w2138 -> [w2147 w2157]
              frame False {
              }
              frame True {
                n957 = control-ref of="Elevator Cabin"() -> (w2165:refnum<vi>)
                n958 = property class="Slide (strict)"(reference=w2165) -> ("Top"=w2164:i32)  [unwired: 1 in, 2 out]
                n959 = local read "Floors Schematic"() -> (w2162:T4)
                n960 = Preview Queue Element(queue=w2158, timeout in ms (-1)=1, error in (no error)=w2157) -> (timed out?=w2156:bool)  [unwired: 3 out]
                n961 = Unbundle By Name(w2162) -> ("Floor Position"=w2163:i16[])
                n962 = Decrement(x=7 ("32bit integer")) -> (x-1=w2152:i32)
                n963 = Index Array(array=w2163, index=w2152) -> (element=w2160:i16)
                n964 = To Long Integer(number=w2160) -> (32bit integer=w2161:i32)
                n965 = Not Equal?(x=w2161, y=w2164) -> (x != y?=w2155:bool)
                n966 = Select(t=TRUE, s=w2156, f=w2155) -> (s? t:f=w2153:bool)
                n967 = case shown="False" w2153 {
                  tunnel: w2158 -> [w2171 w2183]
                  tunnel: w2157 -> [w2170 w2182]
                  tunnel: [w2171 w2181] -> w2167
                  tunnel: [w2170 w2180] -> w2166
                  frame True {
                    n968 = local read "Elevator Automate"() -> (w2173:T2)
                    n969 = Bundle By Name(cluster=w2173, "Add Floor\nto Queue"=TRUE ("Add to Queue")) -> (w2174:T2)
                    n970 = local write "Elevator Automate"(w2174) -> ()
                  }
                  frame False {
                    n971 = local read "Elevator Automate"() -> (w2187:T2)
                    n972 = Unbundle By Name(w2187) -> ("Elevator Command"=w2186:T1)
                    n973 = Equal?(x=w2186, y=Elevator_Command."Close Doors") -> (x = y?=w2184:bool)
                    n974 = case shown="True" w2184 {
                      tunnel: w2183 -> [w2200 w2215]
                      tunnel: w2182 -> [w2199 w2214]
                      tunnel: [w2198 w2215] -> w2181
                      tunnel: [w2197 w2214] -> w2180
                      tunnel: [FALSE ("Call 12") FALSE ("Call 12")] -> w2175
                      frame True {
                        w2210 = T8 20 items=["Floor Length"=48, "Sum of Floors"=12, "Floor Step in ms"=63, "Elevator Door Step in ms"=30, "Global Wait in ms"=20, "Event Wait in ms"=100] ("Elevator Constants")
                        n975 = local read "Elevator Automate"() -> (w2209:T2)
                        n976 = Flush Queue(queue=w2200, error in (no error)=w2199) -> (queue out=w2196:refnum<queue>, error out=w2195:errorcluster)  [unwired: 1 out]
                        n977 = To Long Integer(number=w2210) -> (32bit integer=w2211:i32)
                        n978 = Preview Queue Element(queue=w2196, timeout in ms (-1)=w2211, error in (no error)=w2195) -> (queue out=w2190:refnum<queue>, timed out?=w2189:bool, error out=w2191:errorcluster)  [unwired: 1 out]
                        n979 = Bundle By Name(cluster=w2209, "Forced Stop"=w2189) -> (w2208:T2)
                        n980 = Enqueue Element(queue=w2190, element=Elevator_Command."Open Doors", error in (no error)=w2191) -> (queue out=w2193:refnum<queue>, error out=w2192:errorcluster)  [unwired: 1 in, 1 out]
                        n981 = local write "Elevator Automate"(w2208) -> ()
                        n982 = Enqueue Element(queue=w2193, element=Elevator_Command."Long Delay", error in (no error)=w2192) -> (queue out=w2207:refnum<queue>, error out=w2206:errorcluster)  [unwired: 1 in, 1 out]
                        n983 = Enqueue Element(queue=w2207, element=Elevator_Command."Close Doors", error in (no error)=w2206) -> (queue out=w2205:refnum<queue>, error out=w2204:errorcluster)  [unwired: 1 in, 1 out]
                        n984 = Enqueue Element(queue=w2205, element=Elevator_Command."Idle", error in (no error)=w2204) -> (queue out=w2198:refnum<queue>, error out=w2197:errorcluster)  [unwired: 1 in, 1 out]
                      }
                      frame False {
                        n985 = Wait (ms)(milliseconds to wait=u32 250) -> ()  [unwired: 1 out]
                      }
                    }
                    n986 = local read "Floors Schematic"() -> (w2179:T4)
                    n987 = local read "Elevator Panel"() -> (w2177:T3)
                    n988 = Bundle By Name(cluster=w2179, "Call 7"=w2175) -> (w2178:T4)
                    n989 = Bundle By Name(cluster=w2177, "Floor 7"=w2175) -> (w2176:T3)
                    n990 = local write "Elevator Panel"(w2176) -> ()
                    n991 = local write "Floors Schematic"(w2178) -> ()
                  }
                }
              }
            }
          }
        }
      }
      event Value Change {
        n992 = event-data() -> ("NewVal"=w2220:bool)  [unwired: 1 in, 5 out]
        n993 = flat-sequence {
          tunnel: w2224 -> [w2233]
          tunnel: w2223 -> [w2232]
          tunnel: [w2231] -> w2222
          tunnel: [w2230] -> w2221
          tunnel: w2220 -> [w2229]
          tunnel: [w2228] -> w2219
          tunnel: w2218 -> [w2227]
          tunnel: [w2226] -> w2217
          tunnel: w2216 -> [w2225]
          frame #0 {
            n994 = case shown="True" w2229 {
              tunnel: w2233 -> [w2237 w2256]
              tunnel: w2232 -> [w2236 w2255]
              tunnel: [w2237 w2256] -> w2231
              tunnel: [w2236 w2255] -> w2230
              tunnel: [w2235 w2254] -> w2228
              tunnel: w2227 -> [w2235 w2245]
              tunnel: [w2234 w2253] -> w2226
              tunnel: w2225 -> [w2234 w2244]
              frame False {
              }
              frame True {
                n995 = control-ref of="Elevator Cabin"() -> (w2252:refnum<vi>)
                n996 = property class="Slide (strict)"(reference=w2252) -> ("Top"=w2251:i32)  [unwired: 1 in, 2 out]
                n997 = local read "Floors Schematic"() -> (w2249:T4)
                n998 = Preview Queue Element(queue=w2245, timeout in ms (-1)=1, error in (no error)=w2244) -> (timed out?=w2243:bool)  [unwired: 3 out]
                n999 = Unbundle By Name(w2249) -> ("Floor Position"=w2250:i16[])
                n1000 = Decrement(x=8 ("32bit integer")) -> (x-1=w2239:i32)
                n1001 = Index Array(array=w2250, index=w2239) -> (element=w2247:i16)
                n1002 = To Long Integer(number=w2247) -> (32bit integer=w2248:i32)
                n1003 = Not Equal?(x=w2248, y=w2251) -> (x != y?=w2242:bool)
                n1004 = Select(t=TRUE, s=w2243, f=w2242) -> (s? t:f=w2240:bool)
                n1005 = case shown="False" w2240 {
                  tunnel: w2245 -> [w2258 w2270]
                  tunnel: w2244 -> [w2257 w2269]
                  tunnel: [w2258 w2268] -> w2254
                  tunnel: [w2257 w2267] -> w2253
                  frame True {
                    n1006 = local read "Elevator Automate"() -> (w2260:T2)
                    n1007 = Bundle By Name(cluster=w2260, "Add Floor\nto Queue"=TRUE ("Add to Queue")) -> (w2261:T2)
                    n1008 = local write "Elevator Automate"(w2261) -> ()
                  }
                  frame False {
                    n1009 = local read "Elevator Automate"() -> (w2274:T2)
                    n1010 = Unbundle By Name(w2274) -> ("Elevator Command"=w2273:T1)
                    n1011 = Equal?(x=w2273, y=Elevator_Command."Close Doors") -> (x = y?=w2271:bool)
                    n1012 = case shown="True" w2271 {
                      tunnel: w2270 -> [w2287 w2302]
                      tunnel: w2269 -> [w2286 w2301]
                      tunnel: [w2285 w2302] -> w2268
                      tunnel: [w2284 w2301] -> w2267
                      tunnel: [FALSE ("Call 12") FALSE ("Call 12")] -> w2262
                      frame True {
                        w2297 = T8 20 items=["Floor Length"=48, "Sum of Floors"=12, "Floor Step in ms"=63, "Elevator Door Step in ms"=30, "Global Wait in ms"=20, "Event Wait in ms"=100] ("Elevator Constants")
                        n1013 = local read "Elevator Automate"() -> (w2296:T2)
                        n1014 = Flush Queue(queue=w2287, error in (no error)=w2286) -> (queue out=w2283:refnum<queue>, error out=w2282:errorcluster)  [unwired: 1 out]
                        n1015 = To Long Integer(number=w2297) -> (32bit integer=w2298:i32)
                        n1016 = Preview Queue Element(queue=w2283, timeout in ms (-1)=w2298, error in (no error)=w2282) -> (queue out=w2277:refnum<queue>, timed out?=w2276:bool, error out=w2278:errorcluster)  [unwired: 1 out]
                        n1017 = Bundle By Name(cluster=w2296, "Forced Stop"=w2276) -> (w2295:T2)
                        n1018 = Enqueue Element(queue=w2277, element=Elevator_Command."Open Doors", error in (no error)=w2278) -> (queue out=w2280:refnum<queue>, error out=w2279:errorcluster)  [unwired: 1 in, 1 out]
                        n1019 = local write "Elevator Automate"(w2295) -> ()
                        n1020 = Enqueue Element(queue=w2280, element=Elevator_Command."Long Delay", error in (no error)=w2279) -> (queue out=w2294:refnum<queue>, error out=w2293:errorcluster)  [unwired: 1 in, 1 out]
                        n1021 = Enqueue Element(queue=w2294, element=Elevator_Command."Close Doors", error in (no error)=w2293) -> (queue out=w2292:refnum<queue>, error out=w2291:errorcluster)  [unwired: 1 in, 1 out]
                        n1022 = Enqueue Element(queue=w2292, element=Elevator_Command."Idle", error in (no error)=w2291) -> (queue out=w2285:refnum<queue>, error out=w2284:errorcluster)  [unwired: 1 in, 1 out]
                      }
                      frame False {
                        n1023 = Wait (ms)(milliseconds to wait=u32 250) -> ()  [unwired: 1 out]
                      }
                    }
                    n1024 = local read "Floors Schematic"() -> (w2266:T4)
                    n1025 = local read "Elevator Panel"() -> (w2264:T3)
                    n1026 = Bundle By Name(cluster=w2266, "Call 8"=w2262) -> (w2265:T4)
                    n1027 = Bundle By Name(cluster=w2264, "Floor 8"=w2262) -> (w2263:T3)
                    n1028 = local write "Elevator Panel"(w2263) -> ()
                    n1029 = local write "Floors Schematic"(w2265) -> ()
                  }
                }
              }
            }
          }
        }
      }
      event Value Change {
        n1030 = event-data() -> ("NewVal"=w2307:bool)  [unwired: 1 in, 5 out]
        n1031 = flat-sequence {
          tunnel: w2311 -> [w2320]
          tunnel: w2310 -> [w2319]
          tunnel: [w2318] -> w2309
          tunnel: [w2317] -> w2308
          tunnel: w2307 -> [w2316]
          tunnel: [w2315] -> w2306
          tunnel: w2305 -> [w2314]
          tunnel: [w2313] -> w2304
          tunnel: w2303 -> [w2312]
          frame #0 {
            n1032 = case shown="True" w2316 {
              tunnel: w2320 -> [w2324 w2343]
              tunnel: w2319 -> [w2323 w2342]
              tunnel: [w2324 w2343] -> w2318
              tunnel: [w2323 w2342] -> w2317
              tunnel: [w2322 w2341] -> w2315
              tunnel: w2314 -> [w2322 w2332]
              tunnel: [w2321 w2340] -> w2313
              tunnel: w2312 -> [w2321 w2331]
              frame False {
              }
              frame True {
                n1033 = control-ref of="Elevator Cabin"() -> (w2339:refnum<vi>)
                n1034 = property class="Slide (strict)"(reference=w2339) -> ("Top"=w2338:i32)  [unwired: 1 in, 2 out]
                n1035 = local read "Floors Schematic"() -> (w2336:T4)
                n1036 = Preview Queue Element(queue=w2332, timeout in ms (-1)=1, error in (no error)=w2331) -> (timed out?=w2330:bool)  [unwired: 3 out]
                n1037 = Unbundle By Name(w2336) -> ("Floor Position"=w2337:i16[])
                n1038 = Decrement(x=9 ("32bit integer")) -> (x-1=w2326:i32)
                n1039 = Index Array(array=w2337, index=w2326) -> (element=w2334:i16)
                n1040 = To Long Integer(number=w2334) -> (32bit integer=w2335:i32)
                n1041 = Not Equal?(x=w2335, y=w2338) -> (x != y?=w2329:bool)
                n1042 = Select(t=TRUE, s=w2330, f=w2329) -> (s? t:f=w2327:bool)
                n1043 = case shown="False" w2327 {
                  tunnel: w2332 -> [w2345 w2357]
                  tunnel: w2331 -> [w2344 w2356]
                  tunnel: [w2345 w2355] -> w2341
                  tunnel: [w2344 w2354] -> w2340
                  frame True {
                    n1044 = local read "Elevator Automate"() -> (w2347:T2)
                    n1045 = Bundle By Name(cluster=w2347, "Add Floor\nto Queue"=TRUE ("Add to Queue")) -> (w2348:T2)
                    n1046 = local write "Elevator Automate"(w2348) -> ()
                  }
                  frame False {
                    n1047 = local read "Elevator Automate"() -> (w2361:T2)
                    n1048 = Unbundle By Name(w2361) -> ("Elevator Command"=w2360:T1)
                    n1049 = Equal?(x=w2360, y=Elevator_Command."Close Doors") -> (x = y?=w2358:bool)
                    n1050 = case shown="True" w2358 {
                      tunnel: w2357 -> [w2374 w2389]
                      tunnel: w2356 -> [w2373 w2388]
                      tunnel: [w2372 w2389] -> w2355
                      tunnel: [w2371 w2388] -> w2354
                      tunnel: [FALSE ("Call 12") FALSE ("Call 12")] -> w2349
                      frame True {
                        w2384 = T8 20 items=["Floor Length"=48, "Sum of Floors"=12, "Floor Step in ms"=63, "Elevator Door Step in ms"=30, "Global Wait in ms"=20, "Event Wait in ms"=100] ("Elevator Constants")
                        n1051 = local read "Elevator Automate"() -> (w2383:T2)
                        n1052 = Flush Queue(queue=w2374, error in (no error)=w2373) -> (queue out=w2370:refnum<queue>, error out=w2369:errorcluster)  [unwired: 1 out]
                        n1053 = To Long Integer(number=w2384) -> (32bit integer=w2385:i32)
                        n1054 = Preview Queue Element(queue=w2370, timeout in ms (-1)=w2385, error in (no error)=w2369) -> (queue out=w2364:refnum<queue>, timed out?=w2363:bool, error out=w2365:errorcluster)  [unwired: 1 out]
                        n1055 = Bundle By Name(cluster=w2383, "Forced Stop"=w2363) -> (w2382:T2)
                        n1056 = Enqueue Element(queue=w2364, element=Elevator_Command."Open Doors", error in (no error)=w2365) -> (queue out=w2367:refnum<queue>, error out=w2366:errorcluster)  [unwired: 1 in, 1 out]
                        n1057 = local write "Elevator Automate"(w2382) -> ()
                        n1058 = Enqueue Element(queue=w2367, element=Elevator_Command."Long Delay", error in (no error)=w2366) -> (queue out=w2381:refnum<queue>, error out=w2380:errorcluster)  [unwired: 1 in, 1 out]
                        n1059 = Enqueue Element(queue=w2381, element=Elevator_Command."Close Doors", error in (no error)=w2380) -> (queue out=w2379:refnum<queue>, error out=w2378:errorcluster)  [unwired: 1 in, 1 out]
                        n1060 = Enqueue Element(queue=w2379, element=Elevator_Command."Idle", error in (no error)=w2378) -> (queue out=w2372:refnum<queue>, error out=w2371:errorcluster)  [unwired: 1 in, 1 out]
                      }
                      frame False {
                        n1061 = Wait (ms)(milliseconds to wait=u32 250) -> ()  [unwired: 1 out]
                      }
                    }
                    n1062 = local read "Floors Schematic"() -> (w2353:T4)
                    n1063 = local read "Elevator Panel"() -> (w2351:T3)
                    n1064 = Bundle By Name(cluster=w2353, "Call 9"=w2349) -> (w2352:T4)
                    n1065 = Bundle By Name(cluster=w2351, "Floor 9"=w2349) -> (w2350:T3)
                    n1066 = local write "Elevator Panel"(w2350) -> ()
                    n1067 = local write "Floors Schematic"(w2352) -> ()
                  }
                }
              }
            }
          }
        }
      }
      event Value Change {
        n1068 = event-data() -> ("NewVal"=w2394:bool)  [unwired: 1 in, 5 out]
        n1069 = flat-sequence {
          tunnel: w2398 -> [w2407]
          tunnel: w2397 -> [w2406]
          tunnel: [w2405] -> w2396
          tunnel: [w2404] -> w2395
          tunnel: w2394 -> [w2403]
          tunnel: [w2402] -> w2393
          tunnel: w2392 -> [w2401]
          tunnel: [w2400] -> w2391
          tunnel: w2390 -> [w2399]
          frame #0 {
            n1070 = case shown="True" w2403 {
              tunnel: w2407 -> [w2411 w2430]
              tunnel: w2406 -> [w2410 w2429]
              tunnel: [w2411 w2430] -> w2405
              tunnel: [w2410 w2429] -> w2404
              tunnel: [w2409 w2428] -> w2402
              tunnel: w2401 -> [w2409 w2419]
              tunnel: [w2408 w2427] -> w2400
              tunnel: w2399 -> [w2408 w2418]
              frame False {
              }
              frame True {
                n1071 = control-ref of="Elevator Cabin"() -> (w2426:refnum<vi>)
                n1072 = property class="Slide (strict)"(reference=w2426) -> ("Top"=w2425:i32)  [unwired: 1 in, 2 out]
                n1073 = local read "Floors Schematic"() -> (w2423:T4)
                n1074 = Preview Queue Element(queue=w2419, timeout in ms (-1)=1, error in (no error)=w2418) -> (timed out?=w2417:bool)  [unwired: 3 out]
                n1075 = Unbundle By Name(w2423) -> ("Floor Position"=w2424:i16[])
                n1076 = Decrement(x=10 ("32bit integer")) -> (x-1=w2413:i32)
                n1077 = Index Array(array=w2424, index=w2413) -> (element=w2421:i16)
                n1078 = To Long Integer(number=w2421) -> (32bit integer=w2422:i32)
                n1079 = Not Equal?(x=w2422, y=w2425) -> (x != y?=w2416:bool)
                n1080 = Select(t=TRUE, s=w2417, f=w2416) -> (s? t:f=w2414:bool)
                n1081 = case shown="False" w2414 {
                  tunnel: w2419 -> [w2432 w2444]
                  tunnel: w2418 -> [w2431 w2443]
                  tunnel: [w2432 w2442] -> w2428
                  tunnel: [w2431 w2441] -> w2427
                  frame True {
                    n1082 = local read "Elevator Automate"() -> (w2434:T2)
                    n1083 = Bundle By Name(cluster=w2434, "Add Floor\nto Queue"=TRUE ("Add to Queue")) -> (w2435:T2)
                    n1084 = local write "Elevator Automate"(w2435) -> ()
                  }
                  frame False {
                    n1085 = local read "Elevator Automate"() -> (w2448:T2)
                    n1086 = Unbundle By Name(w2448) -> ("Elevator Command"=w2447:T1)
                    n1087 = Equal?(x=w2447, y=Elevator_Command."Close Doors") -> (x = y?=w2445:bool)
                    n1088 = case shown="True" w2445 {
                      tunnel: w2444 -> [w2461 w2476]
                      tunnel: w2443 -> [w2460 w2475]
                      tunnel: [w2459 w2476] -> w2442
                      tunnel: [w2458 w2475] -> w2441
                      tunnel: [FALSE ("Call 12") FALSE ("Call 12")] -> w2436
                      frame True {
                        w2471 = T8 20 items=["Floor Length"=48, "Sum of Floors"=12, "Floor Step in ms"=63, "Elevator Door Step in ms"=30, "Global Wait in ms"=20, "Event Wait in ms"=100] ("Elevator Constants")
                        n1089 = local read "Elevator Automate"() -> (w2470:T2)
                        n1090 = Flush Queue(queue=w2461, error in (no error)=w2460) -> (queue out=w2457:refnum<queue>, error out=w2456:errorcluster)  [unwired: 1 out]
                        n1091 = To Long Integer(number=w2471) -> (32bit integer=w2472:i32)
                        n1092 = Preview Queue Element(queue=w2457, timeout in ms (-1)=w2472, error in (no error)=w2456) -> (queue out=w2451:refnum<queue>, timed out?=w2450:bool, error out=w2452:errorcluster)  [unwired: 1 out]
                        n1093 = Bundle By Name(cluster=w2470, "Forced Stop"=w2450) -> (w2469:T2)
                        n1094 = Enqueue Element(queue=w2451, element=Elevator_Command."Open Doors", error in (no error)=w2452) -> (queue out=w2454:refnum<queue>, error out=w2453:errorcluster)  [unwired: 1 in, 1 out]
                        n1095 = local write "Elevator Automate"(w2469) -> ()
                        n1096 = Enqueue Element(queue=w2454, element=Elevator_Command."Long Delay", error in (no error)=w2453) -> (queue out=w2468:refnum<queue>, error out=w2467:errorcluster)  [unwired: 1 in, 1 out]
                        n1097 = Enqueue Element(queue=w2468, element=Elevator_Command."Close Doors", error in (no error)=w2467) -> (queue out=w2466:refnum<queue>, error out=w2465:errorcluster)  [unwired: 1 in, 1 out]
                        n1098 = Enqueue Element(queue=w2466, element=Elevator_Command."Idle", error in (no error)=w2465) -> (queue out=w2459:refnum<queue>, error out=w2458:errorcluster)  [unwired: 1 in, 1 out]
                      }
                      frame False {
                        n1099 = Wait (ms)(milliseconds to wait=u32 250) -> ()  [unwired: 1 out]
                      }
                    }
                    n1100 = local read "Floors Schematic"() -> (w2440:T4)
                    n1101 = local read "Elevator Panel"() -> (w2438:T3)
                    n1102 = Bundle By Name(cluster=w2440, "Call 10"=w2436) -> (w2439:T4)
                    n1103 = Bundle By Name(cluster=w2438, "Floor 10"=w2436) -> (w2437:T3)
                    n1104 = local write "Elevator Panel"(w2437) -> ()
                    n1105 = local write "Floors Schematic"(w2439) -> ()
                  }
                }
              }
            }
          }
        }
      }
      event Value Change {
        n1106 = event-data() -> ("NewVal"=w2481:bool)  [unwired: 1 in, 5 out]
        n1107 = flat-sequence {
          tunnel: w2485 -> [w2494]
          tunnel: w2484 -> [w2493]
          tunnel: [w2492] -> w2483
          tunnel: [w2491] -> w2482
          tunnel: w2481 -> [w2490]
          tunnel: [w2489] -> w2480
          tunnel: w2479 -> [w2488]
          tunnel: [w2487] -> w2478
          tunnel: w2477 -> [w2486]
          frame #0 {
            n1108 = case shown="True" w2490 {
              tunnel: w2494 -> [w2498 w2517]
              tunnel: w2493 -> [w2497 w2516]
              tunnel: [w2498 w2517] -> w2492
              tunnel: [w2497 w2516] -> w2491
              tunnel: [w2496 w2515] -> w2489
              tunnel: w2488 -> [w2496 w2506]
              tunnel: [w2495 w2514] -> w2487
              tunnel: w2486 -> [w2495 w2505]
              frame False {
              }
              frame True {
                n1109 = control-ref of="Elevator Cabin"() -> (w2513:refnum<vi>)
                n1110 = property class="Slide (strict)"(reference=w2513) -> ("Top"=w2512:i32)  [unwired: 1 in, 2 out]
                n1111 = local read "Floors Schematic"() -> (w2510:T4)
                n1112 = Preview Queue Element(queue=w2506, timeout in ms (-1)=1, error in (no error)=w2505) -> (timed out?=w2504:bool)  [unwired: 3 out]
                n1113 = Unbundle By Name(w2510) -> ("Floor Position"=w2511:i16[])
                n1114 = Decrement(x=11 ("32bit integer")) -> (x-1=w2500:i32)
                n1115 = Index Array(array=w2511, index=w2500) -> (element=w2508:i16)
                n1116 = To Long Integer(number=w2508) -> (32bit integer=w2509:i32)
                n1117 = Not Equal?(x=w2509, y=w2512) -> (x != y?=w2503:bool)
                n1118 = Select(t=TRUE, s=w2504, f=w2503) -> (s? t:f=w2501:bool)
                n1119 = case shown="False" w2501 {
                  tunnel: w2506 -> [w2519 w2531]
                  tunnel: w2505 -> [w2518 w2530]
                  tunnel: [w2519 w2529] -> w2515
                  tunnel: [w2518 w2528] -> w2514
                  frame True {
                    n1120 = local read "Elevator Automate"() -> (w2521:T2)
                    n1121 = Bundle By Name(cluster=w2521, "Add Floor\nto Queue"=TRUE ("Add to Queue")) -> (w2522:T2)
                    n1122 = local write "Elevator Automate"(w2522) -> ()
                  }
                  frame False {
                    n1123 = local read "Elevator Automate"() -> (w2535:T2)
                    n1124 = Unbundle By Name(w2535) -> ("Elevator Command"=w2534:T1)
                    n1125 = Equal?(x=w2534, y=Elevator_Command."Close Doors") -> (x = y?=w2532:bool)
                    n1126 = case shown="False" w2532 {
                      tunnel: w2531 -> [w2548 w2563]
                      tunnel: w2530 -> [w2547 w2562]
                      tunnel: [w2546 w2563] -> w2529
                      tunnel: [w2545 w2562] -> w2528
                      tunnel: [FALSE ("Call 12") FALSE ("Call 12")] -> w2523
                      frame True {
                        w2558 = T8 20 items=["Floor Length"=48, "Sum of Floors"=12, "Floor Step in ms"=63, "Elevator Door Step in ms"=30, "Global Wait in ms"=20, "Event Wait in ms"=100] ("Elevator Constants")
                        n1127 = local read "Elevator Automate"() -> (w2557:T2)
                        n1128 = Flush Queue(queue=w2548, error in (no error)=w2547) -> (queue out=w2544:refnum<queue>, error out=w2543:errorcluster)  [unwired: 1 out]
                        n1129 = To Long Integer(number=w2558) -> (32bit integer=w2559:i32)
                        n1130 = Preview Queue Element(queue=w2544, timeout in ms (-1)=w2559, error in (no error)=w2543) -> (queue out=w2538:refnum<queue>, timed out?=w2537:bool, error out=w2539:errorcluster)  [unwired: 1 out]
                        n1131 = Bundle By Name(cluster=w2557, "Forced Stop"=w2537) -> (w2556:T2)
                        n1132 = Enqueue Element(queue=w2538, element=Elevator_Command."Open Doors", error in (no error)=w2539) -> (queue out=w2541:refnum<queue>, error out=w2540:errorcluster)  [unwired: 1 in, 1 out]
                        n1133 = local write "Elevator Automate"(w2556) -> ()
                        n1134 = Enqueue Element(queue=w2541, element=Elevator_Command."Long Delay", error in (no error)=w2540) -> (queue out=w2555:refnum<queue>, error out=w2554:errorcluster)  [unwired: 1 in, 1 out]
                        n1135 = Enqueue Element(queue=w2555, element=Elevator_Command."Close Doors", error in (no error)=w2554) -> (queue out=w2553:refnum<queue>, error out=w2552:errorcluster)  [unwired: 1 in, 1 out]
                        n1136 = Enqueue Element(queue=w2553, element=Elevator_Command."Idle", error in (no error)=w2552) -> (queue out=w2546:refnum<queue>, error out=w2545:errorcluster)  [unwired: 1 in, 1 out]
                      }
                      frame False {
                        n1137 = Wait (ms)(milliseconds to wait=u32 250) -> ()  [unwired: 1 out]
                      }
                    }
                    n1138 = local read "Floors Schematic"() -> (w2527:T4)
                    n1139 = local read "Elevator Panel"() -> (w2525:T3)
                    n1140 = Bundle By Name(cluster=w2527, "Call 11"=w2523) -> (w2526:T4)
                    n1141 = Bundle By Name(cluster=w2525, "Floor 11"=w2523) -> (w2524:T3)
                    n1142 = local write "Elevator Panel"(w2524) -> ()
                    n1143 = local write "Floors Schematic"(w2526) -> ()
                  }
                }
              }
            }
          }
        }
      }
      event Value Change {
        n1144 = event-data() -> ("NewVal"=w2568:bool)  [unwired: 1 in, 5 out]
        n1145 = flat-sequence {
          tunnel: w2572 -> [w2581]
          tunnel: w2571 -> [w2580]
          tunnel: [w2579] -> w2570
          tunnel: [w2578] -> w2569
          tunnel: w2568 -> [w2577]
          tunnel: [w2576] -> w2567
          tunnel: w2566 -> [w2575]
          tunnel: [w2574] -> w2565
          tunnel: w2564 -> [w2573]
          frame #0 {
            n1146 = case shown="True" w2577 {
              tunnel: w2581 -> [w2585 w2604]
              tunnel: w2580 -> [w2584 w2603]
              tunnel: [w2585 w2604] -> w2579
              tunnel: [w2584 w2603] -> w2578
              tunnel: [w2583 w2602] -> w2576
              tunnel: w2575 -> [w2583 w2593]
              tunnel: [w2582 w2601] -> w2574
              tunnel: w2573 -> [w2582 w2592]
              frame False {
              }
              frame True {
                n1147 = control-ref of="Elevator Cabin"() -> (w2600:refnum<vi>)
                n1148 = property class="Slide (strict)"(reference=w2600) -> ("Top"=w2599:i32)  [unwired: 1 in, 2 out]
                n1149 = local read "Floors Schematic"() -> (w2597:T4)
                n1150 = Preview Queue Element(queue=w2593, timeout in ms (-1)=1, error in (no error)=w2592) -> (timed out?=w2591:bool)  [unwired: 3 out]
                n1151 = Unbundle By Name(w2597) -> ("Floor Position"=w2598:i16[])
                n1152 = Decrement(x=12 ("32bit integer")) -> (x-1=w2587:i32)
                n1153 = Index Array(array=w2598, index=w2587) -> (element=w2595:i16)
                n1154 = To Long Integer(number=w2595) -> (32bit integer=w2596:i32)
                n1155 = Not Equal?(x=w2596, y=w2599) -> (x != y?=w2590:bool)
                n1156 = Select(t=TRUE, s=w2591, f=w2590) -> (s? t:f=w2588:bool)
                n1157 = case shown="False" w2588 {
                  tunnel: w2593 -> [w2606 w2618]
                  tunnel: w2592 -> [w2605 w2617]
                  tunnel: [w2606 w2616] -> w2602
                  tunnel: [w2605 w2615] -> w2601
                  frame True {
                    n1158 = local read "Elevator Automate"() -> (w2608:T2)
                    n1159 = Bundle By Name(cluster=w2608, "Add Floor\nto Queue"=TRUE ("Add to Queue")) -> (w2609:T2)
                    n1160 = local write "Elevator Automate"(w2609) -> ()
                  }
                  frame False {
                    n1161 = local read "Elevator Automate"() -> (w2622:T2)
                    n1162 = Unbundle By Name(w2622) -> ("Elevator Command"=w2621:T1)
                    n1163 = Equal?(x=w2621, y=Elevator_Command."Close Doors") -> (x = y?=w2619:bool)
                    n1164 = case shown="True" w2619 {
                      tunnel: w2618 -> [w2635 w2650]
                      tunnel: w2617 -> [w2634 w2649]
                      tunnel: [w2633 w2650] -> w2616
                      tunnel: [w2632 w2649] -> w2615
                      tunnel: [FALSE ("Call 12") FALSE ("Call 12")] -> w2610
                      frame True {
                        w2645 = T8 20 items=["Floor Length"=48, "Sum of Floors"=12, "Floor Step in ms"=63, "Elevator Door Step in ms"=30, "Global Wait in ms"=20, "Event Wait in ms"=100] ("Elevator Constants")
                        n1165 = local read "Elevator Automate"() -> (w2644:T2)
                        n1166 = Flush Queue(queue=w2635, error in (no error)=w2634) -> (queue out=w2631:refnum<queue>, error out=w2630:errorcluster)  [unwired: 1 out]
                        n1167 = To Long Integer(number=w2645) -> (32bit integer=w2646:i32)
                        n1168 = Preview Queue Element(queue=w2631, timeout in ms (-1)=w2646, error in (no error)=w2630) -> (queue out=w2625:refnum<queue>, timed out?=w2624:bool, error out=w2626:errorcluster)  [unwired: 1 out]
                        n1169 = Bundle By Name(cluster=w2644, "Forced Stop"=w2624) -> (w2643:T2)
                        n1170 = Enqueue Element(queue=w2625, element=Elevator_Command."Open Doors", error in (no error)=w2626) -> (queue out=w2628:refnum<queue>, error out=w2627:errorcluster)  [unwired: 1 in, 1 out]
                        n1171 = local write "Elevator Automate"(w2643) -> ()
                        n1172 = Enqueue Element(queue=w2628, element=Elevator_Command."Long Delay", error in (no error)=w2627) -> (queue out=w2642:refnum<queue>, error out=w2641:errorcluster)  [unwired: 1 in, 1 out]
                        n1173 = Enqueue Element(queue=w2642, element=Elevator_Command."Close Doors", error in (no error)=w2641) -> (queue out=w2640:refnum<queue>, error out=w2639:errorcluster)  [unwired: 1 in, 1 out]
                        n1174 = Enqueue Element(queue=w2640, element=Elevator_Command."Idle", error in (no error)=w2639) -> (queue out=w2633:refnum<queue>, error out=w2632:errorcluster)  [unwired: 1 in, 1 out]
                      }
                      frame False {
                        n1175 = Wait (ms)(milliseconds to wait=u32 250) -> ()  [unwired: 1 out]
                      }
                    }
                    n1176 = local read "Floors Schematic"() -> (w2614:T4)
                    n1177 = local read "Elevator Panel"() -> (w2612:T3)
                    n1178 = Bundle By Name(cluster=w2614, "Call 12"=w2610) -> (w2613:T4)
                    n1179 = Bundle By Name(cluster=w2612, "Floor 12"=w2610) -> (w2611:T3)
                    n1180 = local write "Elevator Panel"(w2611) -> ()
                    n1181 = local write "Floors Schematic"(w2613) -> ()
                  }
                }
              }
            }
          }
        }
      }
      event Value Change {
        # "Закрытие кабины лифта"
        n1182 = event-data() -> ("NewVal"=w2657:bool)  [unwired: 1 in, 5 out]
        n1183 = flat-sequence {
          tunnel: w2657 -> [w2662]
          tunnel: w2656 -> [w2661]
          tunnel: [w2660] -> w2655
          tunnel: w2654 -> [w2659]
          tunnel: [w2658] -> w2653
          frame #0 {
            n1184 = case shown="True" w2662 {
              tunnel: [w2664 w2668] -> w2660
              tunnel: [w2663 w2665] -> w2658
              tunnel: w2661 -> [w2664 w2672]
              tunnel: w2659 -> [w2663 w2671]
              frame False {
              }
              frame True {
                # "Проверка, что лифт на этаже"
                n1185 = local read "Floors Schematic"() -> (w2678:T4)
                n1186 = local read "Elevator Automate"() -> (w2680:T2)
                n1187 = Unbundle By Name(w2680) -> ("Elevator Command"=w2682:T1)
                n1188 = control-ref of="Elevator Cabin"() -> (w2679:refnum<vi>)
                n1189 = property class="Slide (strict)"(reference=w2679) -> ("Top"=w2676:i32)  [unwired: 1 in, 2 out]
                n1190 = Equal?(x=w2682, y=Elevator_Command."Long Delay") -> (x = y?=w2685:bool)
                n1191 = Equal?(x=w2682, y=Elevator_Command."Idle") -> (x = y?=w2683:bool)
                n1192 = Unbundle By Name(w2678) -> ("Floor Position"=w2677:i16[])
                n1193 = Compound Arithmetic op=OR(w2685, w2683) -> (w2674:bool)
                n1194 = while {
                  tunnel: w2677 -> [w2699]
                  tunnel: w2676 -> [w2697]
                  tunnel: [w2694] -> w2673
                  i -> [w2695]
                  stop <- w2696 stop-if-true
                  n1195 = Index Array(array=w2699, index=w2695) -> (element=w2700:i16)
                  n1196 = To Long Integer(number=w2700) -> (32bit integer=w2698:i32)
                  n1197 = Less Or Equal?(x=w2698, y=w2697) -> (x <= y?=w2696:bool)
                  n1198 = Equal?(x=w2697, y=w2698) -> (x = y?=w2701:bool)
                  n1199 = case shown="True" w2701 {
                    selector: w2701 -> [w2702 w2703]
                    tunnel: [w2702 w2703] -> w2694
                    frame False {
                    }
                    frame True {
                    }
                  }
                }
                n1200 = And(x=w2674, y=w2673) -> (x .and. y?=w2675:bool)
                n1201 = case shown="True" w2675 {
                  tunnel: [w2705 w2712] -> w2669
                  tunnel: [w2704 w2711] -> w2666
                  tunnel: w2680 -> [_ w2710]
                  tunnel: w2672 -> [w2705 w2707]
                  tunnel: w2671 -> [w2704 w2706]
                  frame False {
                  }
                  frame True {
                    n1202 = flat-sequence {
                      tunnel: w2710 -> [w2718]
                      tunnel: [w2716] -> w2709
                      tunnel: [w2715] -> w2708
                      tunnel: w2707 -> [w2716]
                      tunnel: w2706 -> [w2715]
                      tunnel: [w2724] -> w2712
                      tunnel: [w2723] -> w2711
                      tunnel: w2709 -> [w2720]
                      tunnel: w2708 -> [w2719]
                      frame #0 {
                        n1203 = local read "# elements in Elevator Command Queue"() -> (w2714:i32)
                        n1204 = Not Equal To 0?(x=w2714) -> (x != 0?=w2713:bool)
                        n1205 = Bundle By Name(cluster=w2718, "Forced Stop"=w2713) -> (w2717:T2)
                        n1206 = local write "Elevator Automate"(w2717) -> ()
                      }
                      frame #1 {
                        n1207 = Flush Queue(queue=w2720, error in (no error)=w2719) -> (queue out=w2722:refnum<queue>, error out=w2721:errorcluster)  [unwired: 1 out]
                        n1208 = Enqueue Element(queue=w2722, element=Elevator_Command."Close Doors", error in (no error)=w2721) -> (queue out=w2727:refnum<queue>, error out=w2726:errorcluster)  [unwired: 1 in, 1 out]
                        n1209 = Enqueue Element(queue=w2727, element=Elevator_Command."Idle", error in (no error)=w2726) -> (queue out=w2724:refnum<queue>, error out=w2723:errorcluster)  [unwired: 1 in, 1 out]
                      }
                    }
                  }
                }
                n1210 = flat-sequence {
                  tunnel: [w2687] -> w2670
                  tunnel: w2669 -> [w2687]
                  tunnel: [w2686] -> w2667
                  tunnel: w2666 -> [w2686]
                  tunnel: w2670 -> [w2690]
                  tunnel: [w2690] -> w2668
                  tunnel: w2667 -> [w2689]
                  tunnel: [w2689] -> w2665
                  frame #0 {
                    n1211 = Wait (ms)(milliseconds to wait=u32 250) -> ()  [unwired: 1 out]
                  }
                  frame #1 {
                    n1212 = local read "Elevator Panel"() -> (w2693:T3)
                    n1213 = Bundle By Name(cluster=w2693, "Close Doors"=FALSE ("Open Doors")) -> (w2692:T3)
                    n1214 = local write "Elevator Panel"(w2692) -> ()
                  }
                }
              }
            }
          }
        }
      }
      event Value Change {
        # "Открытие кабины лифта"
        n1215 = event-data() -> ("NewVal"=w2735:bool)  [unwired: 1 in, 5 out]
        n1216 = flat-sequence {
          tunnel: w2735 -> [w2740]
          tunnel: w2734 -> [w2739]
          tunnel: w2733 -> [w2738]
          tunnel: [w2737] -> w2732
          tunnel: [w2736] -> w2731
          frame #0 {
            n1217 = case shown="True" w2740 {
              tunnel: [w2742 w2744] -> w2737
              tunnel: [w2741 w2743] -> w2736
              tunnel: w2739 -> [w2742 w2762]
              tunnel: w2738 -> [w2741 w2761]
              frame False {
              }
              frame True {
                # "Проверка, что лифт не между этажами"
                n1218 = local read "Elevator Automate"() -> (w2760:T2)
                n1219 = Unbundle By Name(w2760) -> ("Elevator Command"=w2758:T1)
                n1220 = Equal?(x=w2758, y=Elevator_Command."Long Delay") -> (x = y?=w2765:bool)
                n1221 = Equal?(x=w2758, y=Elevator_Command."Close Doors") -> (x = y?=w2757:bool)
                n1222 = Equal?(x=w2758, y=Elevator_Command."Idle") -> (x = y?=w2756:bool)
                n1223 = Compound Arithmetic op=OR(w2765, w2757, w2756) -> (w2749:bool)
                n1224 = local read "Floors Schematic"() -> (w2754:T4)
                n1225 = control-ref of="Elevator Cabin"() -> (w2755:refnum<vi>)
                n1226 = property class="Slide (strict)"(reference=w2755) -> ("Top"=w2752:i32)  [unwired: 1 in, 2 out]
                n1227 = Unbundle By Name(w2754) -> ("Floor Position"=w2753:i16[])
                n1228 = while {
                  tunnel: w2753 -> [w2779]
                  tunnel: w2752 -> [w2777]
                  tunnel: [w2774] -> w2750
                  i -> [w2775]
                  stop <- w2776 stop-if-true
                  n1229 = Index Array(array=w2779, index=w2775) -> (element=w2780:i16)
                  n1230 = To Long Integer(number=w2780) -> (32bit integer=w2778:i32)
                  n1231 = Less Or Equal?(x=w2778, y=w2777) -> (x <= y?=w2776:bool)
                  n1232 = Equal?(x=w2777, y=w2778) -> (x = y?=w2781:bool)
                  n1233 = case shown="True" w2781 {
                    selector: w2781 -> [w2782 w2783]
                    tunnel: [w2782 w2783] -> w2774
                    frame False {
                    }
                    frame True {
                    }
                  }
                }
                n1234 = And(x=w2750, y=w2749) -> (x .and. y?=w2751:bool)
                n1235 = case shown="True" w2751 {
                  selector: w2751 -> [_ w2788]
                  tunnel: w2762 -> [w2785 w2791]
                  tunnel: w2761 -> [w2784 w2790]
                  tunnel: [w2785 w2793] -> w2748
                  tunnel: [w2784 w2792] -> w2747
                  tunnel: w2760 -> [_ w2787]
                  frame False {
                  }
                  frame True {
                    n1236 = flat-sequence {
                      tunnel: w2790 -> [w2796]
                      tunnel: w2791 -> [w2797]
                      tunnel: [w2797] -> w2789
                      tunnel: w2788 -> [_]
                      tunnel: w2787 -> [w2798]
                      tunnel: [w2796] -> w2786
                      tunnel: [w2801] -> w2793
                      tunnel: [w2800] -> w2792
                      tunnel: w2789 -> [w2812]
                      tunnel: w2786 -> [w2811]
                      frame #0 {
                        n1237 = local read "# elements in Elevator Command Queue"() -> (w2795:i32)
                        n1238 = Not Equal To 0?(x=w2795) -> (x != 0?=w2794:bool)
                        n1239 = Bundle By Name(cluster=w2798, "Forced Stop"=w2794) -> (w2799:T2)
                        n1240 = local write "Elevator Automate"(w2799) -> ()
                      }
                      frame #1 {
                        n1241 = Flush Queue(queue=w2812, error in (no error)=w2811) -> (queue out=w2814:refnum<queue>, error out=w2813:errorcluster)  [unwired: 1 out]
                        n1242 = Enqueue Element(queue=w2814, element=Elevator_Command."Open Doors", error in (no error)=w2813) -> (queue out=w2803:refnum<queue>, error out=w2802:errorcluster)  [unwired: 1 in, 1 out]
                        n1243 = Enqueue Element(queue=w2803, element=Elevator_Command."Long Delay", error in (no error)=w2802) -> (queue out=w2810:refnum<queue>, error out=w2809:errorcluster)  [unwired: 1 in, 1 out]
                        n1244 = Enqueue Element(queue=w2810, element=Elevator_Command."Close Doors", error in (no error)=w2809) -> (queue out=w2808:refnum<queue>, error out=w2807:errorcluster)  [unwired: 1 in, 1 out]
                        n1245 = Enqueue Element(queue=w2808, element=Elevator_Command."Idle", error in (no error)=w2807) -> (queue out=w2801:refnum<queue>, error out=w2800:errorcluster)  [unwired: 1 in, 1 out]
                      }
                    }
                  }
                }
                n1246 = flat-sequence {
                  tunnel: w2748 -> [w2767]
                  tunnel: w2747 -> [w2766]
                  tunnel: [w2767] -> w2746
                  tunnel: [w2766] -> w2745
                  tunnel: [w2770] -> w2744
                  tunnel: w2746 -> [w2770]
                  tunnel: [w2769] -> w2743
                  tunnel: w2745 -> [w2769]
                  frame #0 {
                    n1247 = Wait (ms)(milliseconds to wait=u32 250) -> ()  [unwired: 1 out]
                  }
                  frame #1 {
                    n1248 = local read "Elevator Panel"() -> (w2773:T3)
                    n1249 = Bundle By Name(cluster=w2773, "Open Doors"=FALSE) -> (w2772:T3)
                    n1250 = local write "Elevator Panel"(w2772) -> ()
                  }
                }
              }
            }
          }
        }
      }
    }
    n1251 = local read "Global Wait in ms"() -> (w1388:u32)
    n1252 = Wait (ms)(milliseconds to wait=w1388) -> ()  [unwired: 1 out]
    n1253 = local read "STOP"() -> (w1397:bool)
  }
  n1254 = while {
    tunnel: w2 -> [_]
    tunnel: w1 -> [_]
    shift-right: [w2817] -> _
    shift-left: w7 -> [w2824]
    shift-right: [w2816] -> _
    shift-left: w6 -> [w2823]
    tunnel: w5 -> [_]
    tunnel: w4 -> [_]
    stop <- "STOP" stop-if-true
    # "Задержка в случае отмены вызова и повторный запрос очереди вызовов"
    n1255 = local read "Global Wait in ms"() -> (w2821:u32)
    n1256 = To Long Integer(number=w2821) -> (32bit integer=w2820:i32)
    n1257 = Dequeue Element(queue=w2824, timeout in ms (-1)=w2820, error in (no error)=w2823) -> (queue out=w2818:refnum<queue>, element=w2822:T1, error out=w2819:errorcluster)  [unwired: 1 out]
    n1258 = case shown="\"Cancel Delay\"" w2822 {
      selector: w2822 -> [w2828 w2844 w2872 w2917 w3078 w3110 w3145 w3194 w3234]
      tunnel: [w2827 w2842 w2869 w2897 w3072 w3104 w3136 w3185 w3233] -> w2817
      tunnel: [w2826 w2841 w2868 w2905 w3071 w3103 w3135 w3184 w3232] -> w2816
      tunnel: w2818 -> [w2827 w2842 w2869 w2909 w3072 w3104 w3136 w3185 w3233]
      tunnel: w2819 -> [w2826 w2841 w2868 w2908 w3071 w3103 w3135 w3184 w3232]
      frame "Idle", Default {
        # "Команда ожидания"
        n1259 = flat-sequence {
          tunnel: w2828 -> [w2835]
          frame #0 {
            n1260 = local read "# elements in Elevator Floor Queue"() -> (w2830:i32)
            n1261 = local read "Elevator Automate"() -> (w2836:T2)
            n1262 = Bundle By Name(cluster=w2836, "Elevator Command"=w2835, "Forced Stop"=FALSE) -> (w2833:T2)
            n1263 = Equal To 0?(x=w2830) -> (x = 0?=w2831:bool)
            n1264 = case shown="True" w2831 {
              tunnel: w2833 -> [w2837 w2839]
              tunnel: [w2837 w2838] -> w2832
              frame False {
              }
              frame True {
                n1265 = Bundle By Name(cluster=w2839, "Elevator Status"=T9."Stand By") -> (w2838:T2)
              }
            }
            n1266 = local write "Elevator Automate"(w2832) -> ()
            n1267 = Wait (ms)(milliseconds to wait=u32 1) -> ()  [unwired: 1 out]
          }
        }
      }
      frame "Short Delay" {
        # "Короткая задержка ожидания"
        n1268 = flat-sequence {
          tunnel: w2844 -> [w2848]
          frame #0 {
            n1269 = local read "Elevator Automate"() -> (w2847:T2)
            n1270 = Bundle By Name(cluster=w2847, "Elevator Command"=w2848) -> (w2846:T2)
            n1271 = local write "Elevator Automate"(w2846) -> ()
          }
        }
        n1272 = while {
          tunnel: [w2858] -> w2845
          i -> [w2854]
          stop <- w2858 stop-if-true
          n1273 = flat-sequence {
            tunnel: w2854 -> [w2859]
            tunnel: [w2859] -> w2856
            tunnel: [w2860] -> w2857
            tunnel: w2856 -> [w2864]
            tunnel: [w2867] -> w2858
            tunnel: w2857 -> [w2867]
            frame #0 {
            }
            frame #1 {
              n1274 = local read "Elevator Automate"() -> (w2862:T2)
              n1275 = Unbundle By Name(w2862) -> ("Forced Stop"=w2861:bool)
              n1276 = Greater Or Equal?(x=w2864, y=2000) -> (x >= y?=w2865:bool)
              n1277 = local read "STOP"() -> (w2866:bool)
              n1278 = Compound Arithmetic op=OR(w2861, w2865, w2866) -> (w2860:bool)
            }
            frame #2 {
            }
          }
          n1279 = local write "Delay Timer"(w2854) -> ()
          n1280 = Wait (ms)(milliseconds to wait=u32 1) -> ()  [unwired: 1 out]
        }
        n1281 = flat-sequence {
          tunnel: w2845 -> [w2849]
          tunnel: [w2849] -> w2843
          tunnel: w2843 -> [w2851]
          frame #0 {
          }
          frame #1 {
            n1282 = Not(x=w2851) -> (.not. x?=w2852:bool)
            n1283 = local read "Elevator Automate"() -> (w2850:T2)
            n1284 = Bundle By Name(cluster=w2850, "Forced Stop"=w2852) -> (w2853:T2)
            n1285 = local write "Elevator Automate"(w2853) -> ()
          }
          frame #2 {
          }
        }
      }
      frame "Long Delay" {
        # "Долгая задержка ожидания"
        n1286 = flat-sequence {
          tunnel: w2872 -> [w2879]
          tunnel: [w2879] -> w2870
          tunnel: w2870 -> [w2880]
          frame #0 {
          }
          frame #1 {
            n1287 = local read "Elevator Automate"() -> (w2882:T2)
            n1288 = Bundle By Name(cluster=w2882, "Elevator Command"=w2880) -> (w2881:T2)
            n1289 = local write "Elevator Automate"(w2881) -> ()
          }
          frame #2 {
          }
        }
        n1290 = while {
          tunnel: [w2887] -> w2873
          i -> [w2883]
          stop <- w2887 stop-if-true
          n1291 = flat-sequence {
            tunnel: w2883 -> [w2888]
            tunnel: [w2888] -> w2885
            tunnel: [w2889] -> w2886
            tunnel: w2885 -> [w2893]
            tunnel: [w2896] -> w2887
            tunnel: w2886 -> [w2896]
            frame #0 {
            }
            frame #1 {
              n1292 = local read "Elevator Automate"() -> (w2891:T2)
              n1293 = Unbundle By Name(w2891) -> ("Forced Stop"=w2890:bool)
              n1294 = Greater Or Equal?(x=w2893, y=6000) -> (x >= y?=w2894:bool)
              n1295 = local read "STOP"() -> (w2895:bool)
              n1296 = Compound Arithmetic op=OR(w2890, w2894, w2895) -> (w2889:bool)
            }
            frame #2 {
            }
          }
          n1297 = local write "Delay Timer"(w2883) -> ()
          n1298 = Wait (ms)(milliseconds to wait=u32 1) -> ()  [unwired: 1 out]
        }
        n1299 = flat-sequence {
          tunnel: w2873 -> [w2874]
          tunnel: [w2874] -> w2871
          tunnel: w2871 -> [w2875]
          frame #0 {
          }
          frame #1 {
            n1300 = Not(x=w2875) -> (.not. x?=w2876:bool)
            n1301 = local read "Elevator Automate"() -> (w2877:T2)
            n1302 = Bundle By Name(cluster=w2877, "Forced Stop"=w2876) -> (w2878:T2)
            n1303 = local write "Elevator Automate"(w2878) -> ()
          }
          frame #2 {
          }
        }
      }
      frame "Cancel Delay" {
        n1304 = local read "Elevator Automate"() -> (w2918:T2)
        n1305 = Unbundle By Name(w2918) -> ("Elevator Command"=w2916:T1)
        n1306 = while {
          tunnel: [w3003] -> w2907
          tunnel: w2910 -> [w3011]
          tunnel: [w3001] -> w2906
          tunnel: [w3000] -> w2903
          i -> [w3002]
          stop <- w3003 stop-if-true
          w3005 = T8 12 items=["Floor Length"=48, "Sum of Floors"=12, "Floor Step in ms"=63, "Elevator Door Step in ms"=30, "Global Wait in ms"=20, "Event Wait in ms"=100] ("Elevator Constants")
          n1307 = Wait (ms)(milliseconds to wait=u32 1) -> ()  [unwired: 1 out]
          n1308 = To Long Integer(number=w3005) -> (32bit integer=w3004:i32)
          n1309 = local read "Elevator Cabin"() -> (w2997:T5)
          n1310 = local read "Elevator Automate"() -> (w3008:T2)
          n1311 = for {
            N: w3004 -> [_]
            shift-right: [w3018] -> w3000
            shift-left: FALSE -> [w3017]
            i -> [w3019]
            n1312 = Increment(x=w3019) -> (x+1=w3020:i32)
            n1313 = case shown="12" w3020 {
              tunnel: [w3022 w3026 w3030 w3034 w3038 w3042 w3046 w3050 w3054 w3058 w3062 w3066] -> w3018
              tunnel: w3017 -> [w3021 w3025 w3029 w3033 w3037 w3041 w3045 w3049 w3053 w3057 w3061 w3065]
              frame 1, Default {
                n1314 = local read "Elevator Panel"() -> (w3024:T3)
                n1315 = Unbundle By Name(w3024) -> ("Floor 1"=w3023:bool)
                n1316 = Or(x=w3023, y=w3021) -> (x .or. y?=w3022:bool)
              }
              frame 2 {
                n1317 = local read "Elevator Panel"() -> (w3028:T3)
                n1318 = Unbundle By Name(w3028) -> ("Floor 2"=w3027:bool)
                n1319 = Or(x=w3027, y=w3025) -> (x .or. y?=w3026:bool)
              }
              frame 3 {
                n1320 = local read "Elevator Panel"() -> (w3032:T3)
                n1321 = Unbundle By Name(w3032) -> ("Floor 3"=w3031:bool)
                n1322 = Or(x=w3031, y=w3029) -> (x .or. y?=w3030:bool)
              }
              frame 4 {
                n1323 = local read "Elevator Panel"() -> (w3036:T3)
                n1324 = Unbundle By Name(w3036) -> ("Floor 4"=w3035:bool)
                n1325 = Or(x=w3035, y=w3033) -> (x .or. y?=w3034:bool)
              }
              frame 5 {
                n1326 = local read "Elevator Panel"() -> (w3040:T3)
                n1327 = Unbundle By Name(w3040) -> ("Floor 5"=w3039:bool)
                n1328 = Or(x=w3039, y=w3037) -> (x .or. y?=w3038:bool)
              }
              frame 6 {
                n1329 = local read "Elevator Panel"() -> (w3044:T3)
                n1330 = Unbundle By Name(w3044) -> ("Floor 6"=w3043:bool)
                n1331 = Or(x=w3043, y=w3041) -> (x .or. y?=w3042:bool)
              }
              frame 7 {
                n1332 = local read "Elevator Panel"() -> (w3048:T3)
                n1333 = Unbundle By Name(w3048) -> ("Floor 7"=w3047:bool)
                n1334 = Or(x=w3047, y=w3045) -> (x .or. y?=w3046:bool)
              }
              frame 8 {
                n1335 = local read "Elevator Panel"() -> (w3052:T3)
                n1336 = Unbundle By Name(w3052) -> ("Floor 8"=w3051:bool)
                n1337 = Or(x=w3051, y=w3049) -> (x .or. y?=w3050:bool)
              }
              frame 9 {
                n1338 = local read "Elevator Panel"() -> (w3056:T3)
                n1339 = Unbundle By Name(w3056) -> ("Floor 9"=w3055:bool)
                n1340 = Or(x=w3055, y=w3053) -> (x .or. y?=w3054:bool)
              }
              frame 10 {
                n1341 = local read "Elevator Panel"() -> (w3060:T3)
                n1342 = Unbundle By Name(w3060) -> ("Floor 10"=w3059:bool)
                n1343 = Or(x=w3059, y=w3057) -> (x .or. y?=w3058:bool)
              }
              frame 11 {
                n1344 = local read "Elevator Panel"() -> (w3064:T3)
                n1345 = Unbundle By Name(w3064) -> ("Floor 11"=w3063:bool)
                n1346 = Or(x=w3063, y=w3061) -> (x .or. y?=w3062:bool)
              }
              frame 12 {
                n1347 = local read "Elevator Panel"() -> (w3068:T3)
                n1348 = Unbundle By Name(w3068) -> ("Floor 12"=w3067:bool)
                n1349 = Or(x=w3067, y=w3065) -> (x .or. y?=w3066:bool)
              }
            }
          }
          n1350 = case shown="True" w3011 {
            tunnel: [6000 ("y") 15000 ("y")] -> w3013
            frame False {
            }
            frame True {
            }
          }
          n1351 = Not Equal?(x=w2997, y=T5 100) -> (x != y?=w2996:bool)
          n1352 = Unbundle By Name(w3008) -> ("Forced Stop"=w3012:bool)
          n1353 = local write "Delay Timer"(w3002) -> ()
          n1354 = Greater Or Equal?(x=w3002, y=w3013) -> (x >= y?=w3014:bool)
          n1355 = local read "STOP"() -> (w3016:bool)
          n1356 = Select(t=T6."Stop", s=w2996, f=T6."Stand By" ("Elevator Status")) -> (s? t:f=w2993:T6)
          n1357 = Not(x=w3000) -> (.not. x?=w3006:bool)
          n1358 = Compound Arithmetic op=OR(w3012, w3014, w3016, w3000) -> (w3003:bool)
          n1359 = Select(t=w2993, s=w3003, f=T6."Cancel") -> (s? t:f=w3009:T6)
          n1360 = Bundle By Name(cluster=w3008, "Elevator Status"=w3009) -> (w2999:T2)
          n1361 = local write "Elevator Automate"(w2999) -> ()
          n1362 = And(x=w3003, y=w3006) -> (x .and. y?=w3001:bool)
        }
        n1363 = Equal?(x=w2916, y=Elevator_Command."Short Delay") -> (x = y?=w2912:bool)
        n1364 = Equal?(x=w2916, y=Elevator_Command."Going Up" ("element")) -> (x = y?=w2913:bool)
        n1365 = Equal?(x=w2916, y=Elevator_Command."Going Down") -> (x = y?=w2914:bool)
        n1366 = Compound Arithmetic op=OR(w2913, w2914, w2912) -> (w2911:bool)
        n1367 = flat-sequence {
          tunnel: w2918 -> [w2991]
          tunnel: w2917 -> [w2990]
          tunnel: w2911 -> [w2989]
          tunnel: [w2989] -> w2910
          frame #0 {
            n1368 = Bundle By Name(cluster=w2991, "Elevator Command"=w2990) -> (w2992:T2)
            n1369 = local write "Elevator Automate"(w2992) -> ()
          }
        }
        n1370 = local read "Elevator Cabin"() -> (w2901:T5)
        n1371 = Not Equal?(x=w2901, y=T5 100) -> (x != y?=w2902:bool)
        n1372 = And(x=w2902, y=w2903) -> (x .and. y?=w2904:bool)
        n1373 = Not(x=w2907) -> (.not. x?=w2919:bool)
        n1374 = case shown="True" w2906 {
          tunnel: [w2930 w2931] -> w2899
          frame False {
            n1375 = local read "Elevator Automate"() -> (w2930:T2)
          }
          frame True {
            w2933 = T8 12 items=["Floor Length"=48, "Sum of Floors"=12, "Floor Step in ms"=63, "Elevator Door Step in ms"=30, "Global Wait in ms"=20, "Event Wait in ms"=100] ("Elevator Constants")
            n1376 = To Long Integer(number=w2933) -> (32bit integer=w2932:i32)
            n1377 = for {
              N: w2932 -> [_]
              shift-right: [w2938] -> w2934
              shift-left: FALSE -> [w2937]
              i -> [w2939]
              n1378 = Increment(x=w2939) -> (x+1=w2940:i32)
              n1379 = case shown="1, Default" w2940 {
                tunnel: [w2942 w2946 w2950 w2954 w2958 w2962 w2966 w2970 w2974 w2978 w2982 w2986] -> w2938
                tunnel: w2937 -> [w2941 w2945 w2949 w2953 w2957 w2961 w2965 w2969 w2973 w2977 w2981 w2985]
                frame 1, Default {
                  n1380 = local read "Floors Schematic"() -> (w2944:T4)
                  n1381 = Unbundle By Name(w2944) -> ("Call 1"=w2943:bool)
                  n1382 = Or(x=w2943, y=w2941) -> (x .or. y?=w2942:bool)
                }
                frame 2 {
                  n1383 = local read "Floors Schematic"() -> (w2948:T4)
                  n1384 = Unbundle By Name(w2948) -> ("Call 2"=w2947:bool)
                  n1385 = Or(x=w2947, y=w2945) -> (x .or. y?=w2946:bool)
                }
                frame 3 {
                  n1386 = local read "Floors Schematic"() -> (w2952:T4)
                  n1387 = Unbundle By Name(w2952) -> ("Call 3"=w2951:bool)
                  n1388 = Or(x=w2951, y=w2949) -> (x .or. y?=w2950:bool)
                }
                frame 4 {
                  n1389 = local read "Floors Schematic"() -> (w2956:T4)
                  n1390 = Unbundle By Name(w2956) -> ("Call 4"=w2955:bool)
                  n1391 = Or(x=w2955, y=w2953) -> (x .or. y?=w2954:bool)
                }
                frame 5 {
                  n1392 = local read "Floors Schematic"() -> (w2960:T4)
                  n1393 = Unbundle By Name(w2960) -> ("Call 5"=w2959:bool)
                  n1394 = Or(x=w2959, y=w2957) -> (x .or. y?=w2958:bool)
                }
                frame 6 {
                  n1395 = local read "Floors Schematic"() -> (w2964:T4)
                  n1396 = Unbundle By Name(w2964) -> ("Call 6"=w2963:bool)
                  n1397 = Or(x=w2963, y=w2961) -> (x .or. y?=w2962:bool)
                }
                frame 7 {
                  n1398 = local read "Floors Schematic"() -> (w2968:T4)
                  n1399 = Unbundle By Name(w2968) -> ("Call 7"=w2967:bool)
                  n1400 = Or(x=w2967, y=w2965) -> (x .or. y?=w2966:bool)
                }
                frame 8 {
                  n1401 = local read "Floors Schematic"() -> (w2972:T4)
                  n1402 = Unbundle By Name(w2972) -> ("Call 8"=w2971:bool)
                  n1403 = Or(x=w2971, y=w2969) -> (x .or. y?=w2970:bool)
                }
                frame 9 {
                  n1404 = local read "Floors Schematic"() -> (w2976:T4)
                  n1405 = Unbundle By Name(w2976) -> ("Call 9"=w2975:bool)
                  n1406 = Or(x=w2975, y=w2973) -> (x .or. y?=w2974:bool)
                }
                frame 10 {
                  n1407 = local read "Floors Schematic"() -> (w2980:T4)
                  n1408 = Unbundle By Name(w2980) -> ("Call 10"=w2979:bool)
                  n1409 = Or(x=w2979, y=w2977) -> (x .or. y?=w2978:bool)
                }
                frame 11 {
                  n1410 = local read "Floors Schematic"() -> (w2984:T4)
                  n1411 = Unbundle By Name(w2984) -> ("Call 11"=w2983:bool)
                  n1412 = Or(x=w2983, y=w2981) -> (x .or. y?=w2982:bool)
                }
                frame 12 {
                  n1413 = local read "Floors Schematic"() -> (w2988:T4)
                  n1414 = Unbundle By Name(w2988) -> ("Call 12"=w2987:bool)
                  n1415 = Or(x=w2987, y=w2985) -> (x .or. y?=w2986:bool)
                }
              }
            }
            n1416 = local read "Elevator Automate"() -> (w2935:T2)
            n1417 = Bundle By Name(cluster=w2935, "Add Floor\nto Queue"=w2934) -> (w2931:T2)
          }
        }
        n1418 = case shown="True" w2904 {
          tunnel: w2909 -> [w2924 w2927]
          tunnel: w2908 -> [w2923 w2928]
          tunnel: [w2924 w2926] -> w2897
          tunnel: [w2923 w2925] -> w2905
          frame False {
          }
          frame True {
            n1419 = Enqueue Element At Opposite End(queue=w2927, element=Elevator_Command."Long Delay", error in (no error)=w2928) -> (queue out=w2926:refnum<queue>, error out=w2925:errorcluster)  [unwired: 1 in, 1 out]
          }
        }
        n1420 = Bundle By Name(cluster=w2899, "Cancel Delay"=w2919, "Forced Stop"=w2919) -> (w2898:T2)
        n1421 = local write "Elevator Automate"(w2898) -> ()
        n1422 = flat-sequence {
          tunnel: w2898 -> [_]
          tunnel: w2897 -> [_]
          frame #0 {
            n1423 = local read "Global Wait in ms"() -> (w2922:u32)
            n1424 = Wait (ms)(milliseconds to wait=w2922) -> ()  [unwired: 1 out]
          }
        }
      }
      frame "Open Doors" {
        # "Открыть двери лифта"
        n1425 = flat-sequence {
          tunnel: w3078 -> [w3084]
          tunnel: [w3084] -> w3074
          tunnel: [w3085] -> w3075
          tunnel: w3074 -> [w3086]
          tunnel: [w3088] -> w3077
          tunnel: w3075 -> [w3088]
          frame #0 {
          }
          frame #1 {
            n1426 = local read "Elevator Automate"() -> (w3087:T2)
            n1427 = Bundle By Name(cluster=w3087, "Elevator Command"=w3086) -> (w3085:T2)
            n1428 = local write "Elevator Automate"(w3085) -> ()
          }
          frame #2 {
          }
        }
        n1429 = while {
          tunnel: w3077 -> [_]
          tunnel: [w3092] -> w3076
          stop <- w3092 stop-if-true
          w3089 = T8 30 items=["Floor Length"=48, "Sum of Floors"=12, "Floor Step in ms"=63, "Elevator Door Step in ms"=30, "Global Wait in ms"=20, "Event Wait in ms"=100] ("Elevator Constants")
          n1430 = flat-sequence {
            tunnel: [w3097] -> w3091
            tunnel: [w3102] -> w3092
            tunnel: w3091 -> [w3102]
            frame #0 {
            }
            frame #1 {
              n1431 = local read "Elevator Cabin"() -> (w3094:T5)
              n1432 = local read "Elevator Automate"() -> (w3098:T2)
              n1433 = Unbundle By Name(w3098) -> ("Forced Stop"=w3099:bool)
              n1434 = Decrement(x=w3094) -> (x-1=w3095:T5)
              n1435 = Equal?(x=w3094, y=T5 0) -> (x = y?=w3096:bool)
              n1436 = local read "STOP"() -> (w3100:bool)
              n1437 = Select(t=w3094, s=w3096, f=w3095) -> (s? t:f=w3093:T5)
              n1438 = local write "Elevator Cabin"(w3093) -> ()
              n1439 = Compound Arithmetic op=OR(w3099, w3096, w3100) -> (w3097:bool)
            }
            frame #2 {
            }
          }
          n1440 = To Unsigned Long Integer(number=w3089) -> (unsigned 32bit integer=w3090:u32)
          n1441 = Wait (ms)(milliseconds to wait=w3090) -> ()  [unwired: 1 out]
        }
        n1442 = flat-sequence {
          tunnel: w3076 -> [w3079]
          tunnel: [w3079] -> w3073
          tunnel: w3073 -> [w3080]
          frame #0 {
          }
          frame #1 {
            n1443 = Not(x=w3080) -> (.not. x?=w3081:bool)
            n1444 = local read "Elevator Automate"() -> (w3082:T2)
            n1445 = Bundle By Name(cluster=w3082, "Forced Stop"=w3081) -> (w3083:T2)
            n1446 = local write "Elevator Automate"(w3083) -> ()
          }
          frame #2 {
          }
        }
      }
      frame "Close Doors" {
        # "Закрыть двери лифта"
        n1447 = flat-sequence {
          tunnel: w3110 -> [w3116]
          tunnel: [w3116] -> w3106
          tunnel: [w3117] -> w3107
          tunnel: w3106 -> [w3118]
          tunnel: [w3120] -> w3109
          tunnel: w3107 -> [w3120]
          frame #0 {
          }
          frame #1 {
            n1448 = local read "Elevator Automate"() -> (w3119:T2)
            n1449 = Bundle By Name(cluster=w3119, "Elevator Command"=w3118) -> (w3117:T2)
            n1450 = local write "Elevator Automate"(w3117) -> ()
          }
          frame #2 {
          }
        }
        n1451 = while {
          tunnel: w3109 -> [_]
          tunnel: [w3124] -> w3108
          stop <- w3124 stop-if-true
          w3121 = T8 30 items=["Floor Length"=48, "Sum of Floors"=12, "Floor Step in ms"=63, "Elevator Door Step in ms"=30, "Global Wait in ms"=20, "Event Wait in ms"=100] ("Elevator Constants")
          n1452 = flat-sequence {
            tunnel: [w3129] -> w3123
            tunnel: [w3134] -> w3124
            tunnel: w3123 -> [w3134]
            frame #0 {
            }
            frame #1 {
              n1453 = local read "Elevator Cabin"() -> (w3126:T5)
              n1454 = local read "Elevator Automate"() -> (w3130:T2)
              n1455 = Unbundle By Name(w3130) -> ("Forced Stop"=w3131:bool)
              n1456 = Increment(x=w3126) -> (x+1=w3127:T5)
              n1457 = Equal?(x=w3126, y=T5 100) -> (x = y?=w3128:bool)
              n1458 = local read "STOP"() -> (w3132:bool)
              n1459 = Select(t=w3126, s=w3128, f=w3127) -> (s? t:f=w3125:T5)
              n1460 = local write "Elevator Cabin"(w3125) -> ()
              n1461 = Compound Arithmetic op=OR(w3131, w3128, w3132) -> (w3129:bool)
            }
            frame #2 {
            }
          }
          n1462 = To Unsigned Long Integer(number=w3121) -> (unsigned 32bit integer=w3122:u32)
          n1463 = Wait (ms)(milliseconds to wait=w3122) -> ()  [unwired: 1 out]
        }
        n1464 = flat-sequence {
          tunnel: w3108 -> [w3111]
          tunnel: [w3111] -> w3105
          tunnel: w3105 -> [w3112]
          frame #0 {
          }
          frame #1 {
            n1465 = Not(x=w3112) -> (.not. x?=w3113:bool)
            n1466 = local read "Elevator Automate"() -> (w3114:T2)
            n1467 = Bundle By Name(cluster=w3114, "Forced Stop"=w3113) -> (w3115:T2)
            n1468 = local write "Elevator Automate"(w3115) -> ()
          }
          frame #2 {
          }
        }
      }
      frame "Going Down" {
        # "Отправить кабину лифта вниз"
        n1469 = local read "Elevator Automate"() -> (w3146:T2)
        n1470 = Bundle By Name(cluster=w3146, "Elevator Command"=w3145, "Elevator Status"=T6."Going Down") -> (w3144:T2)
        n1471 = control-ref of="Elevator Cabin"() -> (w3149:refnum<vi>)
        n1472 = property class="Slide (strict)"(reference=w3149) -> (reference out=w3147:refnum<vi>, "Top"=w3148:i32)  [unwired: 1 in, 1 out]
        n1473 = while {
          tunnel: w3147 -> [w3158]
          shift-right: [w3157] -> _
          shift-left: w3148 -> [w3159]
          tunnel: w3144 -> [_]
          tunnel: [w3155] -> w3140
          tunnel: [w3154] -> w3137
          stop <- w3156 stop-if-true
          n1474 = flat-sequence {
            tunnel: w3159 -> [w3163]
            tunnel: w3158 -> [w3164]
            tunnel: [w3164] -> w3162
            tunnel: [w3163] -> w3161
            tunnel: [w3180] -> w3160
            tunnel: w3162 -> [w3181]
            tunnel: w3161 -> [w3167]
            tunnel: [w3166] -> w3156
            tunnel: [w3166] -> w3155
            tunnel: [w3165] -> w3154
            tunnel: [w3183] -> w3157
            tunnel: w3160 -> [w3183]
            frame #0 {
            }
            frame #1 {
              w3168 = T8 40 items=["Floor Length"=48, "Sum of Floors"=12, "Floor Step in ms"=40, "Elevator Door Step in ms"=30, "Global Wait in ms"=20, "Event Wait in ms"=100] ("Elevator Constants")
              n1475 = local read "Floors Schematic"() -> (w3176:T4)
              n1476 = local read "Elevator Automate"() -> (w3165:T2)
              n1477 = local read "Elevator Automate"() -> (w3173:T2)
              n1478 = Unbundle By Name(w3176) -> ("Floor Position"=w3175:i16[])
              n1479 = Unbundle By Name(w3173) -> ("Target Floor"=w3172:u8)
              n1480 = property class="Slide (strict)"(reference=w3181, "Top"=w3167) -> ()  [unwired: 1 in, 2 out]
              n1481 = Unbundle By Name(w3165) -> ("Forced Stop"=w3169:bool)
              n1482 = Decrement(x=w3172) -> (x-1=w3170:u8)
              n1483 = To Unsigned Long Integer(number=w3168) -> (unsigned 32bit integer=w3179:u32)
              n1484 = To Long Integer(number=w3170) -> (32bit integer=w3171:i32)
              n1485 = Wait (ms)(milliseconds to wait=w3179) -> ()  [unwired: 1 out]
              n1486 = Index Array(array=w3175, index=w3171) -> (element=w3174:i16)
              n1487 = To Long Integer(number=w3174) -> (32bit integer=w3182:i32)
              n1488 = Increment(x=w3167) -> (x+1=w3180:i32)
              n1489 = Equal?(x=w3167, y=w3182) -> (x = y?=w3178:bool)
              n1490 = local read "STOP"() -> (w3177:bool)
              n1491 = Compound Arithmetic op=OR(w3169, w3178, w3177) -> (w3166:bool)
            }
            frame #2 {
            }
          }
        }
        n1492 = local write "Elevator Automate"(w3144) -> ()
        n1493 = Unbundle By Name(w3137) -> ("Cancel Delay"=w3141:bool)
        n1494 = case shown="False" w3141 {
          tunnel: [w3151 w3153] -> w3139
          tunnel: w3137 -> [w3150 w3153]
          frame False {
            n1495 = Bundle By Name(cluster=w3150, "Elevator Status"=T6."Stop") -> (w3151:T2)
          }
          frame True {
          }
        }
        n1496 = Not(x=w3140) -> (.not. x?=w3143:bool)
        n1497 = Bundle By Name(cluster=w3139, "Forced Stop"=w3143) -> (w3142:T2)
        n1498 = local write "Elevator Automate"(w3142) -> ()
      }
      frame "Going Up" {
        # "Отправить кабину лифта наверх"
        n1499 = local read "Elevator Automate"() -> (w3195:T2)
        n1500 = Bundle By Name(cluster=w3195, "Elevator Command"=w3194, "Elevator Status"=T6."Going Up") -> (w3193:T2)
        n1501 = control-ref of="Elevator Cabin"() -> (w3198:refnum<vi>)
        n1502 = property class="Slide (strict)"(reference=w3198) -> (reference out=w3196:refnum<vi>, "Top"=w3197:i32)  [unwired: 1 in, 1 out]
        n1503 = while {
          tunnel: w3196 -> [w3207]
          shift-right: [w3205] -> _
          shift-left: w3197 -> [w3208]
          tunnel: w3193 -> [_]
          tunnel: [w3204] -> w3187
          tunnel: [w3203] -> w3186
          stop <- w3206 stop-if-true
          n1504 = flat-sequence {
            tunnel: w3208 -> [w3212]
            tunnel: w3207 -> [w3213]
            tunnel: [w3213] -> w3211
            tunnel: [w3212] -> w3210
            tunnel: w3211 -> [w3229]
            tunnel: w3210 -> [w3216]
            tunnel: [w3228] -> w3209
            tunnel: [w3215] -> w3206
            tunnel: [w3215] -> w3204
            tunnel: [w3214] -> w3203
            tunnel: [w3231] -> w3205
            tunnel: w3209 -> [w3231]
            frame #0 {
            }
            frame #1 {
              w3217 = T8 40 items=["Floor Length"=48, "Sum of Floors"=12, "Floor Step in ms"=40, "Elevator Door Step in ms"=30, "Global Wait in ms"=20, "Event Wait in ms"=100] ("Elevator Constants")
              n1505 = local read "Floors Schematic"() -> (w3225:T4)
              n1506 = local read "Elevator Automate"() -> (w3214:T2)
              n1507 = Unbundle By Name(w3225) -> ("Floor Position"=w3224:i16[])
              n1508 = Unbundle By Name(w3214) -> ("Target Floor"=w3222:u8)
              n1509 = property class="Slide (strict)"(reference=w3229, "Top"=w3216) -> ()  [unwired: 1 in, 2 out]
              n1510 = Decrement(x=w3222) -> (x-1=w3220:u8)
              n1511 = To Long Integer(number=w3220) -> (32bit integer=w3221:i32)
              n1512 = To Unsigned Long Integer(number=w3217) -> (unsigned 32bit integer=w3219:u32)
              n1513 = Unbundle By Name(w3214) -> ("Forced Stop"=w3218:bool)
              n1514 = Index Array(array=w3224, index=w3221) -> (element=w3223:i16)
              n1515 = Wait (ms)(milliseconds to wait=w3219) -> ()  [unwired: 1 out]
              n1516 = To Long Integer(number=w3223) -> (32bit integer=w3230:i32)
              n1517 = Decrement(x=w3216) -> (x-1=w3228:i32)
              n1518 = Equal?(x=w3216, y=w3230) -> (x = y?=w3227:bool)
              n1519 = local read "STOP"() -> (w3226:bool)
              n1520 = Compound Arithmetic op=OR(w3218, w3227, w3226) -> (w3215:bool)
            }
            frame #2 {
            }
          }
        }
        n1521 = local write "Elevator Automate"(w3193) -> ()
        n1522 = Unbundle By Name(w3186) -> ("Cancel Delay"=w3190:bool)
        n1523 = case shown="False" w3190 {
          tunnel: [w3200 w3202] -> w3189
          tunnel: w3186 -> [w3199 w3202]
          frame False {
            n1524 = Bundle By Name(cluster=w3199, "Elevator Status"=T6."Stop") -> (w3200:T2)
          }
          frame True {
          }
        }
        n1525 = Not(x=w3187) -> (.not. x?=w3192:bool)
        n1526 = Bundle By Name(cluster=w3189, "Forced Stop"=w3192) -> (w3191:T2)
        n1527 = local write "Elevator Automate"(w3191) -> ()
      }
      frame "Unpress Button" {
        n1528 = flat-sequence {
          tunnel: w3234 -> [w3247]
          frame #0 {
            # "Отжать кнопку на этаже дома и кнопку в кабине"
            n1529 = local read "Elevator Automate"() -> (w3235:T2)
            n1530 = Unbundle By Name(w3235) -> ("Target Floor"=w3239:u8)
            n1531 = Unbundle By Name(w3235) -> ("Elevator Panel Array"=w3242:bool[])
            n1532 = Decrement(x=w3239) -> (x-1=w3248:u8)
            n1533 = To Long Integer(number=w3248) -> (32bit integer=w3240:i32)
            n1534 = Replace Array Subset(array=w3242, new element=FALSE ("new element/subarray"), index=w3240) -> (w3243:bool[])
            n1535 = Bundle By Name(cluster=w3235, "Elevator Panel Array"=w3243) -> (w3238:T2)
            n1536 = Unbundle By Name(w3238) -> ("Floor Array"=w3246:bool[])
            n1537 = Replace Array Subset(array=w3246, new element=FALSE ("new element/subarray"), index=w3240) -> (w3244:bool[])
            n1538 = Bundle By Name(cluster=w3238, "Floor Array"=w3244) -> (w3237:T2)
            n1539 = Bundle By Name(cluster=w3237, "Elevator Command"=w3247) -> (w3236:T2)
            n1540 = local write "Elevator Automate"(w3236) -> ()
            n1541 = case shown="11" w3239 {
              tunnel: w3236 -> [_ _ _ _ _ _ _ _ _ _ _ _]
              frame 1, Default {
                n1542 = local read "Floors Schematic"() -> (w3322:T4)
                n1543 = Bundle By Name(cluster=w3322, "Call 1"=FALSE ("Call 12")) -> (w3320:T4)
                n1544 = control-ref of="Call 1"() -> (w3324:refnum<vi>)
                n1545 = local write "Floors Schematic"(w3320) -> ()
                n1546 = property class="Bool (strict)"(reference=w3324, "DisabledEnum"=T7."Enabled" ("Disabled")) -> ()  [unwired: 1 in, 2 out]
              }
              frame 2 {
                n1547 = local read "Floors Schematic"() -> (w3327:T4)
                n1548 = Bundle By Name(cluster=w3327, "Call 2"=FALSE ("Call 12")) -> (w3325:T4)
                n1549 = control-ref of="Call 2"() -> (w3329:refnum<vi>)
                n1550 = local write "Floors Schematic"(w3325) -> ()
                n1551 = property class="Bool (strict)"(reference=w3329, "DisabledEnum"=T7."Enabled" ("Disabled")) -> ()  [unwired: 1 in, 2 out]
              }
              frame 3 {
                n1552 = local read "Floors Schematic"() -> (w3332:T4)
                n1553 = Bundle By Name(cluster=w3332, "Call 3"=FALSE ("Call 12")) -> (w3330:T4)
                n1554 = control-ref of="Call 3"() -> (w3334:refnum<vi>)
                n1555 = local write "Floors Schematic"(w3330) -> ()
                n1556 = property class="Bool (strict)"(reference=w3334, "DisabledEnum"=T7."Enabled" ("Disabled")) -> ()  [unwired: 1 in, 2 out]
              }
              frame 4 {
                n1557 = local read "Floors Schematic"() -> (w3337:T4)
                n1558 = Bundle By Name(cluster=w3337, "Call 4"=FALSE ("Call 12")) -> (w3335:T4)
                n1559 = control-ref of="Call 4"() -> (w3339:refnum<vi>)
                n1560 = local write "Floors Schematic"(w3335) -> ()
                n1561 = property class="Bool (strict)"(reference=w3339, "DisabledEnum"=T7."Enabled" ("Disabled")) -> ()  [unwired: 1 in, 2 out]
              }
              frame 5 {
                n1562 = local read "Floors Schematic"() -> (w3342:T4)
                n1563 = Bundle By Name(cluster=w3342, "Call 5"=FALSE ("Call 12")) -> (w3340:T4)
                n1564 = control-ref of="Call 5"() -> (w3344:refnum<vi>)
                n1565 = local write "Floors Schematic"(w3340) -> ()
                n1566 = property class="Bool (strict)"(reference=w3344, "DisabledEnum"=T7."Enabled" ("Disabled")) -> ()  [unwired: 1 in, 2 out]
              }
              frame 6 {
                n1567 = local read "Floors Schematic"() -> (w3347:T4)
                n1568 = Bundle By Name(cluster=w3347, "Call 6"=FALSE ("Call 12")) -> (w3345:T4)
                n1569 = control-ref of="Call 6"() -> (w3349:refnum<vi>)
                n1570 = local write "Floors Schematic"(w3345) -> ()
                n1571 = property class="Bool (strict)"(reference=w3349, "DisabledEnum"=T7."Enabled" ("Disabled")) -> ()  [unwired: 1 in, 2 out]
              }
              frame 7 {
                n1572 = local read "Floors Schematic"() -> (w3352:T4)
                n1573 = Bundle By Name(cluster=w3352, "Call 7"=FALSE ("Call 12")) -> (w3350:T4)
                n1574 = control-ref of="Call 7"() -> (w3354:refnum<vi>)
                n1575 = local write "Floors Schematic"(w3350) -> ()
                n1576 = property class="Bool (strict)"(reference=w3354, "DisabledEnum"=T7."Enabled" ("Disabled")) -> ()  [unwired: 1 in, 2 out]
              }
              frame 8 {
                n1577 = local read "Floors Schematic"() -> (w3357:T4)
                n1578 = Bundle By Name(cluster=w3357, "Call 8"=FALSE ("Call 12")) -> (w3355:T4)
                n1579 = control-ref of="Call 8"() -> (w3359:refnum<vi>)
                n1580 = local write "Floors Schematic"(w3355) -> ()
                n1581 = property class="Bool (strict)"(reference=w3359, "DisabledEnum"=T7."Enabled" ("Disabled")) -> ()  [unwired: 1 in, 2 out]
              }
              frame 9 {
                n1582 = local read "Floors Schematic"() -> (w3362:T4)
                n1583 = Bundle By Name(cluster=w3362, "Call 9"=FALSE ("Call 12")) -> (w3360:T4)
                n1584 = control-ref of="Call 9"() -> (w3364:refnum<vi>)
                n1585 = local write "Floors Schematic"(w3360) -> ()
                n1586 = property class="Bool (strict)"(reference=w3364, "DisabledEnum"=T7."Enabled" ("Disabled")) -> ()  [unwired: 1 in, 2 out]
              }
              frame 10 {
                n1587 = local read "Floors Schematic"() -> (w3367:T4)
                n1588 = Bundle By Name(cluster=w3367, "Call 10"=FALSE ("Call 12")) -> (w3365:T4)
                n1589 = control-ref of="Call 10"() -> (w3369:refnum<vi>)
                n1590 = local write "Floors Schematic"(w3365) -> ()
                n1591 = property class="Bool (strict)"(reference=w3369, "DisabledEnum"=T7."Enabled" ("Disabled")) -> ()  [unwired: 1 in, 2 out]
              }
              frame 11 {
                n1592 = local read "Floors Schematic"() -> (w3372:T4)
                n1593 = Bundle By Name(cluster=w3372, "Call 11"=FALSE ("Call 12")) -> (w3370:T4)
                n1594 = control-ref of="Call 11"() -> (w3374:refnum<vi>)
                n1595 = local write "Floors Schematic"(w3370) -> ()
                n1596 = property class="Bool (strict)"(reference=w3374, "DisabledEnum"=T7."Enabled" ("Disabled")) -> ()  [unwired: 1 in, 2 out]
              }
              frame 12 {
                n1597 = local read "Floors Schematic"() -> (w3377:T4)
                n1598 = Bundle By Name(cluster=w3377, "Call 12"=FALSE) -> (w3375:T4)
                n1599 = control-ref of="Call 12"() -> (w3379:refnum<vi>)
                n1600 = local write "Floors Schematic"(w3375) -> ()
                n1601 = property class="Bool (strict)"(reference=w3379, "DisabledEnum"=T7."Enabled" ("Disabled")) -> ()  [unwired: 1 in, 2 out]
              }
            }
            n1602 = case shown="12" w3239 {
              tunnel: w3236 -> [_ _ _ _ _ _ _ _ _ _ _ _]
              frame 1, Default {
                n1603 = local read "Elevator Panel"() -> (w3252:T3)
                n1604 = Wait (ms)(milliseconds to wait=u32 1) -> ()  [unwired: 1 out]
                n1605 = Bundle By Name(cluster=w3252, "Floor 1"=FALSE ("Call 12")) -> (w3250:T3)
                n1606 = control-ref of="Floor 1"() -> (w3254:refnum<vi>)
                n1607 = local write "Elevator Panel"(w3250) -> ()
                n1608 = property class="Bool (strict)"(reference=w3254, "DisabledEnum"=T7."Enabled" ("Disabled")) -> ()  [unwired: 1 in, 2 out]
              }
              frame 2 {
                n1609 = local read "Elevator Panel"() -> (w3258:T3)
                n1610 = Wait (ms)(milliseconds to wait=u32 1) -> ()  [unwired: 1 out]
                n1611 = Bundle By Name(cluster=w3258, "Floor 2"=FALSE ("Call 12")) -> (w3256:T3)
                n1612 = control-ref of="Floor 2"() -> (w3260:refnum<vi>)
                n1613 = local write "Elevator Panel"(w3256) -> ()
                n1614 = property class="Bool (strict)"(reference=w3260, "DisabledEnum"=T7."Enabled" ("Disabled")) -> ()  [unwired: 1 in, 2 out]
              }
              frame 3 {
                n1615 = local read "Elevator Panel"() -> (w3264:T3)
                n1616 = Wait (ms)(milliseconds to wait=u32 1) -> ()  [unwired: 1 out]
                n1617 = Bundle By Name(cluster=w3264, "Floor 3"=FALSE ("Call 12")) -> (w3262:T3)
                n1618 = control-ref of="Floor 3"() -> (w3266:refnum<vi>)
                n1619 = local write "Elevator Panel"(w3262) -> ()
                n1620 = property class="Bool (strict)"(reference=w3266, "DisabledEnum"=T7."Enabled" ("Disabled")) -> ()  [unwired: 1 in, 2 out]
              }
              frame 4 {
                n1621 = Wait (ms)(milliseconds to wait=u32 1) -> ()  [unwired: 1 out]
                n1622 = local read "Elevator Panel"() -> (w3270:T3)
                n1623 = Bundle By Name(cluster=w3270, "Floor 4"=FALSE ("Call 12")) -> (w3268:T3)
                n1624 = control-ref of="Floor 4"() -> (w3272:refnum<vi>)
                n1625 = local write "Elevator Panel"(w3268) -> ()
                n1626 = property class="Bool (strict)"(reference=w3272, "DisabledEnum"=T7."Enabled" ("Disabled")) -> ()  [unwired: 1 in, 2 out]
              }
              frame 5 {
                n1627 = Wait (ms)(milliseconds to wait=u32 1) -> ()  [unwired: 1 out]
                n1628 = local read "Elevator Panel"() -> (w3276:T3)
                n1629 = Bundle By Name(cluster=w3276, "Floor 5"=FALSE ("Call 12")) -> (w3274:T3)
                n1630 = control-ref of="Floor 5"() -> (w3278:refnum<vi>)
                n1631 = local write "Elevator Panel"(w3274) -> ()
                n1632 = property class="Bool (strict)"(reference=w3278, "DisabledEnum"=T7."Enabled" ("Disabled")) -> ()  [unwired: 1 in, 2 out]
              }
              frame 6 {
                n1633 = local read "Elevator Panel"() -> (w3282:T3)
                n1634 = Wait (ms)(milliseconds to wait=u32 1) -> ()  [unwired: 1 out]
                n1635 = Bundle By Name(cluster=w3282, "Floor 6"=FALSE ("Call 12")) -> (w3280:T3)
                n1636 = control-ref of="Floor 6"() -> (w3284:refnum<vi>)
                n1637 = local write "Elevator Panel"(w3280) -> ()
                n1638 = property class="Bool (strict)"(reference=w3284, "DisabledEnum"=T7."Enabled" ("Disabled")) -> ()  [unwired: 1 in, 2 out]
              }
              frame 7 {
                n1639 = Wait (ms)(milliseconds to wait=u32 1) -> ()  [unwired: 1 out]
                n1640 = local read "Elevator Panel"() -> (w3288:T3)
                n1641 = Bundle By Name(cluster=w3288, "Floor 7"=FALSE ("Call 12")) -> (w3286:T3)
                n1642 = control-ref of="Floor 7"() -> (w3290:refnum<vi>)
                n1643 = local write "Elevator Panel"(w3286) -> ()
                n1644 = property class="Bool (strict)"(reference=w3290, "DisabledEnum"=T7."Enabled" ("Disabled")) -> ()  [unwired: 1 in, 2 out]
              }
              frame 8 {
                n1645 = Wait (ms)(milliseconds to wait=u32 1) -> ()  [unwired: 1 out]
                n1646 = local read "Elevator Panel"() -> (w3294:T3)
                n1647 = Bundle By Name(cluster=w3294, "Floor 8"=FALSE ("Call 12")) -> (w3292:T3)
                n1648 = control-ref of="Floor 8"() -> (w3296:refnum<vi>)
                n1649 = local write "Elevator Panel"(w3292) -> ()
                n1650 = property class="Bool (strict)"(reference=w3296, "DisabledEnum"=T7."Enabled" ("Disabled")) -> ()  [unwired: 1 in, 2 out]
              }
              frame 9 {
                n1651 = Wait (ms)(milliseconds to wait=u32 1) -> ()  [unwired: 1 out]
                n1652 = local read "Elevator Panel"() -> (w3300:T3)
                n1653 = Bundle By Name(cluster=w3300, "Floor 9"=FALSE ("Call 12")) -> (w3298:T3)
                n1654 = control-ref of="Floor 9"() -> (w3302:refnum<vi>)
                n1655 = local write "Elevator Panel"(w3298) -> ()
                n1656 = property class="Bool (strict)"(reference=w3302, "DisabledEnum"=T7."Enabled" ("Disabled")) -> ()  [unwired: 1 in, 2 out]
              }
              frame 10 {
                n1657 = Wait (ms)(milliseconds to wait=u32 1) -> ()  [unwired: 1 out]
                n1658 = local read "Elevator Panel"() -> (w3306:T3)
                n1659 = Bundle By Name(cluster=w3306, "Floor 10"=FALSE ("Call 12")) -> (w3304:T3)
                n1660 = control-ref of="Floor 10"() -> (w3308:refnum<vi>)
                n1661 = local write "Elevator Panel"(w3304) -> ()
                n1662 = property class="Bool (strict)"(reference=w3308, "DisabledEnum"=T7."Enabled" ("Disabled")) -> ()  [unwired: 1 in, 2 out]
              }
              frame 11 {
                n1663 = Wait (ms)(milliseconds to wait=u32 1) -> ()  [unwired: 1 out]
                n1664 = local read "Elevator Panel"() -> (w3312:T3)
                n1665 = Bundle By Name(cluster=w3312, "Floor 11"=FALSE ("Call 12")) -> (w3310:T3)
                n1666 = control-ref of="Floor 11"() -> (w3314:refnum<vi>)
                n1667 = local write "Elevator Panel"(w3310) -> ()
                n1668 = property class="Bool (strict)"(reference=w3314, "DisabledEnum"=T7."Enabled" ("Disabled")) -> ()  [unwired: 1 in, 2 out]
              }
              frame 12 {
                n1669 = local read "Elevator Panel"() -> (w3317:T3)
                n1670 = Bundle By Name(cluster=w3317, "Floor 12"=FALSE ("Call 12")) -> (w3316:T3)
                n1671 = control-ref of="Floor 12"() -> (w3319:refnum<vi>)
                n1672 = local write "Elevator Panel"(w3316) -> ()
                n1673 = property class="Bool (strict)"(reference=w3319, "DisabledEnum"=T7."Enabled" ("Disabled")) -> ()  [unwired: 1 in, 2 out]
              }
            }
          }
        }
      }
    }
    n1674 = Wait (ms)(milliseconds to wait=w2821) -> ()  [unwired: 1 out]
  }
  n1675 = while {
    shift-right: [w3382] -> _
    shift-left: w5 -> [w3384]
    shift-right: [w3381] -> _
    shift-left: w4 -> [w3385]
    tunnel: w2 -> [_]
    tunnel: w1 -> [_]
    stop <- w3383 stop-if-true
    # "Передача номера первого в очереди\nэтажа в номер этажа, на который нужно приехать в текущий момент времени"
    n1676 = local read "Global Wait in ms"() -> (w3380:u32)
    n1677 = flat-sequence {
      tunnel: w3385 -> [w3391]
      tunnel: w3384 -> [w3390]
      tunnel: [w3388] -> w3382
      tunnel: [w3387] -> w3381
      frame #0 {
        n1678 = local read "Elevator Automate"() -> (w3386:T2)
        n1679 = Unbundle By Name(w3386) -> ("Update\nTarget Floor"=w3389:bool)
        n1680 = case shown="False" w3389 {
          tunnel: w3391 -> [w3392 w3402]
          tunnel: w3390 -> [w3393 w3401]
          tunnel: [w3393 w3400] -> w3388
          tunnel: [w3392 w3399] -> w3387
          tunnel: w3386 -> [_ w3398]
          frame False {
          }
          frame True {
            n1681 = Dequeue Element(queue=w3401, error in (no error)=w3402) -> (queue out=w3400:refnum<queue>, element=w3395:u8, error out=w3399:errorcluster)  [unwired: 1 in, 1 out]
            n1682 = Bundle By Name(cluster=w3398, "Target Floor"=w3395, "Update\nTarget Floor"=FALSE ("Update Target Floor")) -> (w3397:T2)
            n1683 = local write "Elevator Automate"(w3397) -> ()
            n1684 = Wait (ms)(milliseconds to wait=u32 1) -> ()  [unwired: 1 out]
          }
        }
      }
    }
    n1685 = Wait (ms)(milliseconds to wait=w3380) -> ()  [unwired: 1 out]
    n1686 = local read "STOP"() -> (w3383:bool)
  }
  n1687 = while {
    shift-right: [w3410] -> _
    shift-left: w5 -> [w3405]
    shift-right: [w3409] -> _
    shift-left: w4 -> [w3404]
    tunnel: w2 -> [_]
    tunnel: w1 -> [_]
    stop <- w3411 stop-if-true
    # "Передача номера первого в очереди\nэтажа в номер этажа, на который нужно приехать\nв текущий момент времени"
    n1688 = flat-sequence {
      tunnel: [w3415] -> w3408
      tunnel: [w3414] -> w3407
      tunnel: [w3418] -> w3406
      tunnel: w3405 -> [w3417]
      tunnel: w3404 -> [w3416]
      tunnel: [w3426] -> w3410
      tunnel: [w3425] -> w3409
      tunnel: w3408 -> [w3429]
      tunnel: w3407 -> [w3428]
      tunnel: w3406 -> [w3427]
      frame #0 {
        n1689 = local read "# elements in Elevator Floor Queue"() -> (w3412:i32)
        n1690 = local read "Elevator Automate"() -> (w3422:T2)
        n1691 = Unbundle By Name(w3422) -> ("Elevator Command"=w3424:T1)
        n1692 = To Long Integer(number=1) -> (32bit integer=w3421:i32)
        n1693 = Preview Queue Element(queue=w3417, timeout in ms (-1)=w3421, error in (no error)=w3416) -> (queue out=w3415:refnum<queue>, error out=w3414:errorcluster)  [unwired: 2 out]
        n1694 = Equal?(x=w3424, y=Elevator_Command."Idle" ("element")) -> (x = y?=w3423:bool)
        n1695 = Not Equal To 0?(x=w3412) -> (x != 0?=w3413:bool)
        n1696 = And(x=w3423, y=w3413) -> (x .and. y?=w3418:bool)
      }
      frame #1 {
        n1697 = case shown="True" w3427 {
          tunnel: w3429 -> [w3431 w3433]
          tunnel: w3428 -> [w3430 w3432]
          tunnel: [w3431 w3433] -> w3426
          tunnel: [w3430 w3432] -> w3425
          frame False {
          }
          frame True {
            n1698 = flat-sequence {
              frame #0 {
                n1699 = local read "Elevator Automate"() -> (w3436:T2)
                n1700 = Bundle By Name(cluster=w3436, "Update\nTarget Floor"=TRUE ("Update Target Floor")) -> (w3435:T2)
                n1701 = local write "Elevator Automate"(w3435) -> ()
                n1702 = Wait (ms)(milliseconds to wait=u32 200) -> ()  [unwired: 1 out]
              }
              frame #1 {
                n1703 = local read "Elevator Automate"() -> (w3441:T2)
                n1704 = Bundle By Name(cluster=w3441, "Take a Call"=TRUE ("Update Target Floor")) -> (w3440:T2)
                n1705 = local write "Elevator Automate"(w3440) -> ()
                n1706 = Wait (ms)(milliseconds to wait=u32 200) -> ()  [unwired: 1 out]
              }
            }
          }
        }
      }
    }
    n1707 = local read "Global Wait in ms"() -> (w3403:u32)
    n1708 = Wait (ms)(milliseconds to wait=w3403) -> ()  [unwired: 1 out]
    n1709 = local read "STOP"() -> (w3411:bool)
  }
  n1710 = while {
    shift-right: [w3447] -> _
    shift-left: w6 -> [w3446]
    shift-right: [w3443] -> _
    shift-left: w7 -> [w3445]
    tunnel: w1 -> [_]
    tunnel: w2 -> [_]
    stop <- w3444 stop-if-true
    # "Принятие следующего в очереди вызова с добавлением команд управления лифтом в очередь"
    n1711 = local read "Global Wait in ms"() -> (w3442:u32)
    n1712 = flat-sequence {
      tunnel: [w3453] -> w3447
      tunnel: w3446 -> [w3452]
      tunnel: w3445 -> [w3451]
      tunnel: [w3448] -> w3443
      frame #0 {
        n1713 = local read "Elevator Automate"() -> (w3449:T2)
        n1714 = Unbundle By Name(w3449) -> ("Take a Call"=w3450:bool)
        n1715 = case shown="True" w3450 {
          tunnel: w3451 -> [w3454 w3495]
          tunnel: w3452 -> [w3455 w3494]
          tunnel: [w3455 w3496] -> w3453
          tunnel: [w3454 w3457] -> w3448
          frame False {
          }
          frame True {
            n1716 = local read "Elevator Automate"() -> (w3465:T2)
            n1717 = local read "Floors Schematic"() -> (w3479:T4)
            n1718 = Unbundle By Name(w3465) -> ("Elevator Status"=w3464:T6)
            n1719 = Equal?(x=w3464, y=T9."Stand By") -> (x = y?=w3460:bool)
            n1720 = Unbundle By Name(w3479) -> ("Floor Position"=w3480:i16[])
            n1721 = Unbundle By Name(w3465) -> ("Target Floor"=w3476:u8)
            n1722 = control-ref of="Elevator Cabin"() -> (w3474:refnum<vi>)
            n1723 = Decrement(x=w3476) -> (x-1=w3477:u8)
            n1724 = property class="Slide (strict)"(reference=w3474) -> ("Top"=w3462:i32)  [unwired: 1 in, 2 out]
            n1725 = To Long Integer(number=w3477) -> (32bit integer=w3478:i32)
            n1726 = Index Array(array=w3480, index=w3478) -> (element=w3475:i16)
            n1727 = To Long Integer(number=w3475) -> (32bit integer=w3461:i32)
            n1728 = Bundle By Name(cluster=w3465, "Take a Call"=FALSE ("Update Target Floor")) -> (w3484:T2)
            n1729 = Greater Or Equal?(x=w3462, y=w3461) -> (x >= y?=w3468:bool)
            n1730 = case shown="True" w3468 {
              tunnel: [Elevator_Command."Going Up" ("element") Elevator_Command."Going Down" ("element")] -> w3466
              frame True {
              }
              frame False {
              }
            }
            n1731 = Enqueue Element(queue=w3495, element=w3466, error in (no error)=w3494) -> (queue out=w3493:refnum<queue>, error out=w3492:errorcluster)  [unwired: 1 in, 1 out]
            n1732 = Equal?(x=w3462, y=w3461) -> (x = y?=w3458:bool)
            n1733 = And(x=w3458, y=w3460) -> (x .and. y?=w3459:bool)
            n1734 = case shown="False" w3459 {
              tunnel: w3493 -> [w3498 w3503]
              tunnel: w3492 -> [w3497 w3502]
              tunnel: [w3498 w3500] -> w3473
              tunnel: [w3497 w3499] -> w3472
              frame True {
              }
              frame False {
                n1735 = Enqueue Element(queue=w3503, element=Elevator_Command."Short Delay", error in (no error)=w3502) -> (queue out=w3500:refnum<queue>, error out=w3499:errorcluster)  [unwired: 1 in, 1 out]
              }
            }
            n1736 = Enqueue Element(queue=w3473, element=Elevator_Command."Unpress Button", error in (no error)=w3472) -> (queue out=w3471:refnum<queue>, error out=w3470:errorcluster)  [unwired: 1 in, 1 out]
            n1737 = Enqueue Element(queue=w3471, element=Elevator_Command."Open Doors", error in (no error)=w3470) -> (queue out=w3490:refnum<queue>, error out=w3491:errorcluster)  [unwired: 1 in, 1 out]
            n1738 = local write "Elevator Automate"(w3484) -> ()
            n1739 = Enqueue Element(queue=w3490, element=Elevator_Command."Long Delay", error in (no error)=w3491) -> (queue out=w3489:refnum<queue>, error out=w3488:errorcluster)  [unwired: 1 in, 1 out]
            n1740 = Wait (ms)(milliseconds to wait=u32 1) -> ()  [unwired: 1 out]
            n1741 = Enqueue Element(queue=w3489, element=Elevator_Command."Close Doors", error in (no error)=w3488) -> (queue out=w3483:refnum<queue>, error out=w3482:errorcluster)  [unwired: 1 in, 1 out]
            n1742 = Enqueue Element(queue=w3483, element=Elevator_Command."Idle", error in (no error)=w3482) -> (queue out=w3457:refnum<queue>, error out=w3496:errorcluster)  [unwired: 1 in, 1 out]
          }
        }
      }
    }
    n1743 = Wait (ms)(milliseconds to wait=w3442) -> ()  [unwired: 1 out]
    n1744 = local read "STOP"() -> (w3444:bool)
  }
  n1745 = while {
    tunnel: w2 -> [_]
    tunnel: w1 -> [_]
    shift-right: [w3508] -> _
    shift-left: TRUE -> [w3507]
    stop <- w3509 stop-if-true
    n1746 = flat-sequence {
      tunnel: [w3519] -> w3508
      tunnel: w3507 -> [w3533]
      frame #0 {
        # "Если лифт между этажами едет наверх,\nприравниваем позицию лифта к этажу, что ниже текущего положения.\nЕсли лифт едет между этажами вниз, то приравниваем позицию лифта к этажу, что выше текущего положения"
        # "Информационное табло лифта для пассажиров"
        n1747 = local read "Elevator Automate"() -> (w3529:T2)
        n1748 = Unbundle By Name(w3529) -> ("Elevator Status"=w3514:T6)
        n1749 = local read "Elevator Panel"() -> (w3532:T3)
        n1750 = Equal?(x=w3514, y=T6."Going Up") -> (x = y?=w3528:bool)
        n1751 = Unbundle By Name(w3532) -> ("Emergency"=w3531:bool)
        n1752 = case shown="False" w3531 {
          tunnel: ["" ("string") w3582] -> w3522
          frame False {
          }
          frame True {
            n1753 = Concatenate Strings("\r\n", "*Вызов оператора*" ("string")) -> (w3582:string)
          }
        }
        n1754 = Equal?(x=w3514, y=T6."Stand By") -> (x = y?=w3513:bool)
        n1755 = Equal?(x=w3514, y=T6."Stop") -> (x = y?=w3512:bool)
        n1756 = Equal?(x=w3514, y=T6."Cancel") -> (x = y?=w3511:bool)
        n1757 = Compound Arithmetic op=OR(w3513, w3512, w3511) -> (w3510:bool)
        n1758 = case shown="False" w3510 {
          tunnel: w3528 -> [w3539 _]
          tunnel: [w3539 w3540] -> w3519
          tunnel: w3533 -> [_ w3540]
          frame False {
          }
          frame True {
          }
        }
        n1759 = case shown="True" w3519 {
          tunnel: [w3541 w3563] -> w3530
          frame False {
            n1760 = local read "Floors Schematic"() -> (w3544:T4)
            n1761 = control-ref of="Elevator Cabin"() -> (w3545:refnum<vi>)
            n1762 = property class="Slide (strict)"(reference=w3545) -> ("Top"=w3542:i32)  [unwired: 1 in, 2 out]
            n1763 = Unbundle By Name(w3544) -> ("Floor Position"=w3543:i16[])
            n1764 = while {
              tunnel: w3543 -> [w3555]
              tunnel: w3542 -> [w3553]
              tunnel: [w3552] -> w3541
              i -> [w3550]
              stop <- w3551 stop-if-true
              w3548 = T8 12 items=["Floor Length"=48, "Sum of Floors"=12, "Floor Step in ms"=63, "Elevator Door Step in ms"=30, "Global Wait in ms"=20, "Event Wait in ms"=100] ("Elevator Constants")
              n1765 = To Long Integer(number=w3548) -> (32bit integer=w3549:i32)
              n1766 = Subtract(x=w3549, y=w3550) -> (x-y=w3547:i32)
              n1767 = Decrement(x=w3547) -> (x-1=w3546:i32)
              n1768 = Index Array(array=w3555, index=w3546) -> (element=w3556:i16)
              n1769 = To Long Integer(number=w3556) -> (32bit integer=w3554:i32)
              n1770 = Equal?(x=w3553, y=w3554) -> (x = y?=w3557:bool)
              n1771 = Greater Or Equal?(x=w3554, y=w3553) -> (x >= y?=w3551:bool)
              n1772 = case shown="False" w3557 {
                tunnel: w3546 -> [w3560 w3562]
                tunnel: [w3558 w3561] -> w3552
                frame False {
                  n1773 = Increment(x=w3560) -> (x+1=w3559:i32)
                  n1774 = Increment(x=w3559) -> (x+1=w3558:i32)
                }
                frame True {
                  n1775 = Increment(x=w3562) -> (x+1=w3561:i32)
                }
              }
            }
          }
          frame True {
            n1776 = local read "Floors Schematic"() -> (w3566:T4)
            n1777 = control-ref of="Elevator Cabin"() -> (w3567:refnum<vi>)
            n1778 = property class="Slide (strict)"(reference=w3567) -> ("Top"=w3564:i32)  [unwired: 1 in, 2 out]
            n1779 = Unbundle By Name(w3566) -> ("Floor Position"=w3565:i16[])
            n1780 = while {
              tunnel: w3565 -> [w3573]
              tunnel: w3564 -> [w3571]
              tunnel: [w3570] -> w3563
              i -> [w3568]
              stop <- w3569 stop-if-true
              n1781 = Index Array(array=w3573, index=w3568) -> (element=w3574:i16)
              n1782 = To Long Integer(number=w3574) -> (32bit integer=w3572:i32)
              n1783 = Equal?(x=w3571, y=w3572) -> (x = y?=w3575:bool)
              n1784 = Less Or Equal?(x=w3572, y=w3571) -> (x <= y?=w3569:bool)
              n1785 = case shown="False" w3575 {
                tunnel: w3568 -> [w3576 w3578]
                tunnel: [w3576 w3577] -> w3570
                frame False {
                }
                frame True {
                  n1786 = Increment(x=w3578) -> (x+1=w3577:i32)
                }
              }
            }
          }
        }
        n1787 = Number To Decimal String(number=w3530) -> (decimal integer string=w3523:string)  [unwired: 1 in]
        n1788 = control-ref of="Elevator Cabin"() -> (w3527:refnum<vi>)
        n1789 = case shown="False" w3510 {
          tunnel: [w3535 "Остановка" ("string")] -> w3520
          tunnel: w3519 -> [w3534 _]
          frame False {
            n1790 = Select(t="Движение вверх " ("string"), s=w3534, f="Движение вниз " ("string")) -> (s? t:f=w3535:string)
          }
          frame True {
          }
        }
        n1791 = Concatenate Strings("Этаж " ("string"), w3523, "\r\n", w3520, w3522) -> (w3525:string)
        n1792 = property class="Slide (strict)"(reference=w3527) -> ("Top"=→"Position:Top":i32)  [unwired: 1 in, 2 out]
        n1793 = local write "Passenger Information Board"(w3525) -> ()
      }
    }
    n1794 = local read "Global Wait in ms"() -> (w3506:u32)
    n1795 = Wait (ms)(milliseconds to wait=w3506) -> ()  [unwired: 1 out]
    n1796 = local read "STOP"() -> (w3509:bool)
  }
  n1797 = Release Queue(queue=w11, force destroy? (F)=TRUE, error in (no error)=w10) -> ()  [unwired: 3 out]
  n1798 = Release Queue(queue=w14, force destroy? (F)=TRUE, error in (no error)=w15) -> ()  [unwired: 3 out]
